vi "Main.vi"() -> ()   [LabVIEW 2015, in "Tool Module.lvlib"]
doc: "This template is based from the Queued Message Handler design pattern and the Queued Message Handler Project Template that ships with LabVIEW 2014.\n\nThe main difference is that the Queue is private to this module and communication between modules is done via Broadcast and Request events.\n\nRequest events are wrapped via public API methods and are handled in the Event handler loop in this VI.\nAny module can register for Broadcast events sent by this module.\n\nThe Event Handling Loop generates messages based on user interface actions.\n\nThe Message Handling Loop processes messages generated by the Event Handling Loop, or by other messages. The messages are string values, so new messages can be added easily to the Message Cases case structure in the Message Handling Loop. Each message cluster can also provide an optional value for Message Data, which is a variant that can be converted to whatever message-specific data is required.\n_____\nBased on Delacor QMH Project Template 2.1.0.2."
uses:
  Tool Module.lvlib
  <vilib>/Delacor/Delacor QMH/Libraries/Module Admin_class/Delacor_lib_QMH_Module Admin.lvclass
  Module Data--cluster.ctl
  Support/_STATUS Typedef--cluster.ctl
  Support/Timer State Return Typedef.ctl
  Support/_Sample Data Rtn Cluster--typedef.ctl
  Support/_Inspection Limits cluster--typedef.ctl
  Event Logger Library/Event Log/EventLog.lvclass
  Return FPGA Setup Data (Reply Payload)--cluster.ctl
  Tool Typedefs/_FPGA Setup Params Cluster--typedef.ctl
  Tool Typedefs/_FPGA Timing Constraints Cluster--typedef.ctl
  Tool Typedefs/_FPGA Timing Ctrl Cluster--typedef.ctl
  Tool Typedefs/_FPGA Laser Config Cluster--typedef.ctl
  Tool Typedefs/_FPGA Peak Proc Cfg Cluster--typedef.ctl
  Tool Typedefs/_FPGA SPI Cfg Cluster--typedef.ctl
  Tool Interface/_Host - HS Data Stream State Enum Typedef.ctl
  _Motion Status Reader SM enum--typedef.ctl
  Tool Typedefs/_Motion STATUS Cluster--typedef.ctl
  Support/_IHL Data Cluster--typedef.ctl
  Support/_IHL SM Enum--typedef.ctl
  Support/_IHL Status Update Cluster--typedef.ctl
  Support/_IHL Status Notifier Data Cluster--typedef.ctl
  Support/_HS Data Stream Params Cluster--typedef.ctl
  Support/_HS Data Stream SM enum--typedef.ctl
  <vilib>/Delacor/Delacor QMH/Libraries/Message Queue_class/Delacor_lib_QMH_Message Queue.lvclass/Delacor_lib_QMH_Message Queue.ctl
  Start Inspect 2 (Reply Payload)--cluster.ctl
  Get All Inspect Data (Reply Payload)--cluster.ctl
  Stop Argument--cluster.ctl
  <vilib>/Delacor/Delacor QMH/Libraries/Module Admin_class/Delacor_lib_QMH_Module Admin.lvclass/Delacor_lib_QMH_Module Admin.ctl
  CONNECT Argument--cluster.ctl
  GOTO Argument--cluster.ctl
  Support/_GoTo Cmd Typedef--enum.ctl
  Get All Inspect Data Argument--cluster.ctl
  Start Data Monitor Argument--cluster.ctl
  Get FPGA Setup Params Argument--cluster.ctl
  Get FPGA Setup Params (Reply Payload)--cluster.ctl
  Set FPGA Setup Params Argument--cluster.ctl
  Commit Tool Config Argument--cluster.ctl
  Tool Config/_Configuration Cluster_v3--typedef.ctl
  Tool Config/_Tool Block Cluster_v3--typedef.ctl
  Tool Config/_Motor Block Cluster_v2--typedef.ctl
  Tool Config/_Verification Blk Cluster--typedef.ctl
  Tool Config/_ProbeConfigParams Cluster--typedef.ctl
  Tool Config/_Sensor Block Cluster--typedef.ctl
  Tool Config/_SensorConfigParams Cluster--typedef.ctl
  Set Integration Count Argument--cluster.ctl
  Set Laser Params Argument--cluster.ctl
  Get Mtrl Ctrl Reg Argument--cluster.ctl
  Get Mtrl Ctrl Reg (Reply Payload)--cluster.ctl
  Commit Ctrl Reg Argument--cluster.ctl
  Set Event Logger Argument--cluster.ctl
  Write to File Argument--cluster.ctl
  Read from File Argument--cluster.ctl
  Set Device Temp Thresholds Argument--cluster.ctl
  Tool Typedefs/_Temperature Threshold Arrays--typedef.ctl
  Get Cycle Count Argument--cluster.ctl
  Get Cycle Count (Reply Payload)--cluster.ctl
  Return FPGA Setup Data Argument--cluster.ctl
  Update FPGA Setup Data Argument--cluster.ctl
  Get-Set Inspection Limits Argument--cluster.ctl
  Get-Set Inspection Limits (Reply Payload)--cluster.ctl
  Support/_Tool Status Update Cluster--typedef.ctl
  Connected Argument--cluster.ctl
  Read from File Rtn Argument--cluster.ctl
  Support/_Cycle Count File Cluster--typedef.ctl
  Tool Typedefs/_Temperature All Arrays--typedef.ctl
  Tool Typedefs/_FPGA Return Setup Data Cluster--typedef.ctl
  Tool Config/_Tool Cfg Return Parameters Cluster--typedef.ctl
  Tool Typedefs/_Data Stream Fmt Params Cluster--typedef.ctl
  <vilib>/Delacor/Delacor QMH/Libraries/Message Queue_class/Delacor_lib_QMH_Enqueue Message (Single).vi
  <vilib>/Delacor/Delacor QMH/Libraries/Module Admin_class/Delacor_lib_QMH_Get External Launch.vi
  <vilib>/Delacor/Delacor QMH/Libraries/Message Queue_class/Delacor_lib_QMH_Enqueue Message (Array).vi
  Tool Interface/GLOB - Configuration Options.vi
  Support/ToolModGLOB.vi
  <vilib>/Utility/error.llb/Error Cluster From Error Code.vi
  <vilib>/ErrorRing/Error Ring.xnode
  <vilib>/Delacor/Delacor QMH/Libraries/Message Queue_class/Delacor_lib_QMH_Message Queue.lvclass
  Collect Data Mgr/Collect Data Mgr.lvlib
  Tool Interface/Tool Interface.lvlib
  Tool Config/Tool Cfg.lvlib
panel:
  in  "Retrieve Cfg":bool
  in  "Cfg File Path":path
  in  "Simulate MHL Error":bool
  in  "Simulate EHL Error":bool
  out "error out":errorcluster
  in  "Module Admin":refnum<class "Delacor_lib_QMH_Module Admin.lvclass">
  out "Status":string
  # "Other QMH Modules communicate with this Module via its Public API (wrappers for its Request Events).\n\nThis Module communicates with other Modules via its Broadcast Events.\nAny module that wants to get these messages, just registers for this module's Broadcast events."
  # "This template is for the Delacor Modified Queued Message Handler design pattern.\n\nSee the block diagram for more information on how to use this template."
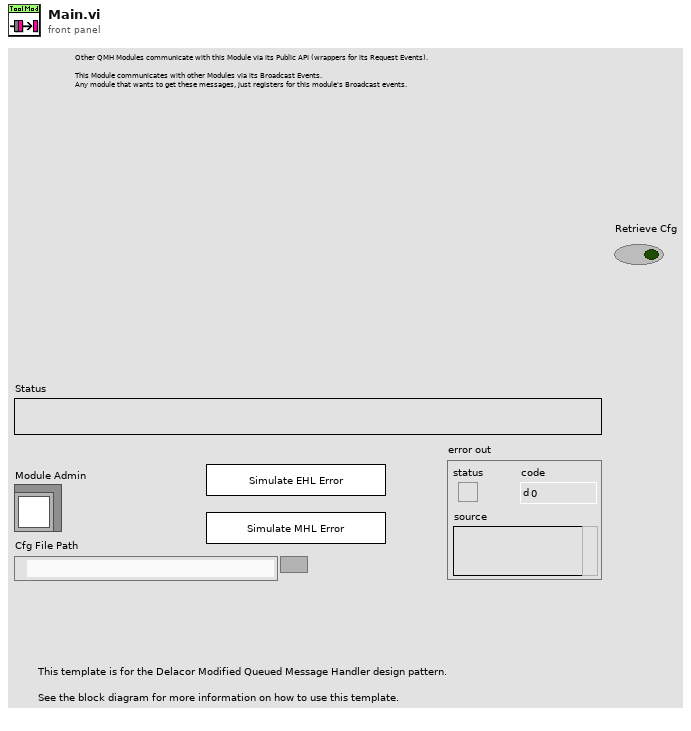
[diagram p1: front panel]
types:
  T1 = typedef "Tool Module.lvlib/_IHL Status Notifier Data Cluster--typedef.ctl" = cluster{"Status":u16, "Encoder":i32}
  T2 = typedef "Tool Module.lvlib/_IHL Data Cluster--typedef.ctl" = cluster{"IHL State":T3, "Timeout":i32, "Loop Count":i32, "Start Sample No.":u32, "Collecting Data":bool, "No. Samples":i32, "Success Flag":bool, "Inspect Status ":T4, "Status":u16, "Encoder Count":i32, "PosToStartScan":i32, "ScanLength":i32, "MaxSamples":i32, "PosToEndScan":i32, "Host SampleData":refnum<notifier>, "data value reference":refnum<data-value>, "Block Cnt notifier out":refnum<notifier>, "EventLog":refnum<class "EventLog.lvclass">}
  T3 = typedef "Tool Module.lvlib/_IHL SM Enum--typedef.ctl" = enum16{"Init", "Set Motion Speed", "Move To Scan Start", "Wait for Motion Out", "Wait for Start Pos", "Inspect: START", "Wait for Motion IN", "Wait for Inspect Range", "Inspecting", "Inspect: STOP"}
  T4 = typedef "Tool Module.lvlib/_IHL Status Update Cluster--typedef.ctl" = cluster{"Ready":bool, "Inspecting":bool, "Cancel":bool}
  T5 = typedef "_Motion STATUS Cluster--typedef.ctl" = cluster{"Encoder":i32, "STATUS":u16, "MC SM State":u16, "M_Ctrl":u16}
  T6 = typedef "Tool Module.lvlib/_Motion Status Reader SM enum--typedef.ctl" = enum16{"Not Connected", "Connect", "Idle", "Receive Data", "Disconnect"}
  T7 = typedef "Tool Module.lvlib/_Host - HS Data Stream State Enum Typedef.ctl" = enum16{"Idle", "Connect", "Receive Data", "Close Connection"}
  T8 = typedef "Tool Module.lvlib/Module Data--cluster.ctl" = cluster{"Status String":string, "STATUS":T9, "Timer 1":T10, "Timer 2":T10, "Timer 1 Call State":string, "Timer 2 Call State":string, "LED State 1":bool, "LED State 2":bool, "OK to Connect":bool, "Connecting":bool, "Got FW Ver":bool, "Got Tool Type":bool, "Got Tool Cfg":bool, "Got Fmt Params":bool, "Got FPGA Setup":bool, "Got Cycle Count":bool, "Cancel Inspect":bool, "Trig State":bool, "Encoder Count":i32, "Loop Counter":i32, "Start Sample No.":u32, "Host SampleData":refnum<notifier>, "Inspection Limits":T11, "EventLog.lvclass":refnum<class "EventLog.lvclass">, "Prev. Encdr":i32, "Status Update Cnt":i32, "Cycle Count":i32, "data value reference":refnum<data-value>, "Final No. of Blks":i32, "CD Success":bool, "FW Ver Maj/Min":dbl, "FPGA Setup Reply Notifier":refnum<notifier>}
  T9 = typedef "Tool Module.lvlib/_STATUS Typedef--cluster.ctl" = cluster{"Initialized":bool, "Connected":bool, "Ready":bool, "Inspecting":bool, "Position":dbl, "Status":u16, "Error":bool, "Code":i32, "MC SM State":u16, "M_Ctrl":u16}
  T10 = typedef "Tool Module.lvlib/Timer State Return Typedef.ctl" = cluster{"Instance Name":string, "On/Off":bool, "Running":bool}
  T11 = typedef "Tool Module.lvlib/_Inspection Limits cluster--typedef.ctl" = cluster{"MaxSamples":i32, "PosToStartScan":i32, "PosToEndScan":i32, "ScanLength":i32}
  T12 = typedef "Tool Module.lvlib/Request Events--cluster.ctl" = cluster{"Stop Module":refnum<user-event>, "Show Panel":refnum<user-event>, "Hide Panel":refnum<user-event>, "Get Module Execution Status":refnum<user-event>, "Show Diagram":refnum<user-event>, "GOTO":refnum<user-event>, "CONNECT":refnum<user-event>, "Get All Inspect Data":refnum<user-event>, "Start Data Monitor":refnum<user-event>, "Get FPGA Setup Params":refnum<user-event>, "Set FPGA Setup Params":refnum<user-event>, "Commit Tool Config":refnum<user-event>, "Set Integration Count":refnum<user-event>, "Set Laser Params":refnum<user-event>, "Get Mtrl Ctrl Reg":refnum<user-event>, "Commit Ctrl Reg":refnum<user-event>, "Set Event Logger":refnum<user-event>, "Write to File":refnum<user-event>, "Read from File":refnum<user-event>, "Set Device Temp Thresholds":refnum<user-event>, "Get Cycle Count":refnum<user-event>, "Return FPGA Setup Data":refnum<user-event>, "Update FPGA Setup Data":refnum<user-event>, "Setup Timer":refnum<user-event>, "Tool Status Reader Cmd":refnum<user-event>, "Stop Helper Loops":refnum<user-event>, "Enable Receive Stream":refnum<user-event>, "Get-Set Inspection Limits":refnum<user-event>, "Start Inspect 2":refnum<user-event>}
  T13 = typedef "Tool Module.lvlib/_Loop Ctrl Notifiers Cluster--typedef.ctl" = cluster{"Raw Stream Ctrl":refnum<notifier>}
  T14 = typedef "Tool Module.lvlib/Broadcast Events--cluster.ctl" = cluster{"Module Did Init":refnum<user-event>, "Status Updated":refnum<user-event>, "Error Reported":refnum<user-event>, "Module Did Stop":refnum<user-event>, "Update Module Execution Status":refnum<user-event>, "Send Status":refnum<user-event>, "Trigger":refnum<user-event>, "Connected":refnum<user-event>, "Read from File Rtn":refnum<user-event>, "Device Temperature":refnum<user-event>, "Time Expired":refnum<user-event>}
  T15 = typedef "Tool Module.lvlib/_HS Data Stream SM enum--typedef.ctl" = enum16{"Idle", "Receive HS Data", "Close Connection"}
  T16 = typedef "Tool Module.lvlib/_HS Data Stream Params Cluster--typedef.ctl" = cluster{"Raw Data Stream Loop cmd":T15, "Data Array DVR ref":refnum<data-value>, "HS Sample Data notifier":refnum<notifier>, "Block Count Notifier":refnum<notifier>}
  T17 = typedef "Tool Module.lvlib/Start Inspect 2 (Reply Payload)--cluster.ctl" = cluster{"Sample Data notifier":refnum<notifier>, "Start Inspect 2_error":errorcluster}
  T18 = typedef "Tool Module.lvlib/Get All Inspect Data (Reply Payload)--cluster.ctl" = cluster{"Success":bool, "Full Inspection Data":u32[][], "data value reference":refnum<data-value>}
  T19 = enum32{"invalid lock state", "Not Locked", "Locked (No Password)", "Password-protected"}
  T20 = typedef "Tool Module.lvlib/Stop Argument--cluster.ctl" = cluster{"Origin":string, "Exit via Stop Module Req?":bool, "Wait for Module to stop?":bool}
  T21 = typedef "Tool Module.lvlib/CONNECT Argument--cluster.ctl" = cluster{"Connect":bool}
  T22 = typedef "Tool Module.lvlib/GOTO Argument--cluster.ctl" = cluster{"GoTo Cmd":T23, "Data":i32}
  T23 = typedef "Tool Module.lvlib/_GoTo Cmd Typedef--enum.ctl" = enum16{"MoveA", "MoveR", "Home Position", "Home None", "Cleaning Position"}
  T24 = typedef "Tool Module.lvlib/Get All Inspect Data Argument--cluster.ctl" = cluster{"dummy":bool, "Wait Notifier":refnum<notifier>}
  T25 = typedef "Tool Module.lvlib/Start Data Monitor Argument--cluster.ctl" = cluster{"Monitor":bool, "Lasers ON?":bool, "Host Sample Data notifier":refnum<notifier>}
  T26 = typedef "Tool Module.lvlib/Get FPGA Setup Params Argument--cluster.ctl" = cluster{"dummy":bool, "Wait Notifier":refnum<notifier>}
  T27 = typedef "Tool Module.lvlib/Set FPGA Setup Params Argument--cluster.ctl" = cluster{"Commit":bool, "FPGA Setup Parameters":T28}
  T28 = typedef "_FPGA Setup Params Cluster--typedef.ctl" = cluster{"FPGA Timing Constraints":T29, "FPGA Timing Ctrl":T30, "FPGA Laser Config":T31, "FPGA Peak Proc Cfg":T32, "FPGA SPI Cfg":T33}
  T29 = typedef "_FPGA Timing Constraints Cluster--typedef.ctl" = cluster{"frame.length Min":u16, "frame.ST_OFF Min":u16, "frame.ST_ON Min":u16, "frame.first data idx":u16, "frame.integ Offset":u16, "frame.integ Delay":u16, "frame.ad_latch Delay":u16, "frame.trig time Max":u32}
  T30 = typedef "_FPGA Timing Ctrl Cluster--typedef.ctl" = cluster{"trig.time":u32, "integ.count 1":u32, "integ.count 2":u32, "encdr.latch ctrl":u32, "pixel.read count":u16, "clock.select":u16, "ad.clock offset":u16, "data.control reg":u16}
  T31 = typedef "_FPGA Laser Config Cluster--typedef.ctl" = cluster{"laser.gain":i16, "laser.threshold Low":u16, "laser.threshold High":u16, "laser.dac init":u16, "laser.dac Min":u16, "laser.dac Max":u16, "laser.config reg":u16}
  T32 = typedef "_FPGA Peak Proc Cfg Cluster--typedef.ctl" = cluster{"PD.threshold":u16, "PD.width detect Min":u8, "PD.sensor pixels":u16, "PD.config reg":u16}
  T33 = typedef "_FPGA SPI Cfg Cluster--typedef.ctl" = cluster{"SPI Divide Value":u8, "SPI config reg":u16}
  T34 = typedef "Tool Module.lvlib/Commit Tool Config Argument--cluster.ctl" = cluster{"Tool Config Cluster":T35}
  T35 = typedef "Tool Cfg.lvlib/_Configuration Cluster_v3--typedef.ctl" = cluster{"Tool Type":u16, "Tool SN":u16, "Tool Block":T36, "Motor Block":T37, "Verification Block":T38, "Probe Block":cluster{"nProbes":u16, "Probe Param Array":T39[]}}
  T36 = typedef "Tool Cfg.lvlib/_Tool Block Cluster_v3--typedef.ctl" = cluster{"Encoder Size":u16, "Encoder Scale":u32, "Encoder Offset":i32, "MaxEncoder":i32, "MinEncoder":i32, "Start Delay":sgl, "Tool Face Ref":sgl}
  T37 = typedef "Tool Cfg.lvlib/_Motor Block Cluster_v2--typedef.ctl" = cluster{"MinMotor Speed":u16, "MaxMotor Speed":u16, "Homing Speed":u16, "Jog Speed":u16, "Inspect Speed":u16, "VBlk Speed":u16, "CleaningPos":i32, "Safe Zone":i32, "Has Motor":bool, "Use Home Index":bool}
  T38 = typedef "Tool Cfg.lvlib/_Verification Blk Cluster--typedef.ctl" = cluster{"Angle":sgl, "FlankLength1":sgl, "FlankLength2":sgl, "Location":sgl, "Serial Number":u16}
  T39 = typedef "Tool Cfg.lvlib/_ProbeConfigParams Cluster--typedef.ctl" = cluster{"Name":string, "Laser Init Pwr":u16, "Laser Gain":u8, "Integ Count":u16, "Meas. Range":sgl, "Angle":sgl, "Probe Offset":sgl, "Sensor Block":T40}
  T40 = typedef "Tool Cfg.lvlib/_Sensor Block Cluster--typedef.ctl" = cluster{"nSensors":u16, "SensorCfgParams Array":T41[]}
  T41 = typedef "Tool Cfg.lvlib/_SensorConfigParams Cluster--typedef.ctl" = cluster{"Total Pixels":u16, "Positive  Peaks":bool, "CalibrCoefArray":dbl[], "Start Idx":u16, "End Idx":u16}
  T42 = typedef "Tool Module.lvlib/Set Integration Count Argument--cluster.ctl" = cluster{"Mode":i16, "Integ Count":u32}
  T43 = typedef "Tool Module.lvlib/Set Laser Params Argument--cluster.ctl" = cluster{"Mode":i16, "Gain":u16, "Init DAC":u16}
  T44 = typedef "Tool Module.lvlib/Get Mtrl Ctrl Reg Argument--cluster.ctl" = cluster{"dummy":bool, "Wait Notifier":refnum<notifier>}
  T45 = typedef "Tool Module.lvlib/Commit Ctrl Reg Argument--cluster.ctl" = cluster{"Ctrl Reg":u16}
  T46 = typedef "Tool Module.lvlib/Set Event Logger Argument--cluster.ctl" = cluster{"EventLog.lvclass":refnum<class "EventLog.lvclass">}
  T47 = typedef "Tool Module.lvlib/Write to File Argument--cluster.ctl" = cluster{"Filename":string, "Flattened data strings":string[]}
  T48 = typedef "Tool Module.lvlib/Read from File Argument--cluster.ctl" = cluster{"Filename":string, "Create?":bool, "Flattened Data Strings":string[]}
  T49 = typedef "Tool Module.lvlib/Set Device Temp Thresholds Argument--cluster.ctl" = cluster{"Device Temp Thold Arrays":T50}
  T50 = typedef "_Temperature Threshold Arrays--typedef.ctl" = cluster{"High Thold ":dbl[], "Low Thold ":dbl[]}
  T51 = typedef "Tool Module.lvlib/Get Cycle Count Argument--cluster.ctl" = cluster{"Clear?":bool, "Wait Notifier":refnum<notifier>}
  T52 = typedef "Tool Module.lvlib/Return FPGA Setup Data Argument--cluster.ctl" = cluster{"Reload":bool, "Wait Notifier":refnum<notifier>, "wait for reply":bool}
  T53 = typedef "Tool Module.lvlib/Update FPGA Setup Data Argument--cluster.ctl" = cluster{"Commit":bool, "FPGA Setup Parameters":T28}
  T54 = typedef "Tool Module.lvlib/Get-Set Inspection Limits Argument--cluster.ctl" = cluster{"Set":bool, "Inspection Limits":T11, "Wait Notifier":refnum<notifier>, "wait for reply":bool}
  T55 = enum32{"Invalid", "Standard", "Closed", "Hidden", "Minimized", "Maximized"}
  T56 = typedef "Tool Module.lvlib/_Tool Status Update Cluster--typedef.ctl" = cluster{"Tool Status":T5, "Reader SM State":T6}
  T57 = cluster{"TE_Running":bool, "PD_Running":bool, "Laser On 1":bool, "Laser On 2":bool}
  T58 = typedef "Tool Module.lvlib/Connected Argument--cluster.ctl" = cluster{"Connected":bool, "Tool Type":u16, "Tool SN":u16}
  T59 = typedef "Tool Module.lvlib/Get Mtrl Ctrl Reg (Reply Payload)--cluster.ctl" = cluster{"Mtr Ctrl Reg":u16, "Get Mtrl Ctrl Reg_error":errorcluster}
  T60 = typedef "Tool Module.lvlib/Get-Set Inspection Limits (Reply Payload)--cluster.ctl" = cluster{"Inspection Limits":T11, "Get-Set Inspection Limits_error":errorcluster}
  T61 = typedef "Tool Module.lvlib/Get FPGA Setup Params (Reply Payload)--cluster.ctl" = cluster{"Version String":string, "FPGA Setup Parameters":T28}
  T62 = typedef "Tool Module.lvlib/Read from File Rtn Argument--cluster.ctl" = cluster{"Filename":string, "XML Strings":string[], "Error Status":errorcluster}
  T63 = typedef "Tool Module.lvlib/_Cycle Count File Cluster--typedef.ctl" = cluster{"Cycle Count":i32}
  T64 = cluster{"Filename":string, "XML Strings":string, "Error Status":errorcluster}
  T65 = typedef "_Temperature All Arrays--typedef.ctl" = cluster{"Temp Sensors":dbl[], "High Thold ":dbl[], "Low Thold ":dbl[]}
  T66 = typedef "Tool Module.lvlib/Get Cycle Count (Reply Payload)--cluster.ctl" = cluster{"Cycle Count":i32, "Get Cycle Count_error":errorcluster}
  T67 = typedef "Tool Module.lvlib/Return FPGA Setup Data (Reply Payload)--cluster.ctl" = cluster{"Version String":string, "FPGA Setup Parameters":T28, "Return FPGA Setup Data_error":errorcluster}
  T68 = typedef "_FPGA Return Setup Data Cluster--typedef.ctl" = cluster{"Version String":string, "Mtr Ctrl Reg":u16, "FPGA Setup Parameters":T28}
  T69 = typedef "Tool Cfg.lvlib/_Tool Cfg Return Parameters Cluster--typedef.ctl" = cluster{"Config Cluster Version":string, "Product Name":string, "Tool Config Cluster":T35}
  T70 = typedef "_Data Stream Fmt Params Cluster--typedef.ctl" = cluster{"Samples per Block":i32, "Raw Data Status Len":i32, "Fltr Data Status Len":i32}
  T71 = typedef "Tool Module.lvlib/_Sample Data Rtn Cluster--typedef.ctl" = cluster{"Inspecting":bool, "Acquiring Data":bool, "Success":bool, "Cancelled":bool, "Scan Data Array":u32[], "error cluster":errorcluster}
  T72 = typedef "Tool Cfg.lvlib/_Tool Operation Config Cluster--typedef.ctl" = cluster{"Use Tool Cfg":bool, "Use Tool Cal":bool, "Fake Data?":bool, "Mode":i16, "Array Subset Length":i16, "nArrays to Read":i16, "Full Array Read Length":i16, "nSubarrays/Sensor":i16}
  T73 = typedef "Collect Data Mgr.lvlib/Start Collect (Reply Payload)--cluster.ctl" = cluster{"Success":bool, "CD_Status":u8}
  T74 = typedef "Tool Module.lvlib/_Data Notifiers Cluster--typedef.ctl" = cluster{"Sample Data":refnum<notifier>}
  T75 = cluster{"Tool Status Cluster":T5, "Tool Status Reader State":T6}
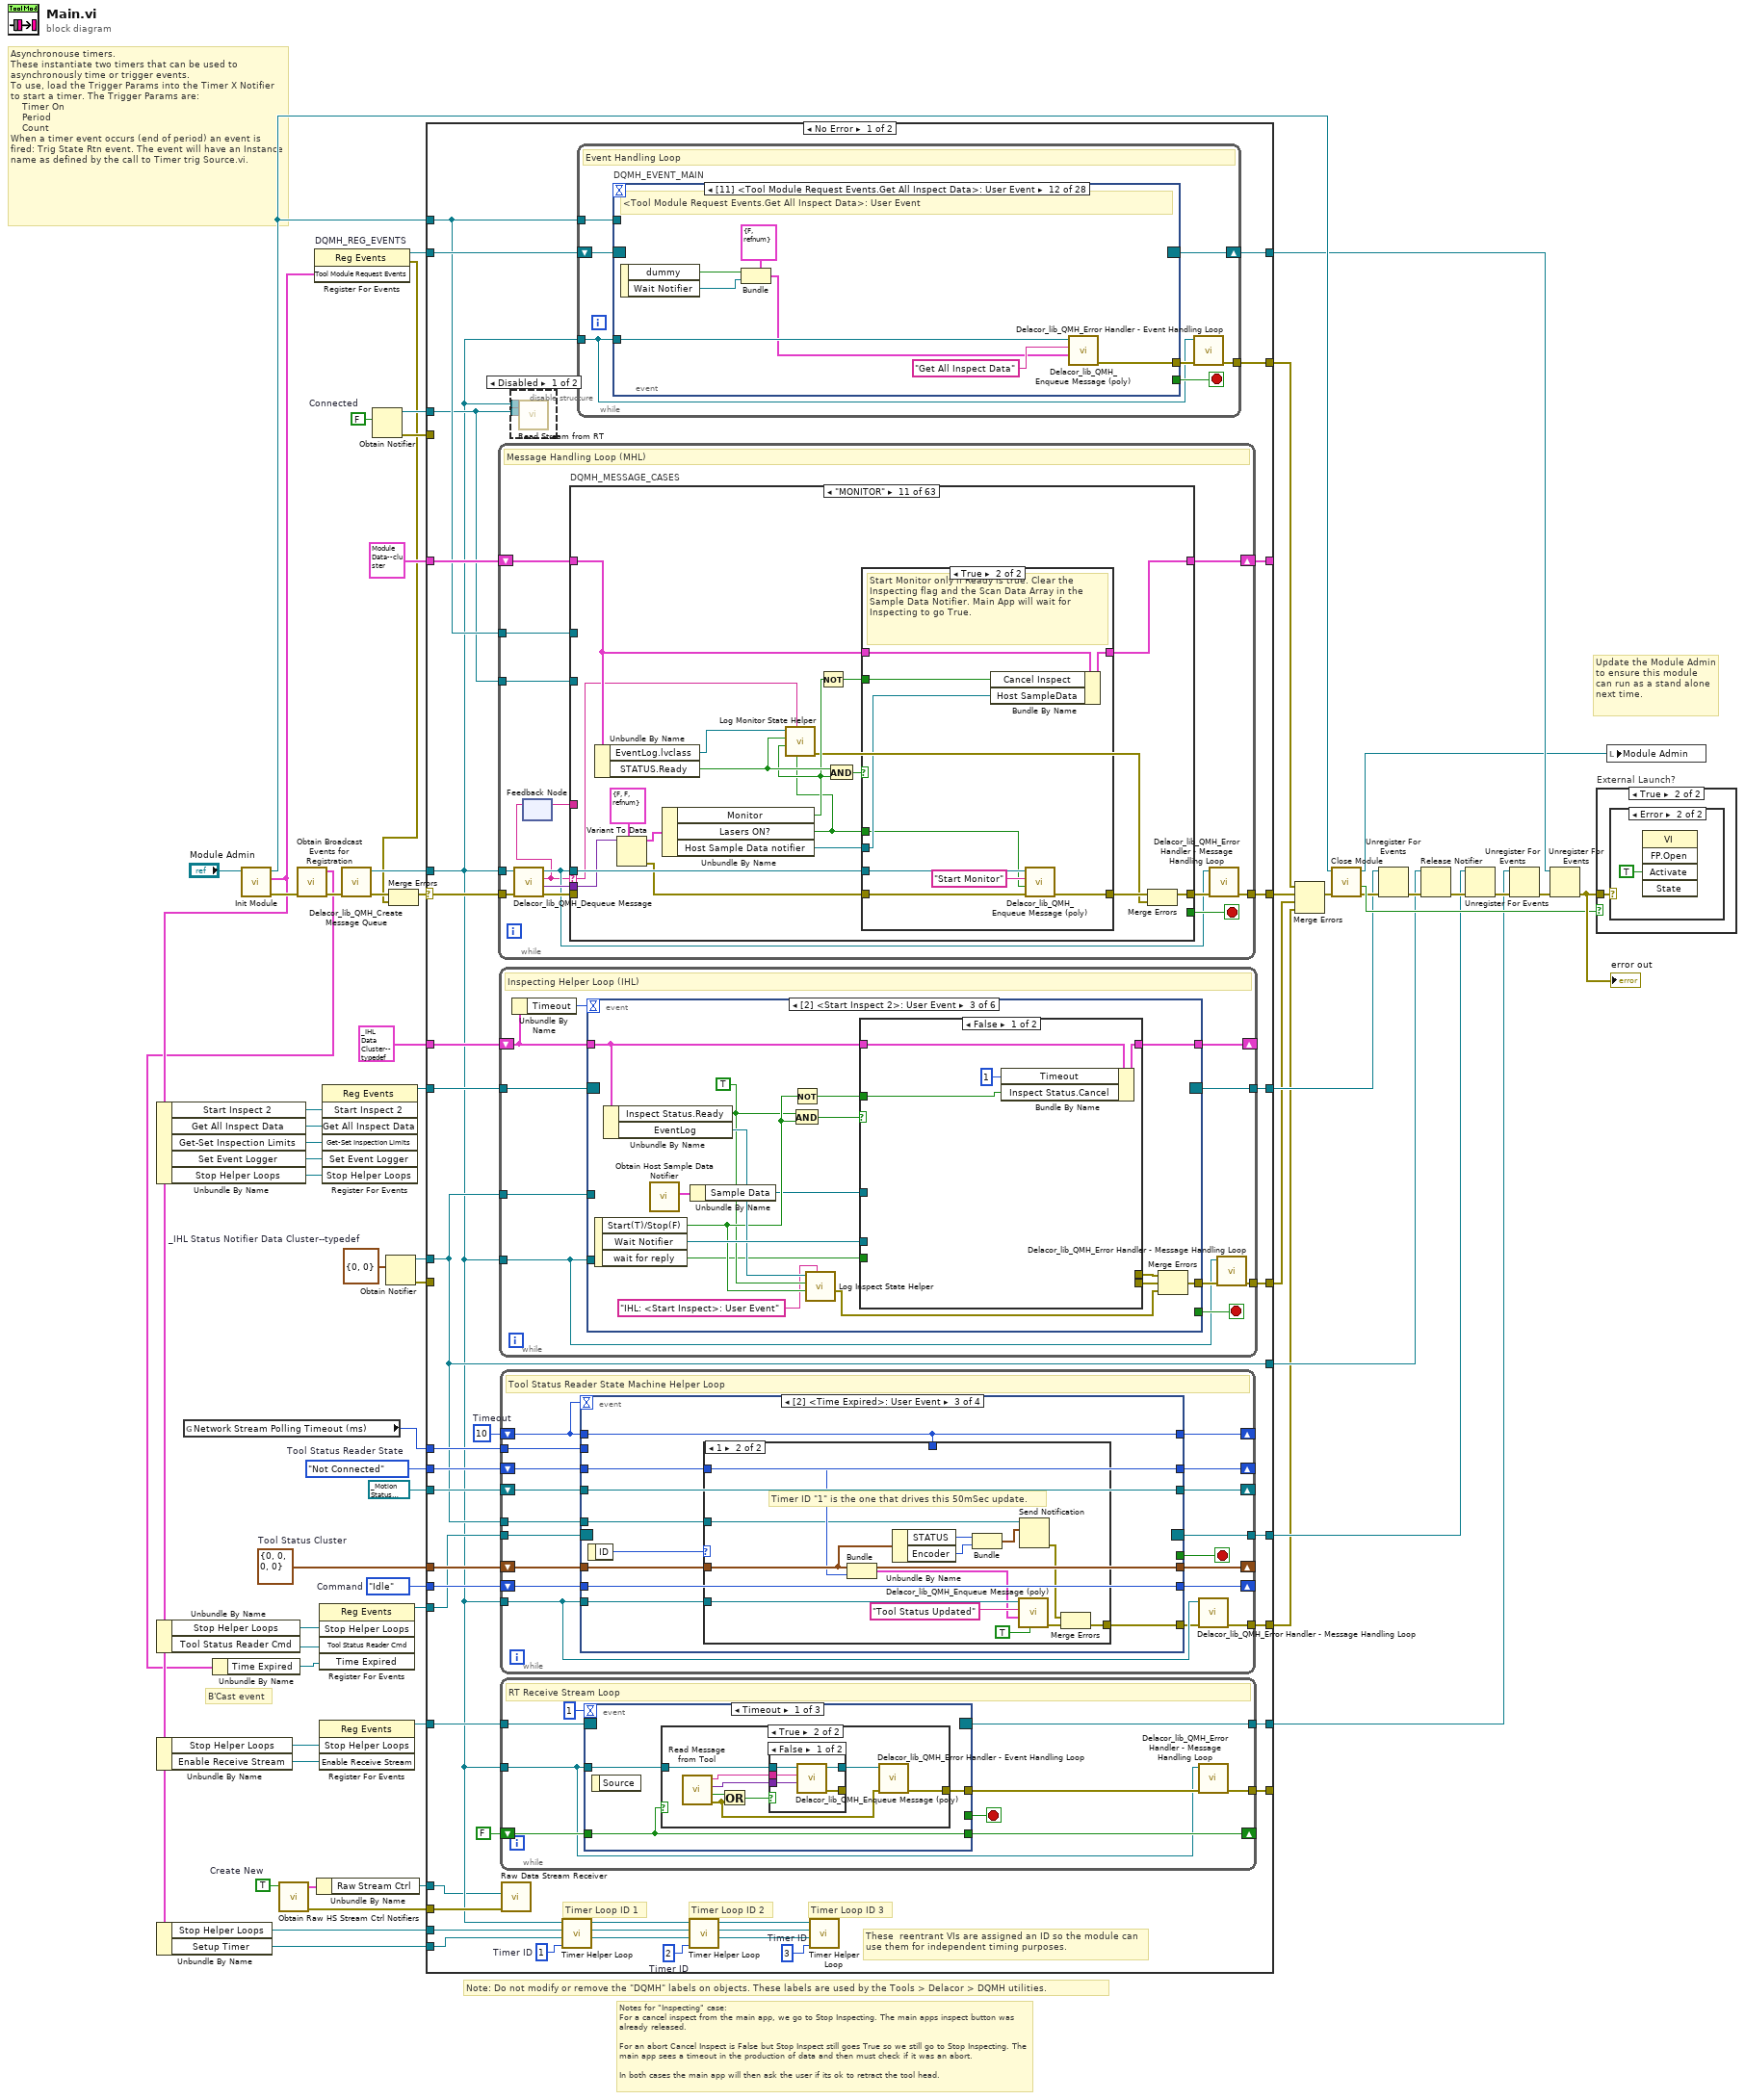
[diagram p0: block diagram]
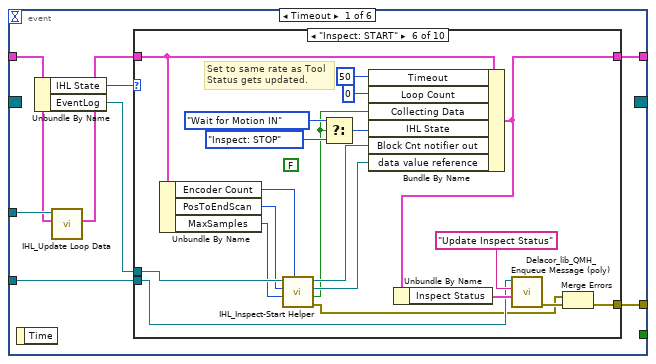
[diagram p2: hidden frame]
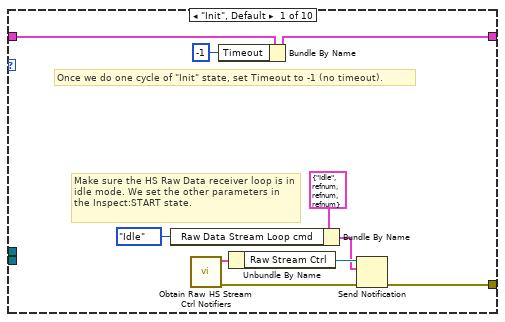
[diagram p3: hidden frame]
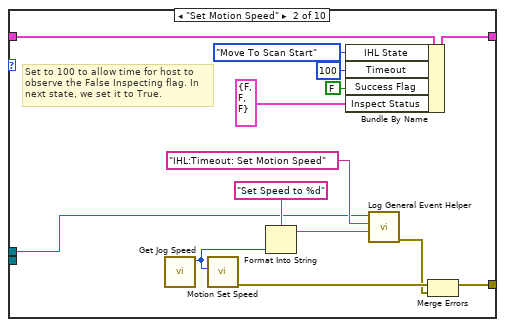
[diagram p4: hidden frame]
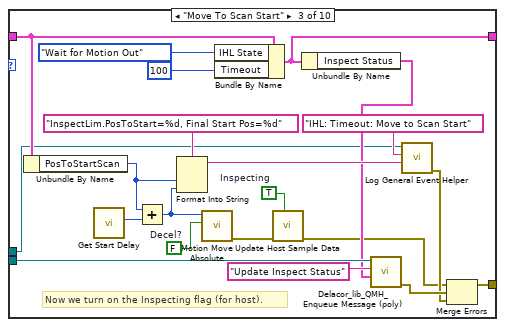
[diagram p5: hidden frame]
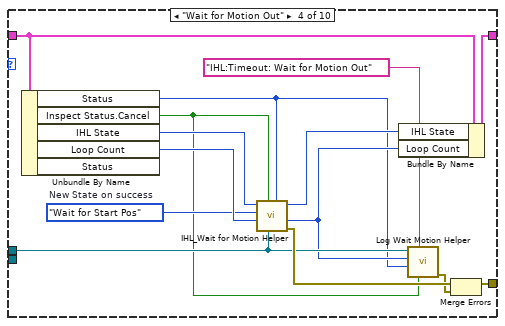
[diagram p6: hidden frame]
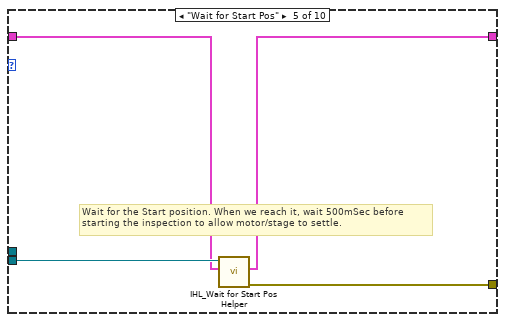
[diagram p7: hidden frame]
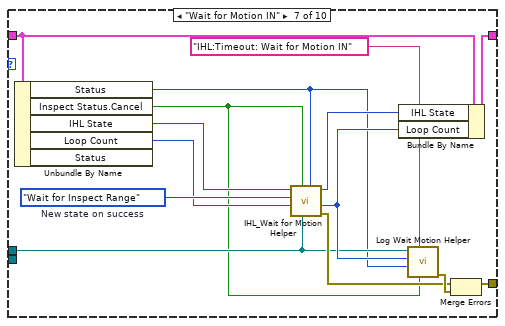
[diagram p8: hidden frame]
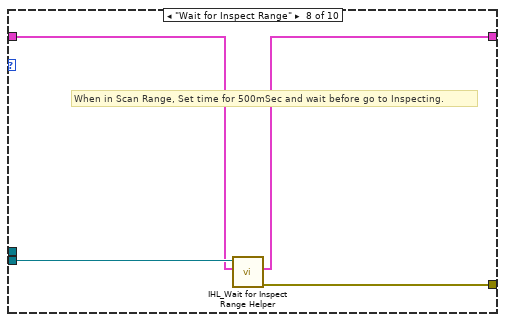
[diagram p9: hidden frame]
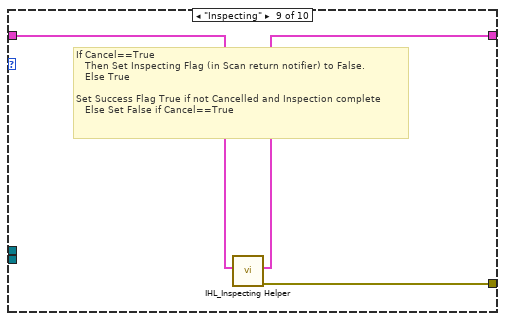
[diagram p10: hidden frame]
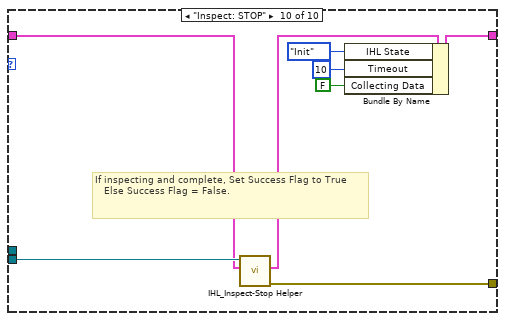
[diagram p11: hidden frame]
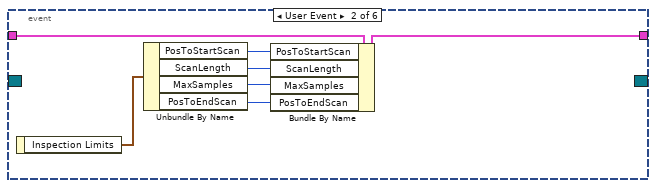
[diagram p12: hidden frame]
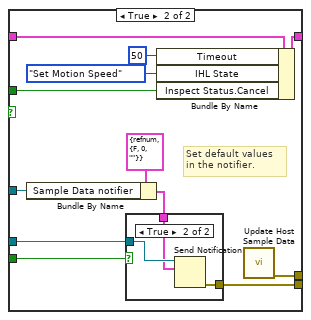
[diagram p13: hidden frame]
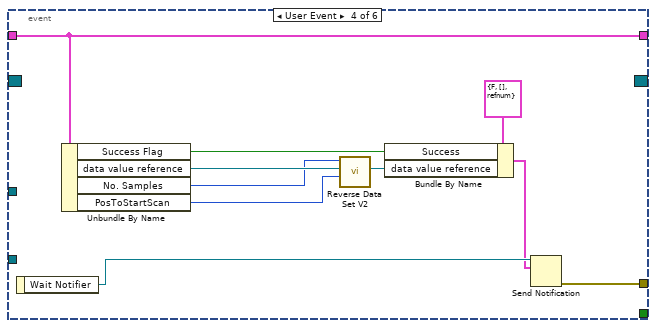
[diagram p15: hidden frame]
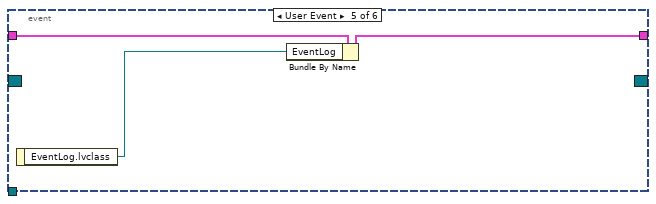
[diagram p16: hidden frame]
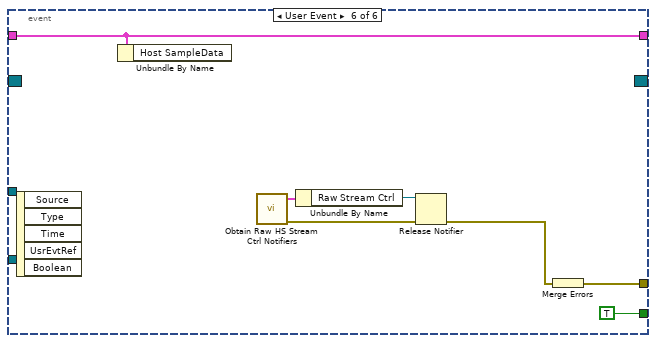
[diagram p17: hidden frame]
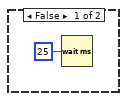
[diagram p18: hidden frame]
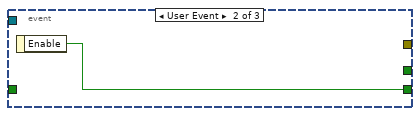
[diagram p20: hidden frame]
diagram:
  w5 = TRUE  # Create New
  w12 = T1 {"Status"=0, "Encoder"=0}  # _IHL Status Notifier Data Cluster--typedef
  w31 = T5 {"Encoder"=0, "STATUS"=0, "MC SM State"=0, "M_Ctrl"=0}  # Tool Status Cluster
  w36 = _Motion_Status_Reader_SM_enum--typedef."Not Connected"  # Tool Status Reader State
  w35 = _Host_-_HS_Data_Stream_State_Enum_Typedef."Idle"  # Command
  w46 = FALSE  # Connected
  # "B'Cast event"
  # "Notes for \"Inspecting\" case:\nFor a cancel inspect from the main app, we go to Stop Inspecting. The main apps inspect button was already released. \n\nFor an abort Cancel Inspect is False but Stop Inspect still goes True so we still go to Stop Inspecting. The main app sees a timeout in the production of data and then must check if it was an abort.\n\nIn both cases the main app will then ask the user if its ok to retract the tool head."
  # "Asynchronouse timers.\nThese instantiate two timers that can be used to asynchronously time or trigger events.\nTo use, load the Trigger Params into the Timer X Notifier to start a timer. The Trigger Params are:\n    Timer On\n    Period\n    Count\nWhen a timer event occurs (end of period) an event is fired: Trig State Rtn event. The event will have an Instance name as defined by the call to Timer trig Source.vi."
  # "Note: Do not modify or remove the \"DQMH\" labels on objects. These labels are used by the Tools > Delacor > DQMH utilities."
  # "Update the Module Admin to ensure this module can run as a stand alone next time."
  n1 = global read "GLOB - Configuration Options.vi" "Network Stream Polling Timeout (ms)"() -> (w34:i32)
  n2 = call "Init Module.vi"("Singleton Module Admin in"="Module Admin") -> ("error out"=w60:errorcluster, "Tool Module Request Events"=w22:T12, "Singleton Module Admin out"=w58:refnum<class "Delacor_lib_QMH_Module Admin.lvclass">)  [unwired: 8 in]
  n3 = Unbundle By Name(w22) -> ("Start Inspect 2"=w21:refnum<user-event>, "Get All Inspect Data"=w20:refnum<user-event>, "Get-Set Inspection Limits"=w19:refnum<user-event>, "Set Event Logger"=w15:refnum<user-event>, "Stop Helper Loops"=w14:refnum<user-event>)
  n4 = Unbundle By Name(w22) -> ("Stop Helper Loops"=w39:refnum<user-event>, "Tool Status Reader Cmd"=w37:refnum<user-event>)
  n5 = Unbundle By Name(w22) -> ("Stop Helper Loops"=w30:refnum<user-event>, "Enable Receive Stream"=w29:refnum<user-event>)
  n6 = Unbundle By Name(w22) -> ("Stop Helper Loops"=w41:refnum<user-event>, "Setup Timer"=w40:refnum<user-event>)
  n7 = call "Obtain Raw HS Stream Ctrl Notifiers.vi"("Create New"=w5) -> ("error out"=w6:errorcluster, "Loop Ctrl Notifiers Cluster"=w4:T13)  [unwired: 9 in]
  n8 = call "Obtain Broadcast Events for Registration.vi"("error in (no error)"=w60) -> ("error out"=w18:errorcluster, "Tool Module Broadcast Events"=w17:T14)  [unwired: 8 in, 1 out]
  n9 = Unbundle By Name(w17) -> ("Time Expired"=w24:refnum<user-event>)
  n10 = register-events "DQMH_REG_EVENTS"(w22) -> (reference out=w55:refnum<event-registration>, error out=w42:errorcluster)  [unwired: 2 in]
  n11 = Unbundle By Name(w4) -> ("Raw Stream Ctrl"=w3:refnum<notifier>)
  n12 = register-events(w39, w37, w24) -> (reference out=w38:refnum<event-registration>)  [unwired: 2 in, 1 out]
  n13 = register-events(w30, w29) -> (reference out=w28:refnum<event-registration>)  [unwired: 2 in, 1 out]
  n14 = register-events(w21, w20, w19, w15, w14) -> (reference out=w23:refnum<event-registration>)  [unwired: 2 in, 1 out]
  n15 = call <vilib>:"Delacor_lib_QMH_Create Message Queue.vi"("error in (no error)"=w18) -> ("error out"=w48:errorcluster, "Message Queue"=w54:refnum<class "Delacor_lib_QMH_Message Queue.lvclass">)  [unwired: 9 in]
  n16 = Obtain Notifier(notification data type=w46) -> (notifier out=w45:refnum<notifier>, error out=w44:errorcluster)  [unwired: 3 in, 1 out]
  n17 = Obtain Notifier(notification data type=w12) -> (notifier out=w13:refnum<notifier>, error out=w11:errorcluster)  [unwired: 3 in, 1 out]
  n18 = Merge Errors(w48, w42) -> (w43:errorcluster)
  n19 = case shown="No Error" w43 {
    selector: w43 -> [w89 w1939]
    tunnel: [w93 w1939] -> w57
    tunnel: [w92 w1944] -> w56
    tunnel: w55 -> [w91 w1944]
    tunnel: w54 -> [w64 _]
    tunnel: [w90 _] -> w47
    tunnel: w58 -> [w88 w1940]
    tunnel: T8 {"Status String"="", "STATUS"={"Initialized"=FALSE, "Connected"=FALSE, "Ready"=FALSE, "Inspecting"=FALSE, "Position"=0.0, "Status"=0, "Error"=FALSE, "Code"=0, "MC SM State"=0, "M_Ctrl"=0}, "Timer 1"={"Instance Name"="", "On/Off"=FALSE, "Running"=FALSE}, "Timer 2"={"Instance Name"="", "On/Off"=FALSE, "Running"=FALSE}, "Timer 1 Call State"="", "Timer 2 Call State"="", "LED State 1"=FALSE, "LED State 2"=FALSE, "OK to Connect"=FALSE, "Connecting"=FALSE, "Got FW Ver"=FALSE, "Got Tool Type"=FALSE, "Got Tool Cfg"=FALSE, "Got Fmt Params"=FALSE, "Got FPGA Setup"=FALSE, "Got Cycle Count"=FALSE, "Cancel Inspect"=FALSE, "Trig State"=FALSE, "Encoder Count"=0, "Loop Counter"=0, "Start Sample No."=0, "Host SampleData"=refnum, "Inspection Limits"={"MaxSamples"=0, "PosToStartScan"=0, "PosToEndScan"=0, "ScanLength"=0}, "EventLog.lvclass"=refnum, "Prev. Encdr"=0, "Status Update Cnt"=0, "Cycle Count"=0, "data value reference"=refnum, "Final No. of Blks"=0, "CD Success"=FALSE, "FW Ver Maj/Min"=0.0, "FPGA Setup Reply Notifier"=refnum} ("Data Cluster") -> [w94 _]
    tunnel: w45 -> [w87 _]
    tunnel: w44 -> [_ _]
    tunnel: [w86 _] -> _
    tunnel: w41 -> [w77 _]
    tunnel: w40 -> [w76 _]
    tunnel: w38 -> [w85 w1936]
    tunnel: w36 -> [w84 _]
    tunnel: w35 -> [w96 _]
    tunnel: w34 -> [w83 _]
    tunnel: refnum<k21> refnum ("reader endpoint") -> [w82 _]
    tunnel: w31 -> [w95 _]
    tunnel: [w81 _] -> w2
    tunnel: [w80 w1936] -> w32
    tunnel: w28 -> [w73 w1935]
    tunnel: [w71 _] -> _
    tunnel: [w70 w1935] -> w25
    tunnel: w23 -> [w69 w1934]
    tunnel: T2 {"IHL State"=enum."Init", "Timeout"=10, "Loop Count"=0, "Start Sample No."=0, "Collecting Data"=FALSE, "No. Samples"=0, "Success Flag"=FALSE, "Inspect Status "={"Ready"=FALSE, "Inspecting"=FALSE, "Cancel"=FALSE}, "Status"=0, "Encoder Count"=0, "PosToStartScan"=50800, "ScanLength"=50800, "MaxSamples"=50800, "PosToEndScan"=0, "Host SampleData"=refnum, "data value reference"=refnum, "Block Cnt notifier out"=refnum, "EventLog"=refnum} ("_Inspect Helper Loop Data Cluster--typedef") -> [w68 _]
    tunnel: w13 -> [w66 w1933]
    tunnel: w11 -> [_ _]
    tunnel: [w67 w1934] -> w9
    tunnel: [w66 w1933] -> w7
    tunnel: w6 -> [w65 _]
    tunnel: w3 -> [w63 _]
    tunnel: [w62 _] -> w1
    frame No Error {
      w74 = 10  # Timeout
      w75 = 3  # Timer ID
      w78 = 2  # Timer ID
      w79 = 1  # Timer ID
      # "These  reentrant VIs are assigned an ID so the module can use them for independent timing purposes."
      # "Timer Loop ID 3"
      # "Timer Loop ID 2"
      # "Timer Loop ID 1"
      n20 = while {
        tunnel: w64 -> [w523]
        shift-right: [w528] -> w86
        shift-left: w94 -> [w529]
        tunnel: w89 -> [w526]
        tunnel: [w521] -> w93
        tunnel: w88 -> [w520]
        tunnel: w87 -> [w519]
        stop <- w527 stop-if-true
        # "Message Handling Loop (MHL)"
        n21 = call-dynamic "Delacor_lib_QMH_Dequeue Message.vi"("error in (no error)"=w526, "Message Queue in"=w523) -> ("error out"=w525:errorcluster, "Message Data"=w524:variant, "Message"=w518:string, "Message Queue out"=w522:refnum<class "Delacor_lib_QMH_Message Queue.lvclass">)  [unwired: 6 in]
        n22 = feedback-in #1(w518) -> ()
        n23 = feedback #1() -> (w517:string)  [unwired: 1 in]
        n24 = case "DQMH_MESSAGE_CASES" shown="\"MONITOR\"" w518 {
          selector: w518 -> [_ _ _ w597 w608 w645 w661 _ w677 w769 w837 _ _ _ _ _ _ _ _ _ w1016 _ _ _ _ _ _ _ _ _ _ _ w1200 w1204 w1229 w1252 w1269 w1318 w1344 w1363 w1392 w1414 w1449 w1470 w1487 w1516 w1543 w1564 _ _ w1650 w1661 w1675 _ _ _ _ _ w1756 w1780 _ _ _]
          tunnel: w522 -> [w552 _ _ _ _ _ _ _ w696 w781 w853 _ _ _ _ _ _ _ w969 w997 _ _ _ _ _ _ _ w1104 _ _ _ _ _ w1217 _ w1256 w1287 _ w1357 _ w1401 w1430 w1462 _ w1507 _ _ w1585 w1618 w1636 w1653 w1670 w1681 _ _ _ w1731 w1746 w1771 _ _ _ _]
          tunnel: w525 -> [w541 w558 w563 w596 _ _ _ w675 _ w780 _ w878 w887 w904 w923 _ w945 w949 w982 w1005 _ w1041 w1072 w1082 w1087 _ w1101 w1118 w1143 _ _ w1186 w1189 _ _ w1258 _ _ _ _ _ _ w1463 _ w1506 w1537 w1555 _ w1616 w1639 w1652 w1669 w1680 w1710 w1713 w1718 w1737 w1750 w1770 _ w1792 w1794 w1796]
          tunnel: [w532 w559 w561 w596 w628 w647 w664 w673 w687 w776 w842 w872 w882 w896 w913 w928 w940 w946 w970 w998 w1018 w1037 w1068 w1081 w1086 w1088 w1097 w1111 w1137 w1153 w1167 w1184 w1203 w1209 w1234 w1250 w1278 w1326 w1352 w1381 w1398 w1428 w1461 w1473 w1504 w1535 w1545 w1586 w1619 w1637 w1659 w1666 w1682 w1708 w1711 w1716 w1728 w1748 w1767 w1781 w1792 w1794 w1796] -> w530
          tunnel: w529 -> [w540 w560 w562 w580 w635 w644 w663 w674 w690 w771 w848 w869 w880 w889 w918 w931 w937 w947 w972 w993 w1017 w1034 w1073 w1077 w1085 w1091 w1094 w1106 w1133 w1162 w1166 w1185 w1202 w1210 w1233 w1259 w1285 w1327 w1350 w1380 w1393 w1424 w1458 w1475 w1492 w1532 w1558 w1573 w1605 w1630 w1656 w1665 w1677 w1709 w1712 w1717 w1736 w1749 w1759 w1782 w1791 w1793 w1795]
          tunnel: [w539 w560 w562 w575 w629 w652 w663 w674 w685 w773 w847 w869 w880 w888 w918 w931 w937 w947 w972 w993 w1017 w1033 w1073 w1076 w1085 w1091 w1094 w1107 w1127 w1162 w1166 w1185 w1202 w1213 w1233 w1259 w1279 w1327 w1353 w1380 w1393 w1425 w1458 w1482 w1493 w1538 w1557 w1580 w1615 w1634 w1658 w1665 w1677 w1709 w1712 w1717 w1736 w1749 w1759 w1782 w1791 w1793 w1795] -> w528
          tunnel: [_ _ _ _ _ _ _ _ _ _ _ _ _ _ _ _ _ _ _ _ _ _ _ _ _ _ _ _ _ _ _ _ _ _ _ _ _ _ _ _ _ _ _ _ _ _ _ _ _ _ _ _ _ _ _ _ _ _ w1768 _ _ _ _] -> w527
          tunnel: w524 -> [_ w557 _ _ w615 w654 w672 _ w692 w779 w852 w877 w885 w902 w922 w934 w944 w948 w981 w1004 w1015 w1042 w1074 w1080 _ w1093 w1100 w1116 w1142 w1160 w1174 _ _ w1216 w1237 _ w1277 w1329 w1356 _ w1400 w1429 _ _ _ _ _ w1576 _ _ _ _ _ _ _ _ w1735 _ w1766 _ _ _ _]
          tunnel: w520 -> [w542 _ _ _ _ _ _ _ _ _ _ _ _ _ _ _ _ _ _ _ _ _ _ _ _ _ _ _ _ _ _ _ _ _ _ _ _ _ _ _ _ _ _ _ _ _ _ _ _ _ _ _ _ _ _ _ w1730 _ w1760 _ _ _ _]
          tunnel: w519 -> [_ _ _ _ _ _ _ _ w686 _ _ _ _ _ _ _ _ _ _ _ _ _ _ _ _ _ _ _ _ _ _ _ _ _ _ _ _ _ _ _ _ _ _ _ _ _ _ _ _ _ _ _ _ _ _ _ _ _ w1772 _ _ _ _]
          tunnel: w517 -> [_ _ _ _ _ _ _ _ _ _ _ _ _ _ _ _ _ _ _ _ _ _ _ _ _ _ _ _ _ _ _ _ _ _ _ _ _ _ _ _ _ _ _ _ _ _ _ _ _ _ _ _ _ _ _ _ w1726 _ _ _ _ _ _]
          frame "Initialize" {
            w538 = "Initial Message" ("Initial Message")
            # "#CodeNeeded - Initialize the appearance of the front panel."
            # "#CodeNeeded - Initialize your state data here."
            # "Initialize - Any operation that needs to be done before the module can receive messages. Synchronize Caller Events.vi will inform Start Module.vi that the module has launched and is ready to receive messages. Module Did Init.vi will broadcast that the module initialized."
            n25 = call "Synchronize Caller Events.vi"("error in (no error)"=w541, "Singleton Module Admin in"=w542) -> ("error out"=w534:errorcluster, "Singleton Module Admin out"=w535:refnum<class "Delacor_lib_QMH_Module Admin.lvclass">)  [unwired: 8 in]
            n26 = property on="Property Node" class="Module Admin"(reference=w535) -> ("Accessors:External Launch"=w546:bool)  [unwired: 1 in, 2 out]
            n27 = Select(t=T55."Hidden" ("State"), s=w546, f=T55."Standard" ("State")) -> (s? t:f=w543:T55)
            n28 = call-poly <vilib>:"Delacor_lib_QMH_Enqueue Message (poly).vi"("error in (no error)"=w534, "Message"="Init Tool", "Message Queue in"=w552) -> ("error out"=w533:errorcluster)  [unwired: 7 in, 1 out]
            n29 = call "Module Name--constant.vi"() -> ("Module Name"=w551:string)  [unwired: 11 in]
            n30 = property on="Property Node" class="VI"("Front Panel.Title"=w551) -> (reference out=w549:refnum<vi>, error out=w550:errorcluster)  [unwired: 2 in]
            n31 = call "Module Name--constant.vi"() -> ("Module Name"=w536:string)  [unwired: 11 in]
            n32 = invoke on="Invoke Node" class="VI" method="FP.Open"(reference=w549, error in=w550, "State"=w543) -> (reference out=w548:refnum<vi>, error out=w547:errorcluster)  [unwired: 2 in, 3 out]
            n33 = call "Module Did Init.vi"("error in (no error)"=w533, "Initialized?"=TRUE, "Origin"=w536) -> ("error out"=w532:errorcluster)  [unwired: 8 in]
            n34 = Bundle By Name(cluster=w540, "Status String"=w538) -> (w539:T8)
            n35 = local write "Status"(w538) -> ()
            n36 = invoke on="Invoke Node" class="VI" method="FP.Center"(reference=w548, error in=w547) -> ()  [unwired: 1 in, 3 out]
          }
          frame "Update Display" {
            # "Broadcast updated status to any VI registered to listen to this module's broadcast events."
            # "Convert the message data to a string to display in the Status indicator."
            # "#CodeRecommended - If you wish to decouple the Message Handling Loop from your user interface, consider creating User Events (like the \"Stop\" event in this VI) to message the Event Handling Loop whenever the user interface needs updating."
            # "Update Display - Update user interface here."
            n37 = Variant To Data(error in=w558, type="", Variant=w557) -> (data=w555:string, error out=w554:errorcluster)
            "Status" <- w555
            n38 = call "Status Updated.vi"("error in (no error)"=w554, "Status"=w555) -> ("error out"=w553:errorcluster)  [unwired: 9 in]
            n39 = Merge Errors(w553) -> (w559:errorcluster)
          }
          frame "------- Module Specific -------" {
            # "Separator -- The following cases handle messages specific to this Module."
            n40 = Merge Errors(w563) -> (w561:errorcluster)
          }
          frame "Init Tool" {
            w568 = TRUE  # Create New?
            w577 = FALSE ("Error")
            w586 = 1 items=["no exception", "cancel error on match", "set error on match"] ("[exception action] (none:0)")
            w576 = FALSE ("STATUS.Connected")
            # "Note: EventLog.lvclass has not been initialized yet!"
            # "Start asynchronous timer for 50ms period, run forever (Count = -1)."
            # "Read in the QC-X Tool Cfg.xml file, which sets up the ToolMgrGLOB tool config and Operation Config clusters.\nAsynchronous timer will fire status event to main app regularly. Note that the cfg file path is passed in when this VI is called to run by the Start Module.vi."
            n41 = global read "ToolModGLOB.vi" "Tool Config Filename"() -> (w594:string)
            n42 = call "Setup Timer.vi"("Enqueue Next State"=FALSE, "Timer ID"=1, "Count"=-1, "Period"=50, "Timer On"=TRUE) -> ("error out"=w566:errorcluster)  [unwired: 6 in]
            n43 = Unbundle By Name(w580) -> ("STATUS"=w579:T9, "EventLog.lvclass"=w564:refnum<class "EventLog.lvclass">)
            n44 = disable-structure shown="Enabled" {
              disable-tunnel: w594 -> [w601 _]
              disable-tunnel: [w600 w604] -> w593
              disable-tunnel: [w599 w603] -> w592
              disable-tunnel: "Cfg File Path" -> [w598 w605]
              frame Disabled {
                n45 = Build Path(base path=w598, name or relative path=w601) -> (appended path=w602:path)
                n46 = call "READ Config from XML file.vi"("Path"=w602) -> ("error out"=w600:errorcluster, "Found"=w599:bool)  [unwired: 7 in, 2 out]
              }
              frame Enabled {
                n47 = call "Read OpCfg from GXML File.vi"("Path"=w605) -> ("error out"=w604:errorcluster, "Found"=w603:bool)  [unwired: 8 in, 1 out]
              }
            }
            n48 = call "IHL_HS Stream Sample Data Notifier.vi"("error in (no error)"=w566, "Create New?"=w568) -> ("error out"=w567:errorcluster)  [unwired: 8 in, 1 out]
            n49 = call "Format Boolean Descriptor.vi"("Descriptor"="Tool Cfg File OK?", "selector"=w592) -> ("resulting string"=w581:string)  [unwired: 6 in]
            n50 = call "Obtain Host Sample Data Notifier.vi"("error in (no error)"=w567, "Create New?"=w568) -> ("error out"=w565:errorcluster)  [unwired: 8 in, 1 out]
            n51 = call "Log General Event Helper.vi"("Payload"=w581, "State Info"=w597, "EventLog in"=w564) -> ("error out"=w583:errorcluster, "EventLog out"=w582:refnum<class "EventLog.lvclass">)  [unwired: 7 in]
            n52 = Bundle By Name(cluster=w579, "Initialized"=TRUE, "Connected"=w577, "Ready"=w577, "Inspecting"=w577, "Error"=w577) -> (w574:T9)
            n53 = call "Error Event.vi"("error in (no error)"=w593, "EventLog ref"=w582) -> ("error out"=w589:errorcluster)  [unwired: 8 in, 1 out]
            n54 = call <vilib>:"General Error Handler.vi"("error in (no error)"=w583, "[exception action] (none:0)"=w586, "[exception code]"=538053) -> ("error out"=w584:errorcluster)  [unwired: 8 in, 4 out]
            n55 = Merge Errors(w589, w565, w584) -> (w588:errorcluster)
            n56 = Bundle By Name(cluster=w580, "Trig State"=w576, "LED State 1"=w576, "LED State 2"=w576, "OK to Connect"=w576, "Connecting"=w576, "Got FW Ver"=w576, "Got Tool Type"=w576, "Got Tool Cfg"=w576, "Got Fmt Params"=w576, "Got FPGA Setup"=w576, "STATUS"=w574) -> (w575:T8)
            n57 = call "Close Tool Connection.vi"() -> ("error out"=w595:errorcluster)  [unwired: 11 in]
            n58 = call <vilib>:"Simple Error Handler.vi"("error in (no error)"=w588) -> ("error out"=w587:errorcluster)  [unwired: 4 in, 4 out]
            n59 = call <vilib>:"Clear Errors.vi"("error in (no error)"=w595) -> ()  [unwired: 5 in, 2 out]
            n60 = call <vilib>:"Clear Errors.vi"("error in (no error)"=w587) -> ()  [unwired: 5 in, 2 out]
          }
          frame "Tool Status Updated" {
            # "Tool Status Updated is used for the Status update timer. This will send a status update event to the main app regularly. (50mSec)"
            n61 = Variant To Data(type=T56 {"Tool Status"={"Encoder"=0, "STATUS"=0, "MC SM State"=0, "M_Ctrl"=0}, "Reader SM State"=enum."Not Connected"} ("_Tool Status Update Cluster--typedef"), Variant=w615) -> (data=w606:T56, error out=w607:errorcluster)  [unwired: 1 in]
            n62 = Unbundle By Name(w635) -> ("Status Update Cnt"=w611:i32, "Connecting"=w619:bool, "OK to Connect"=w618:bool, "Trig State"=w633:bool, "STATUS"=w631:T9, "EventLog.lvclass"=w626:refnum<class "EventLog.lvclass">, "STATUS.Connected"=w620:bool)
            n63 = Unbundle By Name(w606) -> ("Tool Status"=w613:T5, "Reader SM State"=w612:T6)
            n64 = Unbundle By Name(w613) -> ("Encoder"=w632:i32, "STATUS"=w610:u16, "MC SM State"=w624:u16, "M_Ctrl"=w623:u16)
            n65 = call "Encoder to Inch.vi"("Encoder in"=w632) -> ("Encoder out(in)"=w625:dbl)  [unwired: 14 in]
            n66 = Bundle By Name(cluster=w631, "Code"=w611, "Position"=w625, "Status"=w610, "MC SM State"=w624, "M_Ctrl"=w623) -> (w634:T9)
            n67 = call "Update Tool Status Helper.vi"("STATUS Cluster in"=w634, "error in (no error)"=w607, "Trig State in"=w633, "OK to Connect"=w618, "Connecting"=w619) -> ("error out"=w637:errorcluster, "Trig State out"=w622:bool, "Stream Connected"=w616:bool, "STATUS Cluster out"=w621:T9)  [unwired: 3 in]
            n68 = Increment(x=w611) -> (x+1=w630:i32)
            n69 = call "Send Status.vi"("error in (no error)"=w637, "STATUS"=w621) -> ("error out"=w636:errorcluster)  [unwired: 9 in]
            n70 = Number To Hexadecimal String(2:w610) -> (0:w609:string)  [unwired: 1 in]
            n71 = Format Into String(w625, w609, w624, w623, w616, w620, w619, w618, w612) -> (resulting string=w617:string)  [unwired: 3 in, 1 out]
            n72 = Bundle By Name(cluster=w635, "Status Update Cnt"=w630, "Trig State"=w622, "Encoder Count"=w632, "STATUS"=w621) -> (w629:T8)
            n73 = call "Log General Event Helper.vi"("Payload"=w617, "State Info"=w608, "EventLog in"=w626) -> ("error out"=w627:errorcluster)  [unwired: 7 in, 1 out]
            n74 = Merge Errors(w636, w627) -> (w628:errorcluster)
          }
          frame "Update Inspect Status" {
            # "Send B'cast to Tool Status Reader State Machine Helper Loop to trigger an update to the tool status using the new settings here. Can't just queue up request to Tool Status Updated state, because we don't have the payload to deliver."
            # "Update the Ready, Inspecting, and Cancel status flags in the MHL data from the 'Inspecting Helper Loop'. It queues this state whenever it modifies any of these flags."
            n75 = Variant To Data(type=T4 {"Ready"=FALSE, "Inspecting"=FALSE, "Cancel"=FALSE} ("Inspect Status"), Variant=w654) -> (data=w649:T4, error out=w650:errorcluster)  [unwired: 1 in]
            n76 = Unbundle By Name(w644) -> ("EventLog.lvclass"=w643:refnum<class "EventLog.lvclass">)
            n77 = Unbundle By Name(w649) -> ("Ready"=w642:bool, "Inspecting"=w641:bool, "Cancel"=w640:bool)
            n78 = call "Time Expired.vi"("error in (no error)"=w650, "ID"=1) -> ("error out"=w648:errorcluster)  [unwired: 9 in]
            n79 = Format Into String(format string="Ready=%s, Inspecting=%s, Cancel=%s", w642, w641, w640) -> (resulting string=w639:string)  [unwired: 2 in, 1 out]
            n80 = Bundle By Name(cluster=w644, "STATUS.Ready"=w642, "STATUS.Inspecting"=w641, "Cancel Inspect"=w640) -> (w652:T8)
            n81 = call "Log General Event Helper.vi"("Payload"=w639, "State Info"=w645, "EventLog in"=w643) -> ("error out"=w646:errorcluster)  [unwired: 7 in, 1 out]
            n82 = Merge Errors(w648, w646) -> (w647:errorcluster)
          }
          frame "FPGA Acq Status Rtn" {
            # "This state exists for the debug log.."
            n83 = Variant To Data(type=T57 {"TE_Running"=FALSE, "PD_Running"=FALSE, "Laser On 1"=FALSE, "Laser On 2"=FALSE} ("_FPGA Run Status Rtn Cluster--typedef"), Variant=w672) -> (data=w655:T57, error out=w656:errorcluster)  [unwired: 1 in]
            n84 = Unbundle By Name(w663) -> ("EventLog.lvclass"=w659:refnum<class "EventLog.lvclass">)
            n85 = Unbundle By Name(w655) -> ("TE_Running"=w670:bool, "PD_Running"=w669:bool, "Laser On 1"=w668:bool, "Laser On 2"=w667:bool)
            n86 = Unbundle By Name(w656) -> ("code"=w657:i32)
            n87 = Format Into String(format string="TE_Running=%s, PD_Running=%s, Laser On 1=%s, Laser On 2=%s, ErrCode=%d", w670, w669, w668, w667, w657) -> (resulting string=w660:string)  [unwired: 2 in, 1 out]
            n88 = call "Log General Event Helper.vi"("Payload"=w660, "State Info"=w661, "EventLog in"=w659) -> ("error out"=w662:errorcluster, "EventLog out"=w658:refnum<class "EventLog.lvclass">)  [unwired: 7 in]
            n89 = call "Error Event.vi"("error in (no error)"=w656, "EventLog ref"=w658) -> ("error out"=w665:errorcluster)  [unwired: 8 in, 1 out]
            n90 = Merge Errors(w665, w662) -> (w664:errorcluster)
          }
          frame "------- Event Handlers -------" {
            # "These states handle specific events (commands) from the calling app."
            n91 = Merge Errors(w675) -> (w673:errorcluster)
          }
          frame "CONNECT" {
            # "Attempt to connect/disconnect from the tool. Report back with Success, Tool Type and Tool Serial Number. Set OK to Connect to True (even if unsuccessful). This tells the system to keep trying to connect (see Timer Event 2 state)."
            n92 = Unbundle By Name(w690) -> ("STATUS.Connected"=w682:bool)
            n93 = Variant To Data(type=T21 {"Connect"=FALSE} ("CONNECT Argument"), Variant=w692) -> (data=w694:T21, error out=w695:errorcluster)  [unwired: 1 in]
            n94 = Unbundle By Name(w694) -> ("Connect"=w681:bool)
            n95 = case shown="False" w681 {
              tunnel: w695 -> [w699 w730]
              tunnel: [w699 w729] -> w689
              tunnel: w682 -> [w704 w728]
              tunnel: [w700 w727] -> w680
              tunnel: T58 {"Connected"=FALSE, "Tool Type"=0, "Tool SN"=0} ("Connected Argument") -> [w701 w726]
              tunnel: w690 -> [w703 w725]
              tunnel: [w702 w724] -> w685
              tunnel: [w698 w723] -> w684
              tunnel: w696 -> [_ w722]
              tunnel: w686 -> [w697 w721]
              frame False {
                # "Disconnect"
                n96 = case shown="True" w704 {
                  tunnel: w703 -> [w705 w719]
                  tunnel: [w705 w715] -> w702
                  tunnel: w701 -> [_ w718]
                  tunnel: [_ w716] -> w700
                  tunnel: [_ w714] -> w698
                  tunnel: w697 -> [_ w712]
                  frame False {
                    # "Already disconnected: do nothing"
                  }
                  frame True {
                    w711 = FALSE  # Connected
                    w713 = FALSE ("STATUS.Connected")
                    # "Connected, so disconnect"
                    n97 = call "Enable Receive Stream.vi"("Enable"=FALSE) -> ("error out"=w720:errorcluster)  [unwired: 10 in]
                    n98 = Send Notification(notification=w711, notifier=w712) -> ()  [unwired: 1 in, 2 out]
                    n99 = Bundle By Name(cluster=w719, "STATUS.Connected"=w713, "STATUS.Ready"=w713, "Trig State"=w713, "STATUS.Inspecting"=w713, "Connecting"=w713) -> (w715:T8)
                    n100 = call "Tool Status Reader Cmd.vi"("error in (no error)"=w720, "Command"=_Host_-_HS_Data_Stream_State_Enum_Typedef."Close Connection" ("notification")) -> ("error out"=w708:errorcluster)  [unwired: 9 in]
                    n101 = Bundle By Name(cluster=w718, "Connected"=FALSE) -> (w716:T58)
                    n102 = call "wait (ms) with error clusters.vi"("error in (no error)"=w708, "milliseconds to wait"=u32 2000) -> ("error out"=w710:errorcluster)  [unwired: 9 in]
                    n103 = call "Close Tool Connection.vi"("error in (no error)"=w710) -> ("error out"=w714:errorcluster)  [unwired: 10 in]
                  }
                }
              }
              frame True {
                # "Connect"
                n104 = case shown="False" w728 {
                  tunnel: w730 -> [w743 w761]
                  tunnel: [w742 w761] -> w729
                  tunnel: [w749 w764] -> w727
                  tunnel: w726 -> [w748 w765]
                  tunnel: w725 -> [w747 w762]
                  tunnel: [w746 w762] -> w724
                  tunnel: [w735 _] -> w723
                  tunnel: w722 -> [w741 _]
                  tunnel: w721 -> [w739 _]
                  frame False {
                    # "Note, if no tool, this VI takes 2 seconds to execute."
                    # "Start the Message Stream"
                    # "Start the Motion\nStatus Stream"
                    # "Not connected, so connect"
                    n105 = disable-structure shown="Enabled" {
                      disable-tunnel: [w753 _] -> w736
                      frame Enabled {
                        n106 = call "Close Tool Connection.vi"() -> ("error out"=w753:errorcluster)  [unwired: 11 in]
                      }
                      frame Disabled {
                      }
                    }
                    n107 = disable-structure shown="Enabled" {
                      disable-tunnel: [w752 _] -> w744
                      disable-tunnel: [w751 _] -> w740
                      disable-tunnel: w736 -> [w750 _]
                      frame Enabled {
                        n108 = call "ConnectOnly.vi"("error in (no error)"=w750) -> ("error out"=w752:errorcluster, "Success"=w751:bool)  [unwired: 9 in]
                      }
                      frame Disabled {
                      }
                    }
                    n109 = case shown="True" w740 {
                      tunnel: w743 -> [w754 w758]
                      tunnel: [w754 w757] -> w742
                      tunnel: w741 -> [_ w756]
                      frame False {
                      }
                      frame True {
                        n110 = call-poly <vilib>:"Delacor_lib_QMH_Enqueue Message (poly).vi"("error in (no error)"=w758, "Message"="Connect: Get Version", "Message Queue in"=w756) -> ("error out"=w757:errorcluster)  [unwired: 7 in, 1 out]
                      }
                    }
                    n111 = Send Notification(notification=w740, notifier=w739, error in (no error)=w744) -> (error out=w733:errorcluster)  [unwired: 1 out]
                    n112 = call "Enable Receive Stream.vi"("error in (no error)"=w733, "Enable"=TRUE) -> ("error out"=w732:errorcluster)  [unwired: 9 in]
                    n113 = Bundle By Name(cluster=w747, "Timer 2 Call State"="Check if Ready", "Connecting"=w740, "OK to Connect"=TRUE) -> (w746:T8)
                    n114 = call "Tool Status Reader Cmd.vi"("error in (no error)"=w732, "Command"=_Host_-_HS_Data_Stream_State_Enum_Typedef."Connect") -> ("error out"=w735:errorcluster)  [unwired: 9 in]
                    n115 = Bundle By Name(cluster=w748, "Connected"=FALSE) -> (w749:T58)
                  }
                  frame True {
                    # "Already Connected"
                    n116 = call "Get Tool Type and SN.vi"() -> ("Tool SN"=w759:u16, "Tool Type"=w760:u16)  [unwired: 10 in]
                    n117 = Bundle By Name(cluster=w765, "Connected"=TRUE, "Tool Type"=w760, "Tool SN"=w759) -> (w764:T58)
                  }
                }
              }
            }
            n118 = Unbundle By Name(w685) -> ("EventLog.lvclass"=w679:refnum<class "EventLog.lvclass">)
            n119 = call "Connected.vi"("error in (no error)"=w689, "Connected Argument"=w680) -> ("error out"=w688:errorcluster)  [unwired: 9 in]
            n120 = call "Log Connect Event Helper.vi"("Connected Argument"=w680, "State Info"=w677, "Connecting"=w681, "Connected"=w682, "EventLog in"=w679) -> ("error out"=w676:errorcluster, "EventLog out"=w678:refnum<class "EventLog.lvclass">)  [unwired: 5 in]
            n121 = call "Error Event.vi"("error in (no error)"=w684, "EventLog ref"=w678) -> ("error out"=w683:errorcluster)  [unwired: 8 in, 1 out]
            n122 = Merge Errors(w688, w683, w676) -> (w687:errorcluster)
          }
          frame "GOTO" {
            n123 = Unbundle By Name(w771) -> ("EventLog.lvclass"=w770:refnum<class "EventLog.lvclass">)
            n124 = Variant To Data(error in=w780, type=T22 {"GoTo Cmd"=enum."MoveA", "Data"=0} ("GOTO Argument"), Variant=w779) -> (data=w777:T22, error out=w774:errorcluster)
            n125 = Unbundle By Name(w777) -> ("Data"=w768:i32, "GoTo Cmd"=w767:T23)
            n126 = call "Log GoTo State Helper.vi"("State Info"=w769, "GoTo Cmd"=w767, "Data"=w768, "EventLog in"=w770) -> ("error out"=w766:errorcluster)  [unwired: 6 in, 1 out]
            n127 = case shown="\"MoveA\"" w767 {
              tunnel: w768 -> [_ _ w809 w820 _ _]
              tunnel: [w792 w795 w802 w813 w825 _] -> w775
              tunnel: w774 -> [w790 w800 w810 w821 w832 w835]
              tunnel: [w789 w800 w810 w821 w832 w835] -> w772
              tunnel: w781 -> [_ w799 _ _ _ _]
              tunnel: w771 -> [w793 w797 w801 w812 w823 w834]
              tunnel: [w787 w797 w801 w812 w823 w834] -> w773
              frame "Home Position" {
                w784 = 1000  # Period
                # "Set a 1 second timer which will\nthen go to the Homing: Check Home Off State."
                # "Need to send status update\nimmediately so main sees\nReady as False for Home."
                n128 = Bundle By Name(cluster=w793, "STATUS.Ready"=FALSE, "Loop Counter"=0 ("Count")) -> (w787:T8)
                n129 = Unbundle By Name(w787) -> ("STATUS"=w788:T9)
                n130 = call "Setup Delay for Next State.vi"("Period"=w784, "Next State"="Homing: Check Home Off" ("Timer 2 Call State")) -> ("error out"=w782:errorcluster)  [unwired: 9 in]
                n131 = call "Motion Home.vi"("Home(T)/Fake(F)"=TRUE) -> ("error out"=w794:errorcluster)  [unwired: 10 in]
                n132 = call "Send Status.vi"("error in (no error)"=w790, "STATUS"=w788) -> ("error out"=w789:errorcluster)  [unwired: 9 in]
                n133 = Merge Errors(w782, w794) -> (w792:errorcluster)
              }
              frame "Home None" {
                w796 = FALSE  # Home(T)/Fake(F)
                n134 = call-poly <vilib>:"Delacor_lib_QMH_Enqueue Message (poly).vi"("Message"="Ready", "Message Queue in"=w799) -> ()  [unwired: 8 in, 2 out]
                n135 = call "Motion Home.vi"("Home(T)/Fake(F)"=w796) -> ("error out"=w795:errorcluster)  [unwired: 10 in]
              }
              frame "MoveR" {
                w808 = FALSE  # Decel?
                n136 = call "Get Jog Speed.vi"() -> ("Jog Speed"=w807:u16)  [unwired: 11 in]
                n137 = call "Motion Set Speed.vi"("Speed"=w807) -> ("error out"=w803:errorcluster)  [unwired: 10 in]
                n138 = call "Wait(ms).vi"("error in (no error)"=w803, "milliseconds"=u32 50 ("Milliseconds to wait")) -> ("error out"=w811:errorcluster)  [unwired: 9 in]
                n139 = call "Motion Move Relative.vi"("error in (no error)"=w811, "Decel?"=w808, "Distance"=w809) -> ("error out"=w804:errorcluster)  [unwired: 8 in]
                n140 = call "Wait(ms).vi"("error in (no error)"=w804, "milliseconds"=u32 100 ("Milliseconds to wait")) -> ("error out"=w802:errorcluster)  [unwired: 9 in]
              }
              frame "MoveA" {
                w819 = FALSE  # Decel?
                n141 = call "Get Jog Speed.vi"() -> ("Jog Speed"=w818:u16)  [unwired: 11 in]
                n142 = call "Motion Set Speed.vi"("Speed"=w818) -> ("error out"=w814:errorcluster)  [unwired: 10 in]
                n143 = call "Wait(ms).vi"("error in (no error)"=w814, "milliseconds"=u32 50 ("Milliseconds to wait")) -> ("error out"=w822:errorcluster)  [unwired: 9 in]
                n144 = call "Motion Move Absolute.vi"("error in (no error)"=w822, "Decel?"=w819, "Position"=w820) -> ("error out"=w815:errorcluster)  [unwired: 8 in]
                n145 = call "Wait(ms).vi"("error in (no error)"=w815, "milliseconds"=u32 100 ("Milliseconds to wait")) -> ("error out"=w813:errorcluster)  [unwired: 9 in]
              }
              frame "Cleaning Position" {
                w831 = FALSE  # Decel?
                n146 = call "Get Jog Speed.vi"() -> ("Jog Speed"=w830:u16)  [unwired: 11 in]
                n147 = call "Motion Set Speed.vi"("Speed"=w830) -> ("error out"=w826:errorcluster)  [unwired: 10 in]
                n148 = call "Wait(ms).vi"("error in (no error)"=w826, "milliseconds"=u32 50 ("Milliseconds to wait")) -> ("error out"=w833:errorcluster)  [unwired: 9 in]
                n149 = call "Get Cleaning Position.vi"() -> ("CleaningPos"=w824:i32)  [unwired: 11 in]
                n150 = call "Motion Move Absolute.vi"("error in (no error)"=w833, "Decel?"=w831, "Position"=w824) -> ("error out"=w827:errorcluster)  [unwired: 8 in]
                n151 = call "Wait(ms).vi"("error in (no error)"=w827, "milliseconds"=u32 100 ("Milliseconds to wait")) -> ("error out"=w825:errorcluster)  [unwired: 9 in]
              }
              frame Default {
              }
            }
            n152 = Merge Errors(w775, w772, w766) -> (w776:errorcluster)
          }
          frame "MONITOR" {
            n153 = Unbundle By Name(w848) -> ("EventLog.lvclass"=w841:refnum<class "EventLog.lvclass">, "STATUS.Ready"=w840:bool)
            n154 = Variant To Data(type=T25 {"Monitor"=FALSE, "Lasers ON?"=FALSE, "Host Sample Data notifier"=refnum} ("Start Data Monitor Argument"), Variant=w852) -> (data=w850:T25, error out=w844:errorcluster)  [unwired: 1 in]
            n155 = Unbundle By Name(w850) -> ("Monitor"=w839:bool, "Lasers ON?"=w838:bool, "Host Sample Data notifier"=w845:refnum<notifier>)
            n156 = call "Log Monitor State Helper.vi"("Laser ON?"=w838, "State Info"=w837, "Monitor"=w839, "STATUS.Ready"=w840, "EventLog in"=w841) -> ("error out"=w836:errorcluster)  [unwired: 5 in, 1 out]
            n157 = Not(x=w839) -> (.not. x?=w846:bool)
            n158 = And(x=w840, y=w839) -> (x .and. y?=w849:bool)
            n159 = case shown="True" w849 {
              tunnel: w848 -> [w857 w866]
              tunnel: [w856 w865] -> w847
              tunnel: w846 -> [w855 w864]
              tunnel: w845 -> [_ w863]
              tunnel: w844 -> [w854 w862]
              tunnel: w853 -> [_ w861]
              tunnel: [w854 w859] -> w843
              tunnel: w838 -> [_ w858]
              frame False {
                n160 = Bundle By Name(cluster=w857, "Cancel Inspect"=w855) -> (w856:T8)
              }
              frame True {
                # "Start Monitor only if Ready is true. Clear the Inspecting flag and the Scan Data Array in the Sample Data Notifier. Main App will wait for Inspecting to go True."
                n161 = Bundle By Name(cluster=w866, "Cancel Inspect"=w864, "Host SampleData"=w863) -> (w865:T8)
                n162 = call-poly <vilib>:"Delacor_lib_QMH_Enqueue Message (poly).vi"("error in (no error)"=w862, "Message Data"=w858, "Message"="Start Monitor", "Message Queue in"=w861) -> ("error out"=w859:errorcluster)  [unwired: 6 in, 1 out]
              }
            }
            n163 = Merge Errors(w843, w836) -> (w842:errorcluster)
          }
          frame "Get Mtr Ctrl Reg" {
            # "Retrieves the Mtr Ctrl Reg current state from the FPGA Support Global which is a copy of what was used to set the FPGA."
            n164 = Variant To Data(error in=w878, type=T44 {"dummy"=FALSE, "Wait Notifier"=refnum} ("Get Mtrl Ctrl Reg Argument"), Variant=w877) -> (data=w875:T44, error out=w868:errorcluster)
            n165 = Unbundle By Name(w875) -> ("Wait Notifier"=w874:refnum<notifier>)
            n166 = global read "ToolModGLOB.vi" "Mtr Ctrl Reg(File)"() -> (w867:u16)
            n167 = Bundle By Name(cluster=T59 {"Mtr Ctrl Reg"=0, "Get Mtrl Ctrl Reg_error"={"status"=FALSE, "code"=0, "source"=""}} ("Get Mtrl Ctrl Reg (Reply Payload)"), "Mtr Ctrl Reg"=w867, "Get Mtrl Ctrl Reg_error"=w868) -> (w873:T59)
            n168 = Send Notification(notification=w873, notifier=w874) -> (error out=w870:errorcluster)  [unwired: 1 in, 1 out]
            n169 = Merge Errors(w870) -> (w872:errorcluster)
          }
          frame "Commit Ctrl Reg" {
            # "Send a new value for the Ctrl Register to the Tool. \nNeed to send new value to RT and have RT write to the XML file."
            n170 = Variant To Data(error in=w887, type=T45 {"Ctrl Reg"=0} ("Set Mtr Ctrl Reg Argument"), Variant=w885) -> (data=w883:T45, error out=w886:errorcluster)
            n171 = Unbundle By Name(w883) -> ("Ctrl Reg"=w879:u16)
            n172 = call "Commit Ctrl Reg.vi"("Ctrl Reg"=w879) -> ("error out"=w881:errorcluster)  [unwired: 10 in]
            n173 = Merge Errors(w881, w886) -> (w882:errorcluster)
          }
          frame "Get-Set Inspection Limits" {
            # "If Set is True, then don't do wait for reply."
            # "Get or Set the Inspection Limits. These are local parameters for the Tool Module operation (not in the tool)."
            n174 = Variant To Data(error in=w904, type=T54 {"Set"=FALSE, "Inspection Limits"={"MaxSamples"=50800, "PosToStartScan"=50800, "PosToEndScan"=0, "ScanLength"=50800}, "Wait Notifier"=refnum, "wait for reply"=FALSE} ("Get-Set Inspection Limits Argument"), Variant=w902) -> (data=w900:T54, error out=w903:errorcluster)
            n175 = Unbundle By Name(w900) -> ("Set"=w893:bool, "Inspection Limits"=w894:T11, "Wait Notifier"=w899:refnum<notifier>, "wait for reply"=w892:bool)
            n176 = case shown="True" w893 {
              tunnel: [w905 w908] -> w888
              tunnel: w889 -> [w905 w907]
              tunnel: w894 -> [_ w906]
              frame False {
              }
              frame True {
                n177 = Bundle By Name(cluster=w907, "Inspection Limits"=w906) -> (w908:T8)
              }
            }
            n178 = Unbundle By Name(w888) -> ("Inspection Limits"=w895:T11)
            n179 = Compound Arithmetic op=AND(invert w893, w892) -> (w891:bool)
            n180 = Bundle By Name(cluster=T60 {"Inspection Limits"={"MaxSamples"=50800, "PosToStartScan"=50800, "PosToEndScan"=0, "ScanLength"=50800}, "Get-Set Inspection Limits_error"={"status"=FALSE, "code"=0, "source"=""}} ("Get-Set Inspection Limits (Reply Payload)"), "Inspection Limits"=w895) -> (w898:T60)
            n181 = case shown="True" w891 {
              tunnel: w899 -> [_ w911]
              tunnel: w898 -> [_ w910]
              tunnel: [_ w909] -> w890
              frame False {
              }
              frame True {
                n182 = Send Notification(notification=w910, notifier=w911) -> (error out=w909:errorcluster)  [unwired: 1 in, 1 out]
              }
            }
            n183 = Merge Errors(w903, w890) -> (w896:errorcluster)
          }
          frame "Get FPGA Setup Params" {
            n184 = Variant To Data(error in=w923, type=T26 {"dummy"=FALSE, "Wait Notifier"=refnum} ("Get FPGA Setup Params Argument"), Variant=w922) -> (data=w920:T26, error out=w914:errorcluster)
            n185 = Unbundle By Name(w920) -> ("Wait Notifier"=w919:refnum<notifier>)  [unwired: 1 out]
            n186 = global read "ToolModGLOB.vi" "FPGA Setup Parameters"() -> (w916:T28)
            n187 = global read "ToolModGLOB.vi" "Version String"() -> (w912:string)
            n188 = Bundle By Name(cluster=T61 {"Version String"="", "FPGA Setup Parameters"={"FPGA Timing Constraints"={"frame.length Min"=530, "frame.ST_OFF Min"=15, "frame.ST_ON Min"=8, "frame.first data idx"=14, "frame.integ Offset"=6, "frame.integ Delay"=3, "frame.ad_latch Delay"=11, "frame.trig time Max"=0}, "FPGA Timing Ctrl"={"trig.time"=220, "integ.count 1"=400, "integ.count 2"=350, "encdr.latch ctrl"=1, "pixel.read count"=512, "clock.select"=2, "ad.clock offset"=16, "data.control reg"=2}, "FPGA Laser Config"={"laser.gain"=10, "laser.threshold Low"=1400, "laser.threshold High"=1900, "laser.dac init"=912, "laser.dac Min"=800, "laser.dac Max"=4000, "laser.config reg"=3}, "FPGA Peak Proc Cfg"={"PD.threshold"=0, "PD.width detect Min"=0, "PD.sensor pixels"=512, "PD.config reg"=23}, "FPGA SPI Cfg"={"SPI Divide Value"=1, "SPI config reg"=1}}} ("Get FPGA Setup Params (Reply Payload)"), "Version String"=w912, "FPGA Setup Parameters"=w916) -> (w915:T61)
            n189 = Send Notification(notification=w915, notifier=w919, error in (no error)=w914) -> (error out=w913:errorcluster)  [unwired: 1 out]
          }
          frame "Set FPGA Setup Params" {
            # "Sets the Tool Mgr copy and also the working (volatile) copy in the Tool."
            n190 = Variant To Data(type=T27 {"Commit"=FALSE, "FPGA Setup Parameters"={"FPGA Timing Constraints"={"frame.length Min"=530, "frame.ST_OFF Min"=15, "frame.ST_ON Min"=8, "frame.first data idx"=14, "frame.integ Offset"=6, "frame.integ Delay"=3, "frame.ad_latch Delay"=11, "frame.trig time Max"=0}, "FPGA Timing Ctrl"={"trig.time"=220, "integ.count 1"=400, "integ.count 2"=350, "encdr.latch ctrl"=1, "pixel.read count"=512, "clock.select"=2, "ad.clock offset"=16, "data.control reg"=2}, "FPGA Laser Config"={"laser.gain"=10, "laser.threshold Low"=1400, "laser.threshold High"=1900, "laser.dac init"=912, "laser.dac Min"=800, "laser.dac Max"=4000, "laser.config reg"=3}, "FPGA Peak Proc Cfg"={"PD.threshold"=0, "PD.width detect Min"=0, "PD.sensor pixels"=512, "PD.config reg"=23}, "FPGA SPI Cfg"={"SPI Divide Value"=1, "SPI config reg"=1}}} ("Set Cur FPGA Setup Params Argument"), Variant=w934) -> (data=w932:T27, error out=w930:errorcluster)  [unwired: 1 in]
            n191 = Unbundle By Name(w932) -> ("Commit"=w924:bool, "FPGA Setup Parameters"=w929:T28)
            n192 = Select(t="Commit FPGA Setup Params", s=w924, f="Set Cur FPGA Setup" ("Message")) -> (s? t:f=w925:string)
            n193 = call "Message to RT.vi"("error in (no error)"=w930, "Message Data"=w929, "Message"=w925) -> ("error out"=w928:errorcluster)  [unwired: 8 in]
            n194 = case shown="No Error" w928 {
              tunnel: w929 -> [w935 _]
              frame No Error {
                n195 = global write "ToolModGLOB.vi" "FPGA Setup Parameters"(w935) -> ()
              }
              frame Error {
              }
            }
          }
          frame "Commit Tool Config" {
            # "Saves Tool Configuration to Tool. Currently, the Commit element is ignored. The data is stored in the Tools file system."
            n196 = Variant To Data(error in=w945, type=T34 {"Tool Config Cluster"={"Tool Type"=0, "Tool SN"=0, "Tool Block"={"Encoder Size"=0, "Encoder Scale"=0, "Encoder Offset"=0, "MaxEncoder"=0, "MinEncoder"=0, "Start Delay"=0.0, "Tool Face Ref"=0.0}, "Motor Block"={"MinMotor Speed"=0, "MaxMotor Speed"=0, "Homing Speed"=90, "Jog Speed"=90, "Inspect Speed"=90, "VBlk Speed"=90, "CleaningPos"=0, "Safe Zone"=0, "Has Motor"=FALSE, "Use Home Index"=FALSE}, "Verification Block"={"Angle"=90.0, "FlankLength1"=0.0, "FlankLength2"=0.0, "Location"=0.0, "Serial Number"=0}, "Probe Block"={"nProbes"=0, "Probe Param Array"=[]}}} ("Set Tool Config Argument"), Variant=w944) -> (data=w942:T34, error out=w941:errorcluster)
            n197 = Unbundle By Name(w937) -> ("STATUS.Connected"=w936:bool)
            n198 = Unbundle By Name(w942) -> ("Tool Config Cluster"=w938:T35)
            n199 = call "Message to RT.vi"("error in (no error)"=w941, "Message Data"=w938, "Message"="Commit Tool Config", "Connected(T)"=w936) -> ("error out"=w940:errorcluster)  [unwired: 7 in]
          }
          frame "Get All Inspect Data" {
            # "Use the Data value ref to get the scan data, reverse it and send as reply to caller. We close the data value ref here. \n10Oct19 DJS - Process data in the Reverse Data Set VI in an inplace structure, so pass the DVR in and out. Return DVR to caller rather than data array."
            n200 = disable-structure shown="Disabled" {
              disable-tunnel: w949 -> [w964 _]
              disable-tunnel: w948 -> [w963 _]
              disable-tunnel: w947 -> [w959 _]
              disable-tunnel: [w954 _] -> w946
              frame Disabled {
                n201 = Unbundle By Name(w959) -> ("CD Success"=w957:bool, "Final No. of Blks"=w953:i32, "Inspection Limits.PosToStartScan"=w955:i32, "data value reference"=w965:refnum<data-value>)
                n202 = Variant To Data(error in=w964, type=T24 {"dummy"=FALSE, "Wait Notifier"=refnum} ("Get All Inspect Data Argument"), Variant=w963) -> (data=w961:T24, error out=w951:errorcluster)
                n203 = Unbundle By Name(w961) -> ("Wait Notifier"=w960:refnum<notifier>)
                n204 = call "Reverse Data Set V2.vi"("Pos to Start Scan"=w955, "data value reference"=w965, "Final No of Blocks"=w953) -> ("data value ref out"=w952:refnum<data-value>)  [unwired: 8 in]
                n205 = Bundle By Name(cluster=T18 {"Success"=FALSE, "Full Inspection Data"=[], "data value reference"=refnum} ("Get All Inspect Data (Reply Payload)"), "Success"=w957, "data value reference"=w952) -> (w956:T18)
                n206 = Send Notification(notification=w956, notifier=w960) -> (error out=w950:errorcluster)  [unwired: 1 in, 1 out]
                n207 = Merge Errors(w951, w950) -> (w954:errorcluster)
              }
              frame Enabled {
              }
            }
          }
          frame "Set Laser Params" {
            # "13May2019, DJS, For RT FW Ver 1.7 and higher, use new 'Pull FPGA Setup form Tool' command so as not to overwrite the new local FPGA settings (which the old 'Get Cur FPGA Setup' cmd does)."
            # "Sets the Gain and Init value for laser control."
            n208 = Unbundle By Name(w972) -> ("FW Ver Maj/Min"=w967:dbl)
            n209 = Variant To Data(error in=w982, type=T43 {"Mode"=0, "Gain"=0, "Init DAC"=0} ("Set Laser Params Argument"), Variant=w981) -> (data=w979:T43, error out=w977:errorcluster)
            n210 = Unbundle By Name(w979) -> ("Mode"=w976:i16, "Init DAC"=w974:u16, "Gain"=w973:u16)
            n211 = Greater Or Equal?(x=w967, y=1.7) -> (x >= y?=w966:bool)
            n212 = call "Laser Config.vi"("error in (no error)"=w977, "Gain"=w973, "Init Power"=w974, "Select Probe"=w976) -> ("error out"=w975:errorcluster)  [unwired: 7 in]
            n213 = call "Wait(ms).vi"("error in (no error)"=w975, "milliseconds"=u32 50) -> ("error out"=w971:errorcluster)  [unwired: 9 in]
            n214 = case shown="False" w966 {
              tunnel: [w984 w989] -> w970
              tunnel: w969 -> [_ w988]
              tunnel: w971 -> [w985 w986]
              frame False {
                n215 = call "Message to RT.vi"("error in (no error)"=w985, "Message"="Pull FPGA Setup from Tool") -> ("error out"=w984:errorcluster)  [unwired: 9 in]
              }
              frame True {
                n216 = call-poly <vilib>:"Delacor_lib_QMH_Enqueue Message (poly).vi"("error in (no error)"=w986, "Message"="Get Cur FPGA Setup", "Message Queue in"=w988) -> ("error out"=w989:errorcluster)  [unwired: 7 in, 1 out]
              }
            }
          }
          frame "Set Integration Count" {
            # "13May2019, DJS, For RT FW Ver 1.7 and higher, use new 'Pull FPGA Setup form Tool' command so as not to overwrite the new local FPGA settings (which the old 'Get Cur FPGA Setup' cmd does)."
            # "Sets either one or both integration counts."
            n217 = Unbundle By Name(w993) -> ("FW Ver Maj/Min"=w991:dbl)
            n218 = Variant To Data(error in=w1005, type=T42 {"Mode"=0, "Integ Count"=0} ("Set Integration Count Argument"), Variant=w1004) -> (data=w1002:T42, error out=w999:errorcluster)
            n219 = Unbundle By Name(w1002) -> ("Mode"=w1001:i16, "Integ Count"=w1000:u32)
            n220 = Greater Or Equal?(x=w991, y=1.7) -> (x >= y?=w990:bool)
            n221 = call "Set Integration.vi"("error in (no error)"=w999, "Integ Count"=w1000, "Mode"=w1001) -> ("error out"=w996:errorcluster)  [unwired: 8 in]
            n222 = call "Wait(ms).vi"("error in (no error)"=w996, "milliseconds"=u32 50) -> ("error out"=w994:errorcluster)  [unwired: 9 in]
            n223 = case shown="False" w990 {
              tunnel: [w1007 w1012] -> w998
              tunnel: w997 -> [_ w1011]
              tunnel: w994 -> [w1008 w1009]
              frame False {
                n224 = call "Message to RT.vi"("error in (no error)"=w1008, "Message"="Pull FPGA Setup from Tool") -> ("error out"=w1007:errorcluster)  [unwired: 9 in]
              }
              frame True {
                n225 = call-poly <vilib>:"Delacor_lib_QMH_Enqueue Message (poly).vi"("error in (no error)"=w1009, "Message"="Get Cur FPGA Setup", "Message Queue in"=w1011) -> ("error out"=w1012:errorcluster)  [unwired: 7 in, 1 out]
              }
            }
          }
          frame "Read from File", "Write to File" {
            # "Send flattened XML data string to the tool to save in 'Filename' file.  The error status is returned in \"Write from File Rtn\".\n-OR-\nRead flattened XML data string from the specified file.The flattened XML data string and an error status cluster are returned via broadcast event."
            n226 = case shown="\"Write to File\", Default" w1016 {
              tunnel: w1015 -> [w1027 w1031]
              tunnel: [w1020 w1029] -> w1014
              tunnel: [w1019 w1028] -> w1013
              frame "Write to File", Default {
                n227 = Variant To Data(type=T47 {"Filename"="", "Flattened data strings"=[]} ("Write to File Argument"), Variant=w1027) -> (data=w1026:T47, error out=w1019:errorcluster)  [unwired: 1 in]
                n228 = Unbundle By Name(w1026) -> ("Filename"=w1023:string, "Flattened data strings"=w1022:string[])
                n229 = Bundle By Name(cluster=T48 {"Filename"="", "Create?"=FALSE, "Flattened Data Strings"=[]} ("Read from File Argument"), "Filename"=w1023, "Flattened Data Strings"=w1022, "Create?"=TRUE) -> (w1020:T48)
              }
              frame "Read from File" {
                n230 = Variant To Data(type=T48 {"Filename"="", "Create?"=FALSE, "Flattened Data Strings"=[]} ("Read from File Argument"), Variant=w1031) -> (data=w1029:T48, error out=w1028:errorcluster)  [unwired: 1 in]
              }
            }
            n231 = call "Message to RT.vi"("error in (no error)"=w1013, "Message Data"=w1014, "Message"=w1016) -> ("error out"=w1018:errorcluster)  [unwired: 8 in]
          }
          frame "Read from File Rtn" {
            # "The tool returns the data from the Read from File cmd here. The payload is the XML string from the file and the error code status from the tools attempt to read the file. We broadcast the event so the main app gets it in its event loop."
            n232 = Variant To Data(error in=w1041, type=T62 {"Filename"="", "XML Strings"=[], "Error Status"={"status"=FALSE, "code"=0, "source"=""}} ("Read from File Rtn Argument"), Variant=w1042) -> (data=w1040:T62, error out=w1038:errorcluster)
            n233 = Unbundle By Name(w1040) -> ("Filename"=w1032:string, "XML Strings"=w1035:string[], "Error Status"=w1039:errorcluster)
            n234 = case shown="\"Cycle Count.xml\"" w1032 {
              selector: w1032 -> [w1043 w1049 _]
              tunnel: w1035 -> [w1048 w1050 w1060]
              tunnel: w1039 -> [w1047 w1051 _]
              tunnel: w1038 -> [w1046 w1052 w1063]
              tunnel: [w1045 w1052 w1056] -> w1037
              tunnel: w1034 -> [w1044 w1053 w1062]
              tunnel: [w1044 w1053 w1061] -> w1033
              frame Default {
                # "#ToDo: create custom error msg that includes filename."
                # "Broadcast the contents to listeners."
                n235 = call "Read from File Rtn.vi"("error in (no error)"=w1046, "error status"=w1047, "XML Strings"=w1048, "Filename"=w1043) -> ("error out"=w1045:errorcluster)  [unwired: 7 in]
              }
              frame "Verification Cal Quality Log.xml" {
                n236 = call "Read from File Rtn.vi"("error in (no error)"=w1052, "error status"=w1051, "XML Strings"=w1050, "Filename"=w1049) -> ()  [unwired: 7 in, 1 out]
              }
              frame "Cycle Count.xml" {
                # "This is from the Cycle Counter file, so just update the local parameter."
                n237 = Index Array(array=w1060) -> (element=w1054:string)  [unwired: 1 in]
                n238 = Unflatten From XML(xml string=w1054, type=T63 {"Cycle Count"=0} ("_Cycle Count File Cluster--typedef")) -> (value=w1059:T63, error out=w1055:errorcluster)  [unwired: 1 in]
                n239 = Unbundle By Name(w1059) -> ("Cycle Count"=w1057:i32)
                n240 = Bundle By Name(cluster=w1062, "Cycle Count"=w1057) -> (w1061:T8)
                n241 = Merge Errors(w1055, w1063) -> (w1056:errorcluster)
              }
            }
          }
          frame "Write to File Rtn" {
            # "11Nov19 DJS - The typedef is incorrect for what the RT system returns. Need to fix RT so that the 'XML Strings' item in the cluster is an array of strings. We are hacking it here for now."
            # "The tool returns the the error status from attempting to write to the data file. The payload is a standard error cluster. We broadcast the event so the main app gets it in its event loop."
            n242 = disable-structure shown="Disabled" {
              frame Disabled {
                (unwired) T62 {"Filename"="", "XML Strings"=[], "Error Status"={"status"=FALSE, "code"=0, "source"=""}} ("Read from File Rtn Argument")
              }
              frame Enabled {
              }
            }
            n243 = Variant To Data(error in=w1072, type=T64 {"Filename"="", "XML Strings"="", "Error Status"={"status"=FALSE, "code"=0, "source"=""}} ("Read from File Rtn Argument"), Variant=w1074) -> (data=w1071:T64, error out=w1069:errorcluster)
            n244 = Unbundle By Name(w1071) -> ("Filename"=w1066:string, "Error Status"=w1070:errorcluster)  [unwired: 1 out]
            n245 = Build Array("<***WRITE STATUS***>" ("XML String")) -> (w1065:string[])
            n246 = call "Read from File Rtn.vi"("error in (no error)"=w1069, "error status"=w1070, "XML Strings"=w1065, "Filename"=w1066) -> ("error out"=w1068:errorcluster)  [unwired: 7 in]
          }
          frame "Set Event Logger" {
            # "Sends the event logger data (path, type, etc) class to this module for use logging events."
            n247 = Variant To Data(error in=w1082, type=T46 {"EventLog.lvclass"=refnum} ("Set Event Logger Argument"), Variant=w1080) -> (data=w1078:T46, error out=w1081:errorcluster)
            n248 = Unbundle By Name(w1078) -> ("EventLog.lvclass"=w1075:refnum<class "EventLog.lvclass">)
            n249 = Bundle By Name(cluster=w1077, "EventLog.lvclass"=w1075) -> (w1076:T8)
          }
          frame "Get Device Temperature" {
            # "Send request for the device temperatures. Return will be in \"Get Device Temperature Rtn\" State."
            n250 = Unbundle By Name(w1085) -> ("STATUS.Connected"=w1084:bool)
            n251 = call "Message to RT.vi"("error in (no error)"=w1087, "Message"="Get Device Temperature", "Connected(T)"=w1084) -> ("error out"=w1086:errorcluster)  [unwired: 8 in]
          }
          frame "Get Device Temperature Rtn" {
            # "After the requested Device temperature data is returned, send a broadcast event to whoever is listening."
            n252 = Variant To Data(type=T65 {"Temp Sensors"=[], "High Thold "=[], "Low Thold "=[]} ("_Temperature All Arrays--typedef"), Variant=w1093) -> (data=w1090:T65, error out=w1089:errorcluster)  [unwired: 1 in]
            n253 = call "Device Temperature.vi"("error in (no error)"=w1089, "Device Temperature Arrays"=w1090) -> ("error out"=w1088:errorcluster)  [unwired: 9 in]
          }
          frame "Set Device Temp Thresholds" {
            # "Sets the Device Temperature Thresholds, High and Low for all the sensors."
            n254 = Variant To Data(error in=w1101, type=T49 {"Device Temp Thold Arrays"={"High Thold "=[], "Low Thold "=[]}} ("Set Device Temp Thresholds Argument"), Variant=w1100) -> (data=w1098:T49, error out=w1097:errorcluster)
            n255 = Unbundle By Name(w1098) -> ("Device Temp Thold Arrays"=w1095:T50)
            n256 = call "Message to RT.vi"("error in (no error)"=w1097, "Message Data"=w1095, "Message"="Set Temperature Thresholds") -> ()  [unwired: 8 in, 1 out]
          }
          frame "Get Cycle Count" {
            # "Get the cycle count value. If Clear is set TRUE then clear the cycle count to 0 in the tool."
            n257 = Unbundle By Name(w1106) -> ("Cycle Count"=w1105:i32)
            n258 = Variant To Data(error in=w1118, type=T51 {"Clear?"=FALSE, "Wait Notifier"=refnum} ("Get Cycle Count Argument"), Variant=w1116) -> (data=w1114:T51, error out=w1117:errorcluster)
            n259 = Unbundle By Name(w1114) -> ("Clear?"=w1102:bool, "Wait Notifier"=w1113:refnum<notifier>)
            n260 = Bundle By Name(cluster=T66 {"Cycle Count"=0, "Get Cycle Count_error"={"status"=FALSE, "code"=0, "source"=""}} ("Get Cycle Count (Reply Payload)"), "Cycle Count"=w1105, "Get Cycle Count_error"=errorcluster {"status"=FALSE, "code"=0, "source"=""} ("error constant")) -> (w1112:T66)
            n261 = case shown="True" w1102 {
              tunnel: [w1119 w1125] -> w1107
              tunnel: w1106 -> [w1119 w1124]
              tunnel: w1104 -> [_ w1122]
              tunnel: [_ w1120] -> w1103
              frame False {
              }
              frame True {
                n262 = Bundle By Name(cluster=w1124, "Cycle Count"=-1) -> (w1125:T8)
                n263 = call-poly <vilib>:"Delacor_lib_QMH_Enqueue Message (poly).vi"("Message"="Update Cycle Count", "Message Queue in"=w1122) -> ("error out"=w1120:errorcluster)  [unwired: 8 in, 1 out]
              }
            }
            n264 = Send Notification(notification=w1112, notifier=w1113) -> (error out=w1108:errorcluster)  [unwired: 1 in, 1 out]
            n265 = Merge Errors(w1103, w1108, w1117) -> (w1111:errorcluster)
          }
          frame "Return FPGA Setup Data" {
            # "If Reload is true, do not reply. Instead ask the tool to reload the FPGA setup data from its file system."
            # "Returns local copy of FPGA setup data from Tool Module."
            n266 = Variant To Data(error in=w1143, type=T52 {"Reload"=FALSE, "Wait Notifier"=refnum, "wait for reply"=FALSE} ("Return FPGA Setup Data Argument"), Variant=w1142) -> (data=w1140:T52, error out=w1130:errorcluster)
            n267 = Unbundle By Name(w1140) -> ("Reload"=w1128:bool, "Wait Notifier"=w1126:refnum<notifier>, "wait for reply"=w1132:bool)
            n268 = global read "ToolModGLOB.vi" "FPGA Setup Parameters"() -> (w1134:T28)
            n269 = global read "ToolModGLOB.vi" "Version String"() -> (w1135:string)
            n270 = case shown="True" w1128 {
              tunnel: w1130 -> [w1144 w1147]
              tunnel: [w1144 w1146] -> w1129
              frame False {
              }
              frame True {
                n271 = call "Message to RT.vi"("error in (no error)"=w1147, "Message"="Reload FPGA Setup from File") -> ("error out"=w1146:errorcluster)  [unwired: 9 in]
              }
            }
            n272 = Compound Arithmetic op=AND(invert w1128, w1132) -> (w1131:bool)
            n273 = Bundle By Name(cluster=T67 {"Version String"="", "FPGA Setup Parameters"={"FPGA Timing Constraints"={"frame.length Min"=530, "frame.ST_OFF Min"=15, "frame.ST_ON Min"=8, "frame.first data idx"=14, "frame.integ Offset"=6, "frame.integ Delay"=3, "frame.ad_latch Delay"=11, "frame.trig time Max"=0}, "FPGA Timing Ctrl"={"trig.time"=220, "integ.count 1"=400, "integ.count 2"=350, "encdr.latch ctrl"=1, "pixel.read count"=512, "clock.select"=2, "ad.clock offset"=16, "data.control reg"=2}, "FPGA Laser Config"={"laser.gain"=10, "laser.threshold Low"=1400, "laser.threshold High"=1900, "laser.dac init"=912, "laser.dac Min"=800, "laser.dac Max"=4000, "laser.config reg"=3}, "FPGA Peak Proc Cfg"={"PD.threshold"=0, "PD.width detect Min"=0, "PD.sensor pixels"=512, "PD.config reg"=23}, "FPGA SPI Cfg"={"SPI Divide Value"=1, "SPI config reg"=1}}, "Return FPGA Setup Data_error"={"status"=FALSE, "code"=0, "source"=""}} ("Return FPGA Setup Data (Reply Payload)"), "Version String"=w1135, "FPGA Setup Parameters"=w1134) -> (w1139:T67)
            n274 = case shown="True" w1131 {
              tunnel: w1126 -> [_ w1150]
              tunnel: w1139 -> [_ w1149]
              tunnel: [_ w1148] -> w1136
              frame False {
              }
              frame True {
                n275 = Send Notification(notification=w1149, notifier=w1150) -> (error out=w1148:errorcluster)  [unwired: 1 in, 1 out]
              }
            }
            n276 = Bundle By Name(cluster=w1133, "FPGA Setup Reply Notifier"=w1126) -> (w1127:T8)
            n277 = Merge Errors(w1129, w1136) -> (w1137:errorcluster)
          }
          frame "Reload FPGA Setup from File Rtn" {
            # "The tool is returning the FPGA setup data from the file system. Return it in the Notifier that was sent by the original request."
            n278 = Variant To Data(type=T68 {"Version String"="", "Mtr Ctrl Reg"=0, "FPGA Setup Parameters"={"FPGA Timing Constraints"={"frame.length Min"=530, "frame.ST_OFF Min"=15, "frame.ST_ON Min"=8, "frame.first data idx"=14, "frame.integ Offset"=6, "frame.integ Delay"=3, "frame.ad_latch Delay"=11, "frame.trig time Max"=0}, "FPGA Timing Ctrl"={"trig.time"=220, "integ.count 1"=400, "integ.count 2"=350, "encdr.latch ctrl"=1, "pixel.read count"=512, "clock.select"=2, "ad.clock offset"=16, "data.control reg"=2}, "FPGA Laser Config"={"laser.gain"=10, "laser.threshold Low"=1400, "laser.threshold High"=1900, "laser.dac init"=912, "laser.dac Min"=800, "laser.dac Max"=4000, "laser.config reg"=3}, "FPGA Peak Proc Cfg"={"PD.threshold"=0, "PD.width detect Min"=0, "PD.sensor pixels"=512, "PD.config reg"=23}, "FPGA SPI Cfg"={"SPI Divide Value"=1, "SPI config reg"=1}}} ("_FPGA Return Setup Data Cluster--typedef"), Variant=w1160) -> (data=w1158:T68, error out=w1152:errorcluster)  [unwired: 1 in]
            n279 = Unbundle By Name(w1162) -> ("FPGA Setup Reply Notifier"=w1161:refnum<notifier>)
            n280 = Unbundle By Name(w1158) -> ("Version String"=w1155:string, "FPGA Setup Parameters"=w1154:T28)
            n281 = Bundle By Name(cluster=T67 {"Version String"="", "FPGA Setup Parameters"={"FPGA Timing Constraints"={"frame.length Min"=530, "frame.ST_OFF Min"=15, "frame.ST_ON Min"=8, "frame.first data idx"=14, "frame.integ Offset"=6, "frame.integ Delay"=3, "frame.ad_latch Delay"=11, "frame.trig time Max"=0}, "FPGA Timing Ctrl"={"trig.time"=220, "integ.count 1"=400, "integ.count 2"=350, "encdr.latch ctrl"=1, "pixel.read count"=512, "clock.select"=2, "ad.clock offset"=16, "data.control reg"=2}, "FPGA Laser Config"={"laser.gain"=10, "laser.threshold Low"=1400, "laser.threshold High"=1900, "laser.dac init"=912, "laser.dac Min"=800, "laser.dac Max"=4000, "laser.config reg"=3}, "FPGA Peak Proc Cfg"={"PD.threshold"=0, "PD.width detect Min"=0, "PD.sensor pixels"=512, "PD.config reg"=23}, "FPGA SPI Cfg"={"SPI Divide Value"=1, "SPI config reg"=1}}, "Return FPGA Setup Data_error"={"status"=FALSE, "code"=0, "source"=""}} ("Return FPGA Setup Data (Reply Payload)"), "Version String"=w1155, "FPGA Setup Parameters"=w1154) -> (w1156:T67)
            n282 = Send Notification(notification=w1156, notifier=w1161) -> (error out=w1151:errorcluster)  [unwired: 1 in, 1 out]
            n283 = Merge Errors(w1152, w1151) -> (w1153:errorcluster)
          }
          frame "Update FPGA Setup Data" {
            # "Updates the FPGA Setup Data in either the Tool working copy or as well to the Tool File non-volitile File System (if Commit==T)."
            n284 = Unbundle By Name(w1166) -> ("FW Ver Maj/Min"=w1165:dbl)
            n285 = Variant To Data(type=T53 {"Commit"=FALSE, "FPGA Setup Parameters"={"FPGA Timing Constraints"={"frame.length Min"=530, "frame.ST_OFF Min"=15, "frame.ST_ON Min"=8, "frame.first data idx"=14, "frame.integ Offset"=6, "frame.integ Delay"=3, "frame.ad_latch Delay"=11, "frame.trig time Max"=0}, "FPGA Timing Ctrl"={"trig.time"=220, "integ.count 1"=400, "integ.count 2"=350, "encdr.latch ctrl"=1, "pixel.read count"=512, "clock.select"=2, "ad.clock offset"=16, "data.control reg"=2}, "FPGA Laser Config"={"laser.gain"=10, "laser.threshold Low"=1400, "laser.threshold High"=1900, "laser.dac init"=912, "laser.dac Min"=800, "laser.dac Max"=4000, "laser.config reg"=3}, "FPGA Peak Proc Cfg"={"PD.threshold"=0, "PD.width detect Min"=0, "PD.sensor pixels"=512, "PD.config reg"=23}, "FPGA SPI Cfg"={"SPI Divide Value"=1, "SPI config reg"=1}}} ("Update FPGA Setup Data Argument"), Variant=w1174) -> (data=w1172:T53, error out=w1170:errorcluster)  [unwired: 1 in]
            n286 = Unbundle By Name(w1172) -> ("Commit"=w1168:bool, "FPGA Setup Parameters"=w1169:T28)
            n287 = Greater Or Equal?(x=w1165, y=1.7) -> (x >= y?=w1163:bool)
            n288 = case shown="False" w1163 {
              tunnel: [w1176 w1180] -> w1171
              tunnel: w1168 -> [w1175 w1179]
              frame True {
                # "New version commands after RT V1.7.x"
                n289 = Select(t="Commit FPGA Setup to File", s=w1175, f="Push FPGA Setup to Tool" ("Message")) -> (s? t:f=w1176:string)
              }
              frame False {
                # "Old versions"
                n290 = Select(t="Commit FPGA Setup Params", s=w1179, f="Set Cur FPGA Setup" ("Message")) -> (s? t:f=w1180:string)
              }
            }
            n291 = call "Message to RT.vi"("error in (no error)"=w1170, "Message Data"=w1169, "Message"=w1171) -> ("error out"=w1167:errorcluster)  [unwired: 8 in]
            n292 = case shown="No Error" w1167 {
              tunnel: w1169 -> [w1183 _]
              frame No Error {
                n293 = global write "ToolModGLOB.vi" "FPGA Setup Parameters"(w1183) -> ()
              }
              frame Error {
              }
            }
          }
          frame "------- Tool Connection State Sequence -------" {
            # "These states do the work of interfacing with the tool."
            n294 = Merge Errors(w1186) -> (w1184:errorcluster)
          }
          frame "Connect: Get Version" {
            w1190 = TRUE  # Enqueue Next State
            w1193 = 1000  # Period
            w1194 = -1  # Count
            w1195 = 3  # Timer ID
            # "Start a 1 sec repeating timer to get the tool temperatures. When the timer expires, it will enqueue the \"Get Device Temperature\" state."
            # "Start the Tool Status Reader Helper Loop reading data so that when we finish getting all the tool info, there will be good tool status data available."
            # "Send the Get Firmware Version command.  Wait for the Get Firmware Version Rtn message back from the tool."
            n295 = Unbundle By Name(w1202) -> ("EventLog.lvclass"=w1201:refnum<class "EventLog.lvclass">)
            n296 = call "Message to RT.vi"("error in (no error)"=w1189, "Message"="Get Firmware Version") -> ("error out"=w1188:errorcluster)  [unwired: 9 in]
            n297 = call "Log General Event Helper.vi"("State Info"=w1200, "EventLog in"=w1201) -> ("error out"=w1199:errorcluster)  [unwired: 8 in, 1 out]
            n298 = call "Tool Status Reader Cmd.vi"("error in (no error)"=w1188, "Command"=_Host_-_HS_Data_Stream_State_Enum_Typedef."Receive Data") -> ("error out"=w1197:errorcluster)  [unwired: 9 in]
            n299 = call "Setup Timer.vi"("Enqueue Next State"=w1190, "Timer ID"=w1195, "Next State"="Get Device Temperature", "error in (no error)"=w1197, "Count"=w1194, "Period"=w1193, "Timer On"=TRUE) -> ("error out"=w1196:errorcluster)  [unwired: 4 in]
            n300 = Merge Errors(w1199, w1196) -> (w1203:errorcluster)
          }
          frame "Get Firmware Version Rtn" {
            n301 = Variant To Data(type="", Variant=w1216) -> (data=w1205:string, error out=w1212:errorcluster)  [unwired: 1 in]
            n302 = Unbundle By Name(w1210) -> ("EventLog.lvclass"=w1207:refnum<class "EventLog.lvclass">)
            n303 = Fract/Exp String To Number(string=w1205) -> (number=w1208:dbl)  [unwired: 3 in, 1 out]
            n304 = call "Set Firmware Version.vi"("Firmware Version String"=w1205) -> ()  [unwired: 11 in]
            n305 = case shown="No Error" w1212 {
              selector: w1212 -> [w1220 w1225]
              tunnel: w1217 -> [w1223 _]
              tunnel: [w1222 w1224] -> w1214
              tunnel: [TRUE _] -> w1211
              tunnel: w1207 -> [_ w1226]
              frame No Error {
                w1218 = TRUE  # Init
                n306 = call-poly <vilib>:"Delacor_lib_QMH_Enqueue Message (poly).vi"("error in (no error)"=w1220, "Message Data"=w1218, "Message"="Connect: Retrieve Tool Config", "Message Queue in"=w1223) -> ("error out"=w1222:errorcluster)  [unwired: 6 in, 1 out]
              }
              frame Error {
                n307 = call "Error Event.vi"("error in (no error)"=w1225, "EventLog ref"=w1226) -> ("error out"=w1224:errorcluster)  [unwired: 8 in, 1 out]
              }
            }
            n308 = call "Log General Event Helper.vi"("Payload"=w1205, "State Info"=w1204, "EventLog in"=w1207) -> ("error out"=w1206:errorcluster)  [unwired: 7 in, 1 out]
            n309 = Bundle By Name(cluster=w1210, "FW Ver Maj/Min"=w1208, "Got FW Ver"=w1211) -> (w1213:T8)
            n310 = Merge Errors(w1206, w1214) -> (w1209:errorcluster)
          }
          frame "Connect: Retrieve Tool Config" {
            w1236 = FALSE  # Init
            n311 = Unbundle By Name(w1233) -> ("EventLog.lvclass"=w1230:refnum<class "EventLog.lvclass">)
            n312 = Variant To Data(type=w1236, Variant=w1237) -> (data=w1232:bool, error out=w1235:errorcluster)  [unwired: 1 in]
            n313 = call "wait (ms) with error clusters.vi"("error in (no error)"=w1235, "milliseconds to wait"=u32 1000) -> ("error out"=w1241:errorcluster)  [unwired: 9 in]
            n314 = Format Into String(format string="Got Tool Config?=%s", w1232) -> (resulting string=w1228:string)  [unwired: 2 in, 1 out]
            n315 = call "Message to RT.vi"("error in (no error)"=w1241, "Message"="Retrieve Tool Config") -> ("error out"=w1239:errorcluster)  [unwired: 9 in]
            n316 = case shown="True" w1232 {
              tunnel: w1239 -> [w1244 w1248]
              tunnel: [w1244 w1247] -> w1238
              tunnel: "Connect: Wait for Tool Cfg" ("Timer 2 Call State") -> [_ w1245]
              frame False {
              }
              frame True {
                n317 = call "Setup Delay for Next State.vi"("error in (no error)"=w1248, "Period"=1000, "Next State"=w1245) -> ("error out"=w1247:errorcluster)  [unwired: 8 in]
              }
            }
            n318 = call "Log General Event Helper.vi"("Payload"=w1228, "State Info"=w1229, "EventLog in"=w1230) -> ("error out"=w1243:errorcluster)  [unwired: 7 in, 1 out]
            n319 = Merge Errors(w1238, w1243) -> (w1234:errorcluster)
          }
          frame "Connect: Wait for Tool Cfg" {
            n320 = Unbundle By Name(w1259) -> ("EventLog.lvclass"=w1253:refnum<class "EventLog.lvclass">, "Got Tool Type"=w1255:bool)
            n321 = case shown="False" w1255 {
              tunnel: w1258 -> [w1264 w1265]
              tunnel: [w1263 w1265] -> w1257
              tunnel: w1256 -> [w1262 _]
              frame False {
                # "Haven't gotten the return Tool Config data, so request again."
                n322 = call-poly <vilib>:"Delacor_lib_QMH_Enqueue Message (poly).vi"("error in (no error)"=w1264, "Message Data"=FALSE, "Message"="Connect: Retrieve Tool Config", "Message Queue in"=w1262) -> ("error out"=w1263:errorcluster)  [unwired: 6 in, 1 out]
              }
              frame True {
                # "We do nothing."
                # "This case handles when we've already gotten the Tool Cfg stuff but there is still a \"Wait for Tool Cfg\" state in the timer queue."
              }
            }
            n323 = Format Into String(format string="Got Tool Type=%s", w1255) -> (resulting string=w1251:string)  [unwired: 2 in, 1 out]
            n324 = call "Log General Event Helper.vi"("Payload"=w1251, "State Info"=w1252, "EventLog in"=w1253) -> ("error out"=w1249:errorcluster)  [unwired: 7 in, 1 out]
            n325 = Merge Errors(w1257, w1249) -> (w1250:errorcluster)
          }
          frame "Retrieve Tool Config Rtn" {
            n326 = Unbundle By Name(w1285) -> ("EventLog.lvclass"=w1270:refnum<class "EventLog.lvclass">, "Connecting"=w1268:bool)
            n327 = Variant To Data(type=T69 {"Config Cluster Version"="", "Product Name"="", "Tool Config Cluster"={"Tool Type"=0, "Tool SN"=0, "Tool Block"={"Encoder Size"=0, "Encoder Scale"=0, "Encoder Offset"=0, "MaxEncoder"=0, "MinEncoder"=0, "Start Delay"=0.0, "Tool Face Ref"=0.0}, "Motor Block"={"MinMotor Speed"=0, "MaxMotor Speed"=0, "Homing Speed"=0, "Jog Speed"=0, "Inspect Speed"=0, "VBlk Speed"=0, "CleaningPos"=0, "Safe Zone"=0, "Has Motor"=FALSE, "Use Home Index"=FALSE}, "Verification Block"={"Angle"=0.0, "FlankLength1"=0.0, "FlankLength2"=0.0, "Location"=0.0, "Serial Number"=0}, "Probe Block"={"nProbes"=0, "Probe Param Array"=[]}}} ("output cluster"), Variant=w1277) -> (data=w1273:T69, error out=w1288:errorcluster)  [unwired: 1 in]
            n328 = Unbundle By Name(w1273) -> ("Tool Config Cluster"=w1272:T35, "Config Cluster Version"=w1275:string, "Product Name"=w1274:string)
            n329 = case shown="True" w1268 {
              selector: w1268 -> [w1307 w1314]
              tunnel: w1285 -> [w1308 w1316]
              tunnel: [w1308 w1315] -> w1280
              tunnel: [w1307 w1314] -> w1284
              tunnel: [_ w1313] -> w1267
              tunnel: w1272 -> [_ w1311]
              tunnel: w1275 -> [_ w1310]
              tunnel: w1274 -> [_ w1309]
              frame False {
              }
              frame True {
                # "If connecting, then first get tool type. Check that it is the right type."
                n330 = call "Check Tool Type.vi"("Tool Config Cluster"=w1311) -> ("Success"=w1312:bool, "Tool Type"=w1313:u16)  [unwired: 9 in]
                n331 = Bundle By Name(cluster=w1316, "Got Tool Type"=w1312) -> (w1315:T8)
                n332 = call "Set Config Cluster Version.vi"("Config Cluster Version"=w1310) -> ()  [unwired: 11 in]
                n333 = call "Set Product Name.vi"("Product Name"=w1309) -> ()  [unwired: 11 in]
                n334 = call "Set Tool Type.vi"("Tool Type"=w1313) -> ()  [unwired: 11 in]
              }
            }
            n335 = To Variant(anything=w1272) -> (Variant=w1271:variant)
            n336 = call "Get Op Cfg.vi"() -> ("Tool Operation Config"=w1283:T72)  [unwired: 11 in]
            n337 = call "Log Tool Config Rtn Event Helper.vi"("State Info"=w1269, "Tool Type"=w1267, "Connecting"=w1268, "EventLog in"=w1270) -> ("error out"=w1266:errorcluster)  [unwired: 6 in, 1 out]
            n338 = call "Init Config Data.vi"("error in (no error)"=w1288, "Config Data in"=w1271, "Tool Operation Config"=w1283) -> ("error out"=w1281:errorcluster, "Tool Op Cfg out"=w1282:T72)  [unwired: 7 in]
            n339 = case shown="No Error" w1281 {
              selector: w1281 -> [w1289 w1306]
              tunnel: w1287 -> [w1295 _]
              tunnel: [w1294 w1306] -> w1286
              tunnel: w1284 -> [w1293 _]
              tunnel: w1282 -> [w1292 _]
              tunnel: w1280 -> [w1291 w1305]
              tunnel: [w1290 w1305] -> w1279
              frame No Error {
                n340 = case shown="True" w1293 {
                  tunnel: w1295 -> [_ w1303]
                  tunnel: [w1296 w1304] -> w1294
                  tunnel: w1292 -> [_ w1302]
                  tunnel: w1291 -> [w1297 w1300]
                  tunnel: [w1297 w1299] -> w1290
                  tunnel: w1289 -> [w1296 _]
                  frame False {
                  }
                  frame True {
                    n341 = Bundle By Name(cluster=w1300, "Got Tool Cfg"=TRUE) -> (w1299:T8)
                    n342 = call-poly <vilib>:"Delacor_lib_QMH_Enqueue Message (poly).vi"("Message Data"=w1302, "Message"="Connect: Config Probes", "Message Queue in"=w1303) -> ("error out"=w1304:errorcluster)  [unwired: 7 in, 1 out]
                  }
                }
              }
              frame Error {
              }
            }
            n343 = Merge Errors(w1286, w1266) -> (w1278:errorcluster)
          }
          frame "Connect: Config Probes" {
            n344 = call "Get Op Cfg.vi"() -> ("Tool Operation Config"=w1331:T72)  [unwired: 11 in]
            n345 = Unbundle By Name(w1327) -> ("EventLog.lvclass"=w1319:refnum<class "EventLog.lvclass">, "Connecting"=w1325:bool)
            n346 = Variant To Data(type=w1331, Variant=w1329) -> (data=w1328:T72, error out=w1330:errorcluster)  [unwired: 1 in]
            n347 = call "Configure Probe.vi"("error in (no error)"=w1330, "Tool Operation Config"=w1328) -> ("error out"=w1323:errorcluster)  [unwired: 8 in, 1 out]
            n348 = case shown="True" w1325 {
              tunnel: [w1332 w1335] -> w1322
              tunnel: w1323 -> [w1332 w1333]
              frame False {
              }
              frame True {
                n349 = case shown="No Error" w1333 {
                  selector: w1333 -> [w1337 w1340]
                  tunnel: "Get Data Stream Format Params" ("Message") -> [w1339 _]
                  tunnel: [w1338 w1340] -> w1335
                  tunnel: [TRUE _] -> _
                  frame No Error {
                    n350 = call "Message to RT.vi"("error in (no error)"=w1337, "Message"=w1339) -> ("error out"=w1338:errorcluster)  [unwired: 9 in]
                  }
                  frame Error {
                  }
                }
              }
            }
            n351 = Format Into String(format string="Connecting=%s, ", w1325) -> (resulting string=w1317:string)  [unwired: 2 in, 1 out]
            n352 = call "Log General Event Helper.vi"("Payload"=w1317, "State Info"=w1318, "EventLog in"=w1319) -> ("error out"=w1320:errorcluster)  [unwired: 7 in, 1 out]
            n353 = call "Error Event.vi"("error in (no error)"=w1322, "EventLog ref"=w1319) -> ("error out"=w1321:errorcluster)  [unwired: 8 in, 1 out]
            n354 = Merge Errors(w1320, w1321) -> (w1326:errorcluster)
          }
          frame "Data Stream Format Params Rtn" {
            # "Reads the FPGA setup parameters file from the Tool File system and save to local copy."
            n355 = Variant To Data(type=T70 {"Samples per Block"=20, "Raw Data Status Len"=0, "Fltr Data Status Len"=0} ("_Acq  Process Params Cluster--typedef"), Variant=w1356) -> (data=w1354:T70, error out=w1349:errorcluster)  [unwired: 1 in]
            n356 = case shown="No Error" w1349 {
              tunnel: w1354 -> [w1362 _]
              tunnel: [TRUE _] -> w1351
              frame No Error {
                n357 = global write "ToolModGLOB.vi" "Data Stream Fmt Params"(w1362) -> ()
              }
              frame Error {
              }
            }
            n358 = Unbundle By Name(w1350) -> ("EventLog.lvclass"=w1346:refnum<class "EventLog.lvclass">, "Connecting"=w1347:bool)
            n359 = call "Error Event.vi"("error in (no error)"=w1349, "EventLog ref"=w1346) -> ("error out"=w1343:errorcluster)  [unwired: 8 in, 1 out]
            n360 = case shown="True" w1347 {
              tunnel: w1357 -> [_ w1359]
              tunnel: w1351 -> [_ _]
              tunnel: [_ w1358] -> w1342
              frame False {
              }
              frame True {
                n361 = call-poly <vilib>:"Delacor_lib_QMH_Enqueue Message (poly).vi"("Message"="Get Cur FPGA Setup", "Message Queue in"=w1359) -> ("error out"=w1358:errorcluster)  [unwired: 8 in, 1 out]
              }
            }
            n362 = Format Into String(format string="Connecting=%s, ", w1347) -> (resulting string=w1345:string)  [unwired: 2 in, 1 out]
            n363 = call "Log General Event Helper.vi"("Payload"=w1345, "State Info"=w1344, "EventLog in"=w1346) -> ("error out"=w1341:errorcluster)  [unwired: 7 in, 1 out]
            n364 = Bundle By Name(cluster=w1350, "Got Fmt Params"=w1351) -> (w1353:T8)
            n365 = Merge Errors(w1343, w1342, w1341) -> (w1352:errorcluster)
          }
          frame "Get Cur FPGA Setup" {
            # "Reads the FPGA setup parameters file from the Tool File system and save to local copy."
            n366 = Unbundle By Name(w1380) -> ("EventLog.lvclass"=w1365:refnum<class "EventLog.lvclass">, "Connecting"=w1377:bool, "STATUS.Connected"=w1376:bool, "FW Ver Maj/Min"=w1368:dbl)
            n367 = Greater Or Equal?(x=w1368, y=1.7) -> (x >= y?=w1369:bool)
            n368 = Select(t="Pull FPGA Setup from Tool" ("Message"), s=w1369, f="Get Cur FPGA Setup" ("Message")) -> (s? t:f=w1371:string)
            n369 = Or(x=w1377, y=w1376) -> (x .or. y?=w1379:bool)
            n370 = Format Into String(format string="Connecting=%s, Connected=%s", w1377, w1376) -> (resulting string=w1364:string)  [unwired: 2 in, 1 out]
            n371 = case shown="True" w1379 {
              tunnel: [_ w1383] -> w1375
              tunnel: w1371 -> [_ w1382]
              frame False {
              }
              frame True {
                n372 = call "Message to RT.vi"("Message"=w1382) -> ("error out"=w1383:errorcluster)  [unwired: 10 in]
              }
            }
            n373 = call "Log General Event Helper.vi"("Payload"=w1364, "State Info"=w1363, "EventLog in"=w1365) -> ("error out"=w1367:errorcluster, "EventLog out"=w1366:refnum<class "EventLog.lvclass">)  [unwired: 7 in]
            n374 = call "Error Event.vi"("error in (no error)"=w1375, "EventLog ref"=w1366) -> ("error out"=w1374:errorcluster)  [unwired: 8 in, 1 out]
            n375 = Merge Errors(w1367, w1374) -> (w1381:errorcluster)
          }
          frame "Get Cur FPGA Setup Rtn", "Pull FPGA Setup from Tool Rtn" {
            # "The return data from the this request. If no error, save the data and go to the 'Connected' state."
            n376 = Variant To Data(type=T68 {"Version String"="", "Mtr Ctrl Reg"=0, "FPGA Setup Parameters"={"FPGA Timing Constraints"={"frame.length Min"=530, "frame.ST_OFF Min"=15, "frame.ST_ON Min"=8, "frame.first data idx"=14, "frame.integ Offset"=6, "frame.integ Delay"=3, "frame.ad_latch Delay"=11, "frame.trig time Max"=0}, "FPGA Timing Ctrl"={"trig.time"=220, "integ.count 1"=400, "integ.count 2"=350, "encdr.latch ctrl"=1, "pixel.read count"=512, "clock.select"=2, "ad.clock offset"=16, "data.control reg"=2}, "FPGA Laser Config"={"laser.gain"=10, "laser.threshold Low"=1400, "laser.threshold High"=1900, "laser.dac init"=912, "laser.dac Min"=800, "laser.dac Max"=4000, "laser.config reg"=3}, "FPGA Peak Proc Cfg"={"PD.threshold"=0, "PD.width detect Min"=0, "PD.sensor pixels"=512, "PD.config reg"=23}, "FPGA SPI Cfg"={"SPI Divide Value"=1, "SPI config reg"=1}}} ("_FPGA Return Setup Data Cluster--typedef"), Variant=w1400) -> (data=w1399:T68, error out=w1396:errorcluster)  [unwired: 1 in]
            n377 = Unbundle By Name(w1399) -> ("Version String"=w1388:string, "Mtr Ctrl Reg"=w1395:u16, "FPGA Setup Parameters"=w1394:T28)
            n378 = Unbundle By Name(w1393) -> ("EventLog.lvclass"=w1391:refnum<class "EventLog.lvclass">, "Connecting"=w1390:bool)
            n379 = case shown="No Error" w1396 {
              tunnel: [TRUE _] -> w1387
              tunnel: w1395 -> [w1407 _]
              tunnel: w1388 -> [w1408 _]
              tunnel: w1394 -> [w1406 _]
              frame No Error {
                n380 = global write "ToolModGLOB.vi" "Version String"(w1408) -> ()
                n381 = global write "ToolModGLOB.vi" "Mtr Ctrl Reg(File)"(w1407) -> ()
                n382 = global write "ToolModGLOB.vi" "FPGA Setup Parameters"(w1406) -> ()
              }
              frame Error {
              }
            }
            n383 = case shown="True" w1390 {
              tunnel: w1401 -> [_ w1405]
              tunnel: [_ w1403] -> w1397
              tunnel: w1387 -> [_ w1402]
              frame False {
              }
              frame True {
                n384 = call-poly <vilib>:"Delacor_lib_QMH_Enqueue Message (poly).vi"("Message Data"=w1402, "Message"="Connected", "Message Queue in"=w1405) -> ("error out"=w1403:errorcluster)  [unwired: 7 in, 1 out]
              }
            }
            n385 = Format Into String(format string="Connecting=%s, Success=%s, Version String=%s", w1390, w1387, w1388) -> (resulting string=w1386:string)  [unwired: 2 in, 1 out]
            n386 = call "Log General Event Helper.vi"("Payload"=w1386, "State Info"=w1392, "EventLog in"=w1391) -> ("error out"=w1385:errorcluster)  [unwired: 7 in, 1 out]
            n387 = Merge Errors(w1397, w1396, w1385) -> (w1398:errorcluster)
          }
          frame "Connected" {
            w1415 = FALSE  # Connected
            # "Create cycle count file if it doesn't exist with value set to 0."
            # "There is a connection to the tool AND all necessary information has been retrieved from the tool. Set the 'Conncted' and 'Got FPGA Setup' flags, and clear the 'Connecting' flag (we are done connecting and are connected). We broadcast a conected event (if anyone wants it) and request the tool cycle count and go check if the tool is in the ready state."
            n388 = Variant To Data(type=w1415, Variant=w1429) -> (data=w1413:bool, error out=w1411:errorcluster)  [unwired: 1 in]
            n389 = call "Cycle Count XML Default Text.vi"() -> ("Cycle Counter XML String"=w1421:string)  [unwired: 11 in]
            n390 = Build Array(w1421) -> (w1418:string[])
            n391 = Bundle By Name(cluster=T48 {"Filename"="Cycle Count.xml", "Create?"=FALSE, "Flattened Data Strings"=[]} ("Read from File Argument"), "Filename"="Cycle Count.xml", "Create?"=TRUE, "Flattened Data Strings"=w1418) -> (w1420:T48)
            n392 = Unbundle By Name(w1424) -> ("EventLog.lvclass"=w1410:refnum<class "EventLog.lvclass">, "Connecting"=w1412:bool)
            n393 = case shown="True" w1412 {
              tunnel: w1430 -> [_ w1435]
              tunnel: [_ w1448] -> w1427
              tunnel: w1413 -> [_ w1441]
              tunnel: [_ w1436] -> w1426
              tunnel: w1424 -> [w1431 w1443]
              tunnel: [w1431 w1442] -> w1425
              tunnel: [_ w1440] -> w1417
              tunnel: w1420 -> [_ w1438]
              tunnel: w1411 -> [_ _]
              frame False {
              }
              frame True {
                # "Get Cycle Count"
                # "Update Status Immediately"
                n394 = call "Get Tool Type and SN.vi"() -> ("Tool SN"=w1445:u16, "Tool Type"=w1446:u16)  [unwired: 10 in]
                n395 = call-poly <vilib>:"Delacor_lib_QMH_Enqueue Message (poly).vi"("Message"="Check if Ready", "Message Queue in"=w1435) -> ("error out"=w1433:errorcluster)  [unwired: 8 in, 1 out]
                n396 = Bundle By Name(cluster=w1443, "Got FPGA Setup"=w1441, "STATUS.Connected"=w1441, "Connecting"=FALSE) -> (w1442:T8)
                n397 = Bundle By Name(cluster=T58 {"Connected"=FALSE, "Tool Type"=0, "Tool SN"=0} ("Connected Argument"), "Connected"=w1441, "Tool Type"=w1446, "Tool SN"=w1445) -> (w1440:T58)
                n398 = call "Message to RT.vi"("error in (no error)"=w1433, "Message Data"=w1438, "Message"="Read from File") -> ("error out"=w1432:errorcluster)  [unwired: 8 in]
                n399 = call "Connected.vi"("Connected Argument"=w1440) -> ("error out"=w1448:errorcluster)  [unwired: 10 in]
                n400 = call "Time Expired.vi"("error in (no error)"=w1432, "ID"=1 ("Timer ID")) -> ("error out"=w1436:errorcluster)  [unwired: 9 in]
              }
            }
            n401 = call "Log Connect Event Helper.vi"("Connected Argument"=w1417, "State Info"=w1414, "Connecting"=w1412, "Connected"=w1413, "EventLog in"=w1410) -> ("error out"=w1416:errorcluster)  [unwired: 5 in, 1 out]
            n402 = Merge Errors(w1427, w1426, w1416) -> (w1428:errorcluster)
          }
          frame "Check if Ready" {
            # "has motor?"
            # "After connecting and flashing the mode LED, check if tool has a motor. If so, wait for home command from main app. Otherwise go to 'Ready'."
            n403 = Unbundle By Name(w1458) -> ("STATUS.Status"=w1455:u16, "STATUS.MC SM State"=w1454:u16, "STATUS.M_Ctrl"=w1453:u16)
            n404 = Unbundle By Name(w1458) -> ("EventLog.lvclass"=w1452:refnum<class "EventLog.lvclass">)
            n405 = call "Get Has Motor.vi"() -> ("Has Motor"=w1457:bool)  [unwired: 11 in]
            n406 = call "Check Home Init Status.vi"("Status Byte"=w1455) -> ("Home Init?"=w1456:bool)  [unwired: 14 in]
            n407 = Compound Arithmetic op=OR(invert w1457, w1456) -> (w1460:bool)
            n408 = case shown="True" w1460 {
              tunnel: w1463 -> [w1465 w1469]
              tunnel: w1462 -> [_ w1468]
              tunnel: [w1465 w1467] -> w1464
              frame False {
                # "If tool has motor and home is not set then we wait for main app to send home command."
              }
              frame True {
                # "Tool has no motor  OR\nHome bit is already set."
                n409 = call-poly <vilib>:"Delacor_lib_QMH_Enqueue Message (poly).vi"("error in (no error)"=w1469, "Message"="Ready", "Message Queue in"=w1468) -> ("error out"=w1467:errorcluster)  [unwired: 7 in, 1 out]
              }
            }
            n410 = Format Into String(format string="Has Motor=%s, Home Init=%s, Status=%x, MC SM State=%x, M_Ctrl=%x", w1457, w1456, w1455, w1454, w1453) -> (resulting string=w1451:string)  [unwired: 2 in, 1 out]
            n411 = call "Log General Event Helper.vi"("Payload"=w1451, "State Info"=w1449, "EventLog in"=w1452) -> ("error out"=w1450:errorcluster)  [unwired: 7 in, 1 out]
            n412 = Merge Errors(w1464, w1450) -> (w1461:errorcluster)
          }
          frame "Ready" {
            # "If Tool is now ready to receive commands, take data, etc. Set the ready bit in the STATUS cluster. This will be broadcast to the Main App from the Update Status state."
            n413 = Unbundle By Name(w1475) -> ("STATUS"=w1480:T9, "EventLog.lvclass"=w1471:refnum<class "EventLog.lvclass">)
            n414 = Unbundle By Name(w1480) -> ("Initialized"=w1477:bool, "Connected"=w1476:bool, "Status"=w1474:u16)
            n415 = Compound Arithmetic op=AND(w1477, w1476) -> (w1479:bool)
            n416 = case shown="True" w1479 {
              tunnel: w1480 -> [w1483 w1486]
              tunnel: [w1483 w1484] -> w1481
              frame False {
              }
              frame True {
                n417 = Bundle By Name(cluster=w1486, "Ready"=TRUE) -> (w1484:T9)
              }
            }
            n418 = Format Into String(format string="Initialized=%s, Connected=%s, Status=%x", w1477, w1476, w1474) -> (resulting string=w1472:string)  [unwired: 2 in, 1 out]
            n419 = call "Log General Event Helper.vi"("Payload"=w1472, "State Info"=w1470, "EventLog in"=w1471) -> ("error out"=w1473:errorcluster)  [unwired: 7 in, 1 out]
            n420 = Bundle By Name(cluster=w1475, "STATUS"=w1481) -> (w1482:T8)
          }
          frame "Homing: Check Home Off" {
            w1505 = TRUE  # Ignore Limit Switches?
            # "7Nov16-DJS Added delay because Home bit goes high before the back and forth homing motion is finished. After Ready goes to Monitor state, the Read Encoder vi was timing out cause the homing wasn't finished."
            # "Wait for the Home Init status bit to go False.  We do this so we don't see a false positive. We wait for it to go off, then wait for it to come back on when home operation is complete."
            n421 = Unbundle By Name(w1492) -> ("Loop Counter"=w1497:i32, "STATUS.Status"=w1502:u16, "Encoder Count"=w1500:i32, "STATUS.MC SM State"=w1496:u16, "STATUS.M_Ctrl"=w1495:u16, "EventLog.lvclass"=w1508:refnum<class "EventLog.lvclass">)
            n422 = call "Check Homing Status V2.vi"("Ignore Limit Switches?"=w1505, "Prev Encoder"=w1500, "error in (no error)"=w1506, "Status Byte in"=w1502, "Homing Count in"=w1497) -> ("error out"=w1499:errorcluster, "Homing Count Out"=w1509:i32, "Home Complete"=w1503:bool)  [unwired: 4 in]
            n423 = case shown="True" w1503 {
              tunnel: [w1512 w1515] -> w1490
              tunnel: w1507 -> [w1511 _]
              tunnel: w1487 -> [_ w1513]
              frame False {
                n424 = call-poly <vilib>:"Delacor_lib_QMH_Enqueue Message (poly).vi"("Message"="Homing: Check Status", "Message Queue in"=w1511) -> ("error out"=w1512:errorcluster)  [unwired: 8 in, 1 out]
              }
              frame True {
                n425 = call "Setup Delay for Next State.vi"("Period"=1000, "Next State"=w1513) -> ("error out"=w1515:errorcluster)  [unwired: 9 in]
              }
            }
            n426 = Unbundle By Name(w1499) -> ("code"=w1498:i32)
            n427 = Format Into String(format string="Home Complete=%s, Loop Counter=%d, Status=%x, Encoder=%d, Error=%d\n, MC SM State=%x, M_Ctrl=%x", w1503, w1497, w1502, w1500, w1498, w1496, w1495) -> (resulting string=w1494:string)  [unwired: 2 in, 1 out]
            n428 = call "Error Event.vi"("error in (no error)"=w1499, "EventLog ref"=w1508) -> ("error out"=w1489:errorcluster, "EventLog ref"=w1491:refnum<class "EventLog.lvclass">)  [unwired: 8 in]
            n429 = Bundle By Name(cluster=w1492, "Loop Counter"=w1509) -> (w1493:T8)
            n430 = call "Log General Event Helper.vi"("Payload"=w1494, "State Info"=w1487, "EventLog in"=w1491) -> ("error out"=w1488:errorcluster)  [unwired: 7 in, 1 out]
            n431 = Merge Errors(w1490, w1489, w1488) -> (w1504:errorcluster)
          }
          frame "Homing: Check Status" {
            w1536 = TRUE  # Ignore Limit Switches?
            # "After waiting for the Home Init bit to go false, we now wait until it goes True, indicating the homing has complete."
            n432 = Unbundle By Name(w1532) -> ("EventLog.lvclass"=w1517:refnum<class "EventLog.lvclass">)
            n433 = Unbundle By Name(w1532) -> ("Loop Counter"=w1524:i32, "STATUS.Status"=w1528:u16, "Encoder Count"=w1525:i32, "STATUS.MC SM State"=w1520:u16, "STATUS.M_Ctrl"=w1519:u16, "Prev. Encdr"=w1526:i32)
            n434 = call "Check Homing Status V2.vi"("Ignore Limit Switches?"=w1536, "Prev Encoder"=w1526, "error in (no error)"=w1537, "Status Byte in"=w1528, "Homing Count in"=w1524, "New Encoder"=w1525) -> ("error out"=w1527:errorcluster, "Homing Count Out"=w1529:i32, "Home Complete"=w1530:bool)  [unwired: 3 in]
            n435 = Unbundle By Name(w1527) -> ("code"=w1521:i32, "status"=w1522:bool)
            n436 = Or(x=w1530, y=w1522) -> (x .or. y?=w1533:bool)
            n437 = call <vilib>:"Clear Errors.vi"("error in (no error)"=w1527) -> ("error out"=w1523:errorcluster)  [unwired: 5 in, 1 out]
            n438 = Format Into String(format string="Home Complete=%s, Loop Counter=%d, Status=%x, Encoder=%d, Error Code=%d\n, MC SM State=%x, M_Ctrl=%x", w1530, w1524, w1528, w1525, w1521, w1520, w1519) -> (resulting string=w1518:string)  [unwired: 2 in, 1 out]
            n439 = case shown="False" w1533 {
              tunnel: [w1542 _] -> w1534
              tunnel: w1516 -> [w1540 _]
              frame False {
                n440 = call "Setup Delay for Next State.vi"("Period"=1000, "Next State"=w1540) -> ("error out"=w1542:errorcluster)  [unwired: 9 in]
              }
              frame True {
              }
            }
            n441 = Bundle By Name(cluster=w1532, "Loop Counter"=w1529) -> (w1538:T8)
            n442 = call "Log General Event Helper.vi"("Payload"=w1518, "State Info"=w1516, "EventLog in"=w1517) -> ("error out"=w1539:errorcluster)  [unwired: 7 in, 1 out]
            n443 = Merge Errors(w1539, w1534, w1523) -> (w1535:errorcluster)
          }
          frame "Update Cycle Count" {
            # "Update the cycle count locally and write the updated value to the cycle count.xml file in the tool."
            n444 = Unbundle By Name(w1558) -> ("Cycle Count"=w1556:i32, "EventLog.lvclass"=w1559:refnum<class "EventLog.lvclass">)
            n445 = Increment(x=w1556) -> (x+1=w1547:i32)
            n446 = Bundle By Name(cluster=T63 {"Cycle Count"=0} ("_Cycle Count File Cluster"), "Cycle Count"=w1547) -> (w1552:T63)
            n447 = Bundle By Name(cluster=w1558, "Cycle Count"=w1547) -> (w1557:T8)
            n448 = Flatten To XML(anything=w1552) -> (xml string=w1551:string)
            n449 = Build Array(w1551) -> (w1549:string[])
            n450 = call "Write to File.vi"("error in (no error)"=w1555, "Flattened data strings"=w1549, "Filename"="Cycle Count.xml") -> ("error out"=w1554:errorcluster)  [unwired: 8 in]
            n451 = Format Into String(format string="Cycle Count=%d", w1547) -> (resulting string=w1548:string)  [unwired: 2 in, 1 out]
            n452 = call "Log General Event Helper.vi"("Payload"=w1548, "State Info"=w1543, "EventLog in"=w1559) -> ("error out"=w1544:errorcluster)  [unwired: 7 in, 1 out]
            n453 = Merge Errors(w1554, w1544) -> (w1545:errorcluster)
          }
          frame "Start Monitor" {
            # "Start collecting data while moving from the start position back toward home. Set the Inspect Speed, probe data parameters such as array size and mode. Don't set STATUS.Inspecting true yet.  Wait for Inspect Range state does that."
            n454 = Variant To Data(type=FALSE, Variant=w1576) -> (data=w1568:bool, error out=w1574:errorcluster)  [unwired: 1 in]
            n455 = Unbundle By Name(w1573) -> ("EventLog.lvclass"=w1566:refnum<class "EventLog.lvclass">)
            n456 = call "Get Inspect Speed.vi"() -> ("Inspect Speed"=w1578:u16)  [unwired: 11 in]
            n457 = call "Motion Set Speed.vi"("Speed"=w1578) -> ("error out"=w1577:errorcluster)  [unwired: 10 in]
            n458 = call "CD_MGR Run.vi"("error in (no error)"=w1577, "Lasers ON?"=w1568) -> ("error out"=w1572:errorcluster, "Start Collect (Reply Payload)"=w1587:T73)  [unwired: 7 in, 1 out]
            n459 = Unbundle By Name(w1587) -> ("Success"=w1571:bool)
            n460 = Select(t="Monitor Sample Data" ("Message"), s=w1571, f="Stop Monitor") -> (s? t:f=w1581:string)
            n461 = call "Boolean to Text.vi"("selector"=w1571) -> ("output string"=w1570:string)  [unwired: 4 in]
            n462 = call "Boolean to Text.vi"("selector"=w1568) -> ("output string"=w1567:string)  [unwired: 4 in]
            n463 = call-poly <vilib>:"Delacor_lib_QMH_Enqueue Message (poly).vi"("error in (no error)"=w1574, "Message"=w1581, "Message Queue in"=w1585) -> ("error out"=w1562:errorcluster)  [unwired: 7 in, 1 out]
            n464 = Format Into String(format string="CD MGR Run=%s, Run Lasers=%s", w1570, w1567) -> (resulting string=w1565:string)  [unwired: 2 in, 1 out]
            n465 = call "Log General Event Helper.vi"("Payload"=w1565, "State Info"=w1564, "EventLog in"=w1566) -> ("error out"=w1560:errorcluster, "EventLog out"=w1563:refnum<class "EventLog.lvclass">)  [unwired: 7 in]
            n466 = call "Error Event.vi"("error in (no error)"=w1572, "EventLog ref"=w1563) -> ("error out"=w1561:errorcluster)  [unwired: 8 in, 1 out]
            n467 = Bundle By Name(cluster=w1573, "Trig State"=FALSE ("STATUS.Trigger"), "Cancel Inspect"=FALSE, "STATUS.Inspecting"=w1571) -> (w1580:T8)
            n468 = Merge Errors(w1562, w1561, w1560) -> (w1586:errorcluster)
          }
          frame "Monitor Sample Data" {
            # "#ToDo insert index.\n(Temporary insert 0\nhere)."
            # "Subtract the Start Sample No. from the current sample number and replace the value in the sample data array."
            # "Get the last data sample, replace the sample number with one reduced by the number of samples taken before the nspection actually started.  Send via the Sample Data notifier to the main app. Check if the inspection is done, either by exceeding max samples or at end of scan position."
            n469 = global read "ToolModGLOB.vi" "Data Stream Fmt Params"() -> (w1589:T70)
            n470 = Unbundle By Name(w1605) -> ("Cancel Inspect"=w1617:bool, "Host SampleData"=w1614:refnum<notifier>)
            n471 = call "Get Op Cfg.vi"() -> ("Tool Operation Config"=w1592:T72)  [unwired: 11 in]
            n472 = Unbundle By Name(w1605) -> ("STATUS.Status"=w1602:u16, "Trig State"=w1601:bool)
            n473 = call "IHL_HS Stream Sample Data Notifier.vi"() -> ("Sample Data notifier out"=w1596:refnum<notifier>)  [unwired: 10 in, 1 out]
            n474 = Unbundle By Name(w1592) -> ("Full Array Read Length"=w1591:i16)
            n475 = Unbundle By Name(w1589) -> ("Raw Data Status Len"=w1588:i32)
            n476 = Wait on Notification(notifier=w1596, timeout in ms (-1)=300) -> (notification=w1593:u32[], error out=w1594:errorcluster)  [unwired: 2 in, 2 out]
            n477 = case shown="True" w1617 {
              tunnel: [w1624 w1625] -> w1609
              tunnel: w1618 -> [w1623 w1626]
              tunnel: w1616 -> [w1622 w1627]
              tunnel: [TRUE _] -> w1611
              frame False {
                # "Inspection not Cancelled."
                n478 = call-poly <vilib>:"Delacor_lib_QMH_Enqueue Message (poly).vi"("error in (no error)"=w1622, "Message"="Monitor Sample Data", "Message Queue in"=w1623) -> ("error out"=w1624:errorcluster)  [unwired: 7 in, 1 out]
              }
              frame True {
                # "If Cancel Inspect is true, then go stop the inspection."
                n479 = call-poly <vilib>:"Delacor_lib_QMH_Enqueue Message (poly).vi"("error in (no error)"=w1627, "Message"="Stop Monitor", "Message Queue in"=w1626) -> ("error out"=w1625:errorcluster)  [unwired: 7 in, 1 out]
              }
            }
            n480 = call "Check Start Button.vi"("Trigger Status"=w1601, "Status Byte"=w1602) -> ("error out"=w1603:errorcluster, "Trigger Pressed?"=w1604:bool)  [unwired: 8 in]
            n481 = call "Parse CD Notifier Data V2.vi"("Status Hdr Length"=w1588, "Pixel Array Length"=w1591, "Sample Data Array"=w1593) -> ("Last Sample"=w1590:u32[])  [unwired: 4 in, 4 out]
            n482 = Replace Array Subset(array=w1590, new element=u32 0 ("new element/subarray")) -> (w1610:u32[])  [unwired: 1 in]
            n483 = Insert Into Array(array=w1610, index=5, new element=u32 0 ("new element/subarray")) -> (w1600:u32[])
            n484 = Bundle By Name(cluster=T71 {"Inspecting"=FALSE, "Acquiring Data"=FALSE, "Success"=FALSE, "Cancelled"=FALSE, "Scan Data Array"=[], "error cluster"={"status"=FALSE, "code"=0, "source"=""}} ("_Full Scan Data Rtn Cluster"), "Inspecting"=w1611, "Scan Data Array"=w1600) -> (w1612:T71)
            n485 = Send Notification(notification=w1612, notifier=w1614, error in (no error)=w1609) -> (error out=w1608:errorcluster)  [unwired: 1 out]
            n486 = Bundle By Name(cluster=w1605, "Trig State"=w1604) -> (w1615:T8)
            n487 = call <vilib>:"Clear Errors.vi"("error in (no error)"=w1608, "specific error code to clear (0: all)"=1) -> ("error out"=w1607:errorcluster)  [unwired: 4 in, 1 out]
            n488 = Merge Errors(w1603, w1594, w1607) -> (w1619:errorcluster)
          }
          frame "Stop Monitor" {
            # "#ToDo: Deal with errors"
            # "Stop Mode LED Blinking;\nPower off LaserOn LED"
            # "Stop the inspection.  If Inspecting is still true, then ok to get and save the data. If inspecting is false, then inspection cancelled and no data. Data is saved locally until the main app requests it."
            n489 = Unbundle By Name(w1630) -> ("STATUS.Inspecting"=w1632:bool)
            n490 = case shown="True" w1632 {
              tunnel: [_ w1642] -> w1631
              tunnel: [FALSE _] -> w1629
              frame False {
              }
              frame True {
                n491 = call "Stop Collect.vi"() -> ("error out"=w1641:errorcluster)  [unwired: 9 in, 2 out]
                n492 = call "Stop Module.vi"("Timeout to Wait for Stop (s) (-1: no timeout)"=5.0, "error in (no error)"=w1641, "Wait for Module to Stop? (F)"=TRUE) -> ("error out"=w1642:errorcluster)  [unwired: 8 in]
              }
            }
            n493 = call-poly <vilib>:"Delacor_lib_QMH_Enqueue Message (poly).vi"("error in (no error)"=w1639, "Message"="Ready", "Message Queue in"=w1636) -> ("error out"=w1638:errorcluster)  [unwired: 7 in, 1 out]
            n494 = Bundle By Name(cluster=w1630, "STATUS.Inspecting"=FALSE, "CD Success"=w1629) -> (w1634:T8)
            n495 = Merge Errors(w1631, w1638) -> (w1637:errorcluster)
          }
          frame "EXIT: Shutdown Tool" {
            # "Exit - Exit the application. \nQueue CONNECT, then EXIT: Update Status.  Using priority set true we enqueue in reverse order cause it enqueues to the front of the queue."
            n496 = Unbundle By Name(w1656) -> ("EventLog.lvclass"=w1651:refnum<class "EventLog.lvclass">)
            n497 = Build Array(variant ("Message Data"), T21 {"Connect"=FALSE} ("CONNECT Argument")) -> (w1645:variant[])
            n498 = call-poly <vilib>:"Delacor_lib_QMH_Enqueue Message (poly).vi"("Priority Message? Array"=bool[] [TRUE, TRUE] ("Priority Message? (F)"), "error in (no error)"=w1652, "Message Data Array"=w1645, "Message Array"=string[] ["EXIT: Update Status", "CONNECT"] ("Message"), "Message Queue in"=w1653) -> ("error out"=w1654:errorcluster)  [unwired: 5 in, 1 out]
            n499 = Bundle By Name(cluster=w1656, "OK to Connect"=FALSE) -> (w1658:T8)
            n500 = call "Log General Event Helper.vi"("State Info"=w1650, "EventLog in"=w1651) -> ("error out"=w1649:errorcluster)  [unwired: 8 in, 1 out]
            n501 = Merge Errors(w1654, w1649) -> (w1659:errorcluster)
          }
          frame "EXIT: Update Status" {
            n502 = Unbundle By Name(w1665) -> ("EventLog.lvclass"=w1663:refnum<class "EventLog.lvclass">, "STATUS"=w1660:T9)
            n503 = call "Send Status.vi"("error in (no error)"=w1669, "STATUS"=w1660) -> ("error out"=w1668:errorcluster)  [unwired: 9 in]
            n504 = call "Log General Event Helper.vi"("State Info"=w1661, "EventLog in"=w1663) -> ("error out"=w1662:errorcluster)  [unwired: 8 in, 1 out]
            n505 = call-poly <vilib>:"Delacor_lib_QMH_Enqueue Message (poly).vi"("Priority Message? (F)"=TRUE, "error in (no error)"=w1668, "Message"="EXIT: Shutdown Timers", "Message Queue in"=w1670) -> ("error out"=w1666:errorcluster)  [unwired: 6 in, 1 out]
            n506 = call <vilib>:"Clear Errors.vi"("error in (no error)"=w1662) -> ()  [unwired: 5 in, 2 out]
          }
          frame "EXIT: Shutdown Timers" {
            # "Exit - Exit the application."
            n507 = flat-sequence {
              tunnel: w1680 -> [w1686]
              tunnel: w1681 -> [w1687]
              tunnel: [w1687] -> w1679
              tunnel: [w1686] -> w1678
              tunnel: w1677 -> [w1684]
              tunnel: [w1684] -> w1676
              tunnel: w1675 -> [w1683]
              tunnel: [w1683] -> w1674
              tunnel: w1679 -> [w1701]
              tunnel: w1678 -> [w1700]
              tunnel: w1676 -> [w1699]
              tunnel: [w1696] -> w1671
              tunnel: w1674 -> [w1697]
              tunnel: [w1695] -> w1673
              tunnel: [w1693] -> w1672
              frame #0 {
                n508 = Wait (ms)(milliseconds to wait=u32 200) -> ()  [unwired: 1 out]
              }
              frame #1 {
                # "Close notifier reference for Raw Data Stream Receiver (Sample Data)."
                n509 = call "Obtain Host Sample Data Notifier.vi"() -> ("error out"=w1688:errorcluster, "Data Notifiers"=w1690:T74)  [unwired: 10 in]
                n510 = call "IHL_HS Stream Sample Data Notifier.vi"() -> ("error out"=w1692:errorcluster, "Sample Data notifier out"=w1691:refnum<notifier>)  [unwired: 10 in]
                n511 = Unbundle By Name(w1690) -> ("Sample Data"=w1689:refnum<notifier>)
                n512 = Unbundle By Name(w1699) -> ("EventLog.lvclass"=w1698:refnum<class "EventLog.lvclass">)
                n513 = Release Notifier(notifier=w1689, error in (no error)=w1688) -> ()  [unwired: 1 in, 3 out]
                n514 = Release Notifier(notifier=w1691, error in (no error)=w1692) -> ()  [unwired: 1 in, 3 out]
                n515 = call "Stop Helper Loops.vi"() -> ("error out"=w1694:errorcluster)  [unwired: 11 in]
                n516 = disable-structure shown="Enabled" {
                  disable-tunnel: [w1707 _] -> w1695
                  disable-tunnel: w1701 -> [w1705 _]
                  disable-tunnel: w1700 -> [w1704 _]
                  frame Enabled {
                    n517 = call-poly <vilib>:"Delacor_lib_QMH_Enqueue Message (poly).vi"("Priority Message? (F)"=TRUE, "error in (no error)"=w1704, "Message"="Exit", "Message Queue in"=w1705) -> ("error out"=w1707:errorcluster)  [unwired: 6 in, 1 out]
                  }
                  frame Disabled {
                  }
                }
                n518 = call "Log General Event Helper.vi"("State Info"=w1697, "EventLog in"=w1698) -> ("error out"=w1696:errorcluster)  [unwired: 8 in, 1 out]
                n519 = call "wait (ms) with error clusters.vi"("error in (no error)"=w1694, "milliseconds to wait"=u32 100) -> ("error out"=w1693:errorcluster)  [unwired: 9 in]
              }
            }
            n520 = Merge Errors(w1673, w1672, w1671) -> (w1682:errorcluster)
          }
          frame "-------Copy This Frame-------" {
            # "Duplicate this frame when creating new messages.  Change this comment in the duplicated frame to describe this message."
            n521 = Merge Errors(w1710) -> (w1708:errorcluster)
          }
          frame "------- Exit and Error Handling-------" {
            # "Separator - The following cases handle errors and exit messages."
            n522 = Merge Errors(w1713) -> (w1711:errorcluster)
          }
          frame "Simulate MHL Error" {
            # "Simulate an error occurring at the MHL"
            n523 = call "Module Name--constant.vi"() -> ("Module Name"=w1715:string)  [unwired: 11 in]
            n524 = xnode "Error Ring"("parameter 0"=w1715) -> ("error out"=w1714:errorcluster)
            n525 = Merge Errors(w1718, w1714) -> (w1716:errorcluster)
          }
          frame "Error" {
            # "#CodeRecommended - If you ever change the name of this \"Error\" message, you'll need to update the name in the Check Loop Error.vi as well."
            # "#CodeRecommended - If the module is running in standalone mode (External Launch = FALSE), this code will pop up an error dialog and call the 'Exit' message if an error occurs. Add more fine-grained error handling here."
            # "Error - Check the error message data and respond accordingly. This message is sent by the \"Error Handler\" VIs at the end of each loop in this application."
            n526 = property on="Property Node" class="Module Admin"(reference=w1730) -> ("Accessors:External Launch"=w1729:bool)  [unwired: 1 in, 2 out]
            n527 = Variant To Data(error in=w1737, type=errorcluster {"status"=FALSE, "code"=0, "source"=""} ("error constant"), Variant=w1735) -> (data=w1738:errorcluster, error out=w1733:errorcluster)
            n528 = call "Error Reported.vi"("Additional Information"=w1726, "Error"=w1738) -> ("error out"=w1727:errorcluster)  [unwired: 9 in]
            n529 = case shown="True" w1729 {
              tunnel: [w1743 _] -> w1732
              tunnel: w1731 -> [w1742 _]
              tunnel: w1738 -> [w1739 _]
              tunnel: w1727 -> [_ _]
              frame False {
                # "If the module is running standalone, then pop up an error dialog and call the \"Exit\" message."
                n530 = call <vilib>:"Simple Error Handler.vi"("error in (no error)"=w1739) -> ()  [unwired: 4 in, 5 out]
                n531 = call-poly <vilib>:"Delacor_lib_QMH_Enqueue Message (poly).vi"("Priority Message? (F)"=TRUE, "Message"="Exit", "Message Queue in"=w1742) -> ("error out"=w1743:errorcluster)  [unwired: 7 in, 1 out]
              }
              frame True {
                # "If the module was launched externally, calling the Error Reported broadcast VI is the only action performed by the \"Error\" message. The module's caller can then process the error appropriately."
              }
            }
            n532 = Merge Errors(w1733, w1732) -> (w1728:errorcluster)
            n533 = local write "error out"(w1728) -> ()
          }
          frame "Confirm Quit" {
            # "#CodeNeeded - If you want to provide an \"Are you sure\" dialog (or some other notification) before the application exits, place that code here. This message is typically sent from a Panel Close? event."
            # "Confirm Quit - Message that can confirm whether or not the user wants to exit the application."
            n534 = call-poly <vilib>:"Delacor_lib_QMH_Enqueue Message (poly).vi"("Priority Message? (F)"=TRUE, "error in (no error)"=w1750, "Message"="Exit", "Message Queue in"=w1746) -> ("error out"=w1747:errorcluster)  [unwired: 6 in, 1 out]
            n535 = Merge Errors(w1747) -> (w1748:errorcluster)
          }
          frame "Exit" {
            w1764 = 91  # 91: not all Exit messages will have an argument
            w1768 = TRUE  # Stop the VI
            # "Release the message queue reference"
            # "Exit - Exit the application."
            n536 = Release Notifier(notifier=w1772) -> (error out=w1752:errorcluster)  [unwired: 2 in, 2 out]
            n537 = Variant To Data(error in=w1770, type=T20 {"Origin"="", "Exit via Stop Module Req?"=FALSE, "Wait for Module to stop?"=FALSE} ("Stop Argument"), Variant=w1766) -> (data=w1762:T20, error out=w1765:errorcluster)
            n538 = call <vilib>:"Clear Errors.vi"("error in (no error)"=w1752) -> ()  [unwired: 5 in, 2 out]
            n539 = disable-structure shown="Disabled" {
              disable-tunnel: [w1775 _] -> w1751
              frame Disabled {
                # "This is handled in IHL."
                n540 = call "Obtain Raw HS Stream Ctrl Notifiers.vi"() -> ("error out"=w1776:errorcluster, "Loop Ctrl Notifiers Cluster"=w1778:T13)  [unwired: 10 in]
                n541 = Unbundle By Name(w1778) -> ("Raw Stream Ctrl"=w1777:refnum<notifier>)
                n542 = Release Notifier(notifier=w1777, error in (no error)=w1776) -> (error out=w1775:errorcluster)  [unwired: 1 in, 2 out]
              }
              frame Enabled {
              }
            }
            n543 = call <vilib>:"Clear Errors.vi"("error in (no error)"=w1765, "specific error code to clear (0: all)"=w1764) -> ("error out"=w1769:errorcluster)  [unwired: 4 in, 1 out]
            n544 = Unbundle By Name(w1759) -> ("EventLog.lvclass"=w1757:refnum<class "EventLog.lvclass">, "Host SampleData"=w1758:refnum<notifier>)
            n545 = control-ref of="This VI"() -> (w1761:refnum<vi>)
            n546 = call-dynamic "Delacor_lib_QMH_Release Message Queue.vi"("error in (no error)"=w1769, "Message Queue"=w1771) -> ("error out"=w1755:errorcluster)  [unwired: 9 in]
            n547 = call "Log General Event Helper.vi"("State Info"=w1756, "EventLog in"=w1757) -> ("error out"=w1753:errorcluster)  [unwired: 8 in, 1 out]
            n548 = call "Handle Exit.vi"("Stop Argument"=w1762, "Admin in"=w1760, "VI reference"=w1761) -> ("error out"=w1754:errorcluster)  [unwired: 7 in, 1 out]
            n549 = disable-structure shown="Disabled" {
              disable-tunnel: w1758 -> [w1774 _]
              frame Disabled {
                # "This is closed when inspecting stopped."
                n550 = Release Notifier(notifier=w1774) -> (error out=w1773:errorcluster)  [unwired: 2 in, 2 out]
                n551 = call <vilib>:"Clear Errors.vi"("error in (no error)"=w1773) -> ()  [unwired: 5 in, 2 out]
              }
              frame Enabled {
              }
            }
            n552 = call <vilib>:"Clear Errors.vi"("error in (no error)"=w1753) -> ()  [unwired: 5 in, 2 out]
            n553 = Merge Errors(w1755, w1754, w1751) -> (w1767:errorcluster)
          }
          frame Default {
            # "'Default' case only runs if there is a message that isn't defined in any of the other cases.  Output a programming error."
            n554 = call "Module Name--constant.vi"() -> ("Module Name"=w1779:string)  [unwired: 11 in]
            n555 = xnode "Error Ring"("parameter 0"=w1780, "parameter 1"=w1779) -> ("error out"=w1781:errorcluster)
          }
          frame "Do Nothing State" {
          }
          frame "------- Depricated -------" {
          }
          frame "------- New Cmds -------" {
          }
        }
        n556 = call-dynamic "Delacor_lib_QMH_Error Handler - Message Handling Loop.vi"("error in (no error)"=w530, "Message Queue in"=w522) -> ("dup error in"=w521:errorcluster)  [unwired: 8 in, 1 out]
      }
      n557 = while {
        tunnel: w69 -> [w106]
        shift-right: [w105] -> _
        shift-left: w68 -> [w98]
        tunnel: w64 -> [w101]
        tunnel: w66 -> [w97]
        tunnel: [w100] -> w67
        tunnel: [w99] -> w62
        stop <- w103 stop-if-true
        # "Inspecting Helper Loop (IHL)"
        n558 = Unbundle By Name(w98) -> ("Timeout"=w104:i32)
        n559 = event shown="[2] <Start Inspect 2>: User Event" {
          selector: w106 -> [_ _ _ _ _ _]
          dyn-events: [_ _ _ _ _ _] -> w100
          timeout: w104 -> [_ _ _ _ _ _]
          tunnel: w98 -> [w108 w233 w248 w273 w281 w283]
          tunnel: [w113 w232 w247 w273 w280 w283] -> w105
          tunnel: [_ _ _ _ _ TRUE] -> w103
          tunnel: [w112 _ w244 w278 _ w282] -> w102
          tunnel: w101 -> [w111 _ _ _ _ _]
          tunnel: w97 -> [w109 _ _ _ _ _]
          event Timeout {
            n560 = event-data() -> ()  [unwired: 1 in, 1 out]
            n561 = Unbundle By Name(w108) -> ("IHL State"=w114:T3, "EventLog"=w110:refnum<class "EventLog.lvclass">)
            n562 = call "IHL_Update Loop Data.vi"("Inspect Helper Loop Data"=w108, "Tool Status notifier"=w109) -> ("Inspect Helper Loop Data out"=w107:T2)  [unwired: 8 in, 1 out]
            n563 = case shown="\"Inspect: START\"" w114 {
              tunnel: [w116 w138 w147 w173 w175 w186 w210 w212 w216 w222] -> w113
              tunnel: w107 -> [w124 w128 w155 w170 w174 w195 w211 w213 w217 w225]
              tunnel: [w118 w131 w150 w172 w176 w180 w209 w215 w218 w223] -> w112
              tunnel: w111 -> [_ _ w159 _ w177 w184 _ w214 _ w226]
              tunnel: w110 -> [_ w127 w145 w163 _ w196 w200 _ _ _]
              frame "Init", Default {
                # "Once we do one cycle of \"Init\" state, set Timeout to -1 (no timeout)."
                # "Make sure the HS Raw Data receiver loop is in idle mode. We set the other parameters in the Inspect:START state."
                n564 = Bundle By Name(cluster=T16 {"Raw Data Stream Loop cmd"=enum."Idle", "Data Array DVR ref"=refnum, "HS Sample Data notifier"=refnum, "Block Count Notifier"=refnum} ("_HS Data Stream Params Cluster--typedef"), "Raw Data Stream Loop cmd"=_HS_Data_Stream_SM_enum--typedef."Idle") -> (w120:T16)
                n565 = call "Obtain Raw HS Stream Ctrl Notifiers.vi"() -> ("error out"=w119:errorcluster, "Loop Ctrl Notifiers Cluster"=w121:T13)  [unwired: 10 in]
                n566 = Bundle By Name(cluster=w124, "Timeout"=-1) -> (w116:T2)
                n567 = Unbundle By Name(w121) -> ("Raw Stream Ctrl"=w122:refnum<notifier>)
                n568 = Send Notification(notification=w120, notifier=w122, error in (no error)=w119) -> (error out=w118:errorcluster)  [unwired: 1 out]
              }
              frame "Set Motion Speed" {
                # "Set to 100 to allow time for host to observe the False Inspecting flag. In next state, we set it to True."
                n569 = call "Get Jog Speed.vi"() -> ("Jog Speed"=w133:u16)  [unwired: 11 in]
                n570 = call "Motion Set Speed.vi"("Speed"=w133) -> ("error out"=w130:errorcluster)  [unwired: 10 in]
                n571 = Format Into String(format string="Set Speed to %d", w133) -> (resulting string=w135:string)  [unwired: 2 in, 1 out]
                n572 = Bundle By Name(cluster=w128, "IHL State"=_IHL_SM_Enum--typedef."Move To Scan Start" ("Inspect State"), "Timeout"=100, "Success Flag"=FALSE, "Inspect Status"=T4 {"Ready"=FALSE, "Inspecting"=FALSE, "Cancel"=FALSE}) -> (w138:T2)
                n573 = call "Log General Event Helper.vi"("Payload"=w135, "State Info"="IHL:Timeout: Set Motion Speed", "EventLog in"=w127) -> ("error out"=w129:errorcluster)  [unwired: 7 in, 1 out]
                n574 = Merge Errors(w130, w129) -> (w131:errorcluster)
              }
              frame "Move To Scan Start" {
                w141 = TRUE  # Inspecting
                w143 = FALSE  # Decel?
                # "Now we turn on the Inspecting flag (for host)."
                n575 = Unbundle By Name(w155) -> ("PosToStartScan"=w152:i32)
                n576 = call "Get Start Delay.vi"() -> ("Encoder out"=w157:i32)  [unwired: 10 in, 1 out]
                n577 = Add(x=w152, y=w157) -> (x+y=w144:i32)
                n578 = Format Into String(format string="InspectLim.PosToStart=%d, Final Start Pos=%d", w152, w144) -> (resulting string=w154:string)  [unwired: 2 in, 1 out]
                n579 = call "Motion Move Absolute.vi"("Decel?"=w143, "Position"=w144) -> ("error out"=w140:errorcluster)  [unwired: 9 in]
                n580 = Bundle By Name(cluster=w155, "IHL State"=_IHL_SM_Enum--typedef."Wait for Motion Out" ("Inspect State"), "Timeout"=100) -> (w147:T2)
                n581 = call "Update Host Sample Data.vi"("Inspecting"=w141, "error in (no error)"=w140) -> ("error out"=w139:errorcluster)  [unwired: 9 in]
                n582 = Unbundle By Name(w147) -> ("Inspect Status"=w146:T4)
                n583 = call-poly <vilib>:"Delacor_lib_QMH_Enqueue Message (poly).vi"("Message Data"=w146, "Message"="Update Inspect Status", "Message Queue in"=w159) -> ("error out"=w149:errorcluster)  [unwired: 7 in, 1 out]
                n584 = call "Log General Event Helper.vi"("Payload"=w154, "State Info"="IHL: Timeout: Move to Scan Start", "EventLog in"=w145) -> ("error out"=w142:errorcluster)  [unwired: 7 in, 1 out]
                n585 = Merge Errors(w139, w149, w142) -> (w150:errorcluster)
              }
              frame "Wait for Motion Out" {
                w166 = _IHL_SM_Enum--typedef."Wait for Start Pos"  # New State on success
                n586 = Unbundle By Name(w170) -> ("Status"=w161:u16, "Inspect Status.Cancel"=w160:bool, "IHL State"=w168:T3, "Loop Count"=w167:i32)  [unwired: 1 out]
                n587 = call "IHL_Wait for Motion Helper.vi"("Status"=w161, "EventLog ref"=w163, "Cancel"=w160, "Loop Count in"=w167, "Next State"=w166, "Current State"=w168) -> ("error out"=w165:errorcluster, "Loop Count out"=w162:i32, "New State out"=w169:T3)  [unwired: 3 in]
                n588 = Bundle By Name(cluster=w170, "IHL State"=w169, "Loop Count"=w162) -> (w173:T2)
                n589 = call "Log Wait Motion Helper.vi"("Cancel"=w160, "State Info"="IHL:Timeout: Wait for Motion Out", "Status"=w161, "Loop Count"=w162, "EventLog in"=w163) -> ("error out"=w164:errorcluster)  [unwired: 5 in, 1 out]
                n590 = Merge Errors(w165, w164) -> (w172:errorcluster)
              }
              frame "Wait for Start Pos" {
                # "Wait for the Start position. When we reach it, wait 500mSec before starting the inspection to allow motor/stage to settle."
                n591 = call "IHL_Wait for Start Pos Helper.vi"("Inspect Helper Loop Data"=w174, "Message Queue in"=w177) -> ("error out"=w176:errorcluster, "Inspect Helper Loop Data out"=w175:T2)  [unwired: 8 in]
              }
              frame "Inspect: START" {
                (unwired) FALSE ("Success")
                # "Set to same rate as Tool Status gets updated."
                n592 = Unbundle By Name(w195) -> ("Encoder Count"=w181:i32, "PosToEndScan"=w194:i32, "MaxSamples"=w193:i32)
                n593 = call "IHL_Inspect-Start Helper.vi"("Encoder Cnt"=w181, "MaxSamples"=w193, "PosToEndScan"=w194, "EventLog in"=w196) -> ("error out"=w179:errorcluster, "Success"=w178:bool, "data value reference"=w190:refnum<data-value>, "Block Cnt notifier out"=w189:refnum<notifier>)  [unwired: 4 in]
                n594 = Select(t=_IHL_SM_Enum--typedef."Wait for Motion IN" ("Inspect State"), s=w178, f=_IHL_SM_Enum--typedef."Inspect: STOP") -> (s? t:f=w197:T3)
                n595 = Bundle By Name(cluster=w195, "Timeout"=50, "Loop Count"=0, "Collecting Data"=w178, "IHL State"=w197, "Block Cnt notifier out"=w189, "data value reference"=w190) -> (w186:T2)
                n596 = Unbundle By Name(w186) -> ("Inspect Status"=w185:T4)
                n597 = call-poly <vilib>:"Delacor_lib_QMH_Enqueue Message (poly).vi"("Message Data"=w185, "Message"="Update Inspect Status", "Message Queue in"=w184) -> ("error out"=w188:errorcluster)  [unwired: 7 in, 1 out]
                n598 = Merge Errors(w179, w188) -> (w180:errorcluster)
              }
              frame "Wait for Motion IN" {
                w205 = _IHL_SM_Enum--typedef."Wait for Inspect Range"  # New state on success
                n599 = Unbundle By Name(w211) -> ("Status"=w199:u16, "Inspect Status.Cancel"=w198:bool, "IHL State"=w201:T3, "Loop Count"=w202:i32)  [unwired: 1 out]
                n600 = call "IHL_Wait for Motion Helper.vi"("Status"=w199, "EventLog ref"=w200, "Cancel"=w198, "Loop Count in"=w202, "Next State"=w205, "Current State"=w201) -> ("error out"=w206:errorcluster, "Loop Count out"=w203:i32, "New State out"=w204:T3)  [unwired: 3 in]
                n601 = Bundle By Name(cluster=w211, "IHL State"=w204, "Loop Count"=w203) -> (w210:T2)
                n602 = call "Log Wait Motion Helper.vi"("Cancel"=w198, "State Info"="IHL:Timeout: Wait for Motion IN", "Status"=w199, "Loop Count"=w203, "EventLog in"=w200) -> ("error out"=w208:errorcluster)  [unwired: 5 in, 1 out]
                n603 = Merge Errors(w206, w208) -> (w209:errorcluster)
              }
              frame "Wait for Inspect Range" {
                # "When in Scan Range, Set time for 500mSec and wait before go to Inspecting."
                n604 = call "IHL_Wait for Inspect Range Helper.vi"("Inspect Helper Loop Data"=w213, "Message Queue in"=w214) -> ("error out"=w215:errorcluster, "Inspect Helper Loop Data out"=w212:T2)  [unwired: 8 in]
              }
              frame "Inspecting" {
                # "If Cancel==True \n   Then Set Inspecting Flag (in Scan return notifier) to False.\n   Else True \n\nSet Success Flag True if not Cancelled and Inspection complete\n   Else Set False if Cancel==True"
                n605 = call "IHL_Inspecting Helper.vi"("Inspect Helper Loop Data"=w217) -> ("error out"=w218:errorcluster, "Inspect Helper Loop Data out"=w216:T2)  [unwired: 8 in, 1 out]
              }
              frame "Inspect: STOP" {
                # "If inspecting and complete, Set Success Flag to True\n   Else Success Flag = False."
                n606 = call "IHL_Inspect-Stop Helper.vi"("Inspect Helper Loop Data"=w225, "Message Queue in"=w226) -> ("error out"=w223:errorcluster, "Inspect Helper Loop Data out"=w224:T2)  [unwired: 7 in, 1 out]
                n607 = Bundle By Name(cluster=w224, "IHL State"=_IHL_SM_Enum--typedef."Init" ("Inspect State"), "Timeout"=10, "Collecting Data"=FALSE) -> (w222:T2)
              }
            }
          }
          event User Event {
            n608 = event-data() -> ("Inspection Limits"=w231:T11)  [unwired: 1 in]
            n609 = Unbundle By Name(w231) -> ("PosToStartScan"=w230:i32, "ScanLength"=w229:i32, "MaxSamples"=w228:i32, "PosToEndScan"=w227:i32)
            n610 = Bundle By Name(cluster=w233, "PosToStartScan"=w230, "ScanLength"=w229, "MaxSamples"=w228, "PosToEndScan"=w227) -> (w232:T2)
          }
          event User Event {
            w240 = TRUE
            n611 = event-data() -> ("Start(T)/Stop(F)"=w242:bool, "Wait Notifier"=w246:refnum<notifier>, "wait for reply"=w237:bool)  [unwired: 1 in]
            n612 = Unbundle By Name(w248) -> ("EventLog"=w245:refnum<class "EventLog.lvclass">)  [unwired: 1 out]
            n613 = call "Obtain Host Sample Data Notifier.vi"() -> ("Data Notifiers"=w239:T74)  [unwired: 10 in, 1 out]
            n614 = Unbundle By Name(w239) -> ("Sample Data"=w238:refnum<notifier>)
            n615 = Not(x=w242) -> (.not. x?=w241:bool)
            n616 = And(x=w240, y=w242) -> (x .and. y?=w249:bool)
            n617 = call "Log Inspect State Helper.vi"("State Info"="IHL: <Start Inspect>: User Event", "Inspect"=w242, "Ready"=w240, "EventLog in"=w245) -> ("error out"=w243:errorcluster)  [unwired: 6 in, 1 out]
            n618 = case shown="False" w249 {
              tunnel: w248 -> [w253 w265]
              tunnel: [w252 w264] -> w247
              tunnel: w246 -> [_ w260]
              tunnel: w241 -> [w251 w261]
              tunnel: w238 -> [_ w257]
              tunnel: w237 -> [_ w256]
              tunnel: [_ w255] -> w236
              tunnel: [_ w254] -> w235
              frame False {
                n619 = Bundle By Name(cluster=w253, "Timeout"=1, "Inspect Status.Cancel"=w251) -> (w252:T2)
              }
              frame True {
                # "Set default values in the notifier."
                n620 = Bundle By Name(cluster=T17 {"Sample Data notifier"=refnum, "Start Inspect 2_error"={"status"=FALSE, "code"=0, "source"=""}} ("Start Inspect 2 (Reply Payload)"), "Sample Data notifier"=w257) -> (w258:T17)
                n621 = case shown="True" w256 {
                  tunnel: w260 -> [_ w268]
                  tunnel: w258 -> [_ w267]
                  tunnel: [_ w266] -> w255
                  frame False {
                  }
                  frame True {
                    n622 = Send Notification(notification=w267, notifier=w268) -> (error out=w266:errorcluster)  [unwired: 1 in, 1 out]
                  }
                }
                n623 = Bundle By Name(cluster=w265, "Timeout"=50, "IHL State"=_IHL_SM_Enum--typedef."Set Motion Speed" ("Inspect State"), "Inspect Status.Cancel"=w261) -> (w264:T2)
                n624 = call "Update Host Sample Data.vi"() -> ("error out"=w254:errorcluster)  [unwired: 11 in]
              }
            }
            n625 = Merge Errors(w235, w236, w243) -> (w244:errorcluster)
          }
          event User Event {
            n626 = event-data() -> ("Wait Notifier"=w277:refnum<notifier>)  [unwired: 1 in]
            n627 = Unbundle By Name(w273) -> ("Success Flag"=w272:bool, "data value reference"=w271:refnum<data-value>, "No. Samples"=w269:i32, "PosToStartScan"=w270:i32)
            n628 = call "Reverse Data Set V2.vi"("Pos to Start Scan"=w270, "data value reference"=w271, "Final No of Blocks"=w269) -> ("data value ref out"=w275:refnum<data-value>)  [unwired: 8 in]
            n629 = Bundle By Name(cluster=T18 {"Success"=FALSE, "Full Inspection Data"=[], "data value reference"=refnum} ("Get All Inspect Data (Reply Payload)"), "Success"=w272, "data value reference"=w275) -> (w274:T18)
            n630 = Send Notification(notification=w274, notifier=w277) -> (error out=w278:errorcluster)  [unwired: 1 in, 1 out]
          }
          event User Event {
            n631 = event-data() -> ("EventLog.lvclass"=w279:refnum<class "EventLog.lvclass">)  [unwired: 1 in]
            n632 = Bundle By Name(cluster=w281, "EventLog"=w279) -> (w280:T2)
          }
          event User Event {
            n633 = event-data() -> ()  [unwired: 1 in, 5 out]
            n634 = Unbundle By Name(w283) -> ()  [unwired: 1 out]
            n635 = call "Obtain Raw HS Stream Ctrl Notifiers.vi"() -> ("error out"=w285:errorcluster, "Loop Ctrl Notifiers Cluster"=w287:T13)  [unwired: 10 in]
            n636 = Unbundle By Name(w287) -> ("Raw Stream Ctrl"=w286:refnum<notifier>)
            n637 = Release Notifier(notifier=w286, error in (no error)=w285) -> (error out=w284:errorcluster)  [unwired: 1 in, 2 out]
            n638 = Merge Errors(w284) -> (w282:errorcluster)
          }
        }
        n639 = call-dynamic "Delacor_lib_QMH_Error Handler - Message Handling Loop.vi"("error in (no error)"=w102, "Message Queue in"=w101) -> ("dup error in"=w99:errorcluster)  [unwired: 8 in, 1 out]
      }
      n640 = while {
        tunnel: w64 -> [w1812]
        tunnel: w85 -> [w1814]
        shift-right: [w1810] -> _
        shift-left: w84 -> [w1811]
        shift-right: [w1803] -> _
        shift-left: w96 -> [w1809]
        tunnel: w83 -> [w1808]
        shift-right: [w1806] -> _
        shift-left: w82 -> [w1807]
        shift-right: [w1804] -> _
        shift-left: w74 -> [w1805]
        shift-right: [w1801] -> _
        shift-left: w95 -> [w1802]
        tunnel: [w1800] -> w81
        tunnel: [w1799] -> w80
        tunnel: w66 -> [w1797]
        stop <- w1813 stop-if-true
        # "Tool Status Reader State Machine Helper Loop"
        n641 = event shown="[2] <Time Expired>: User Event" {
          selector: w1814 -> [_ _ _ _]
          dyn-events: [_ _ _ _] -> w1799
          timeout: w1805 -> [_ _ _ _]
          tunnel: [_ _ _ TRUE] -> w1813
          tunnel: w1812 -> [_ _ w1907 _]
          tunnel: w1811 -> [w1824 w1903 w1908 w1931]
          tunnel: [w1823 w1903 w1908 w1931] -> w1810
          tunnel: w1809 -> [w1822 _ w1910 w1930]
          tunnel: w1808 -> [w1821 _ _ _]
          tunnel: w1807 -> [w1825 w1901 w1909 w1927]
          tunnel: [w1820 w1901 w1909 w1927] -> w1806
          tunnel: w1805 -> [w1819 w1900 w1905 w1929]
          tunnel: [w1818 w1900 w1905 w1929] -> w1804
          tunnel: [w1817 w1902 w1910 w1930] -> w1803
          tunnel: w1802 -> [w1816 w1904 w1911 w1928]
          tunnel: [w1815 w1904 w1911 w1928] -> w1801
          tunnel: [_ _ w1912 _] -> w1798
          tunnel: w1797 -> [_ _ w1906 _]
          event Timeout {
            n642 = event-data() -> ()  [unwired: 1 in, 1 out]
            n643 = case shown="\"Receive Data\"" w1824 {
              selector: w1824 -> [w1839 _ w1869 w1887 _]
              tunnel: w1821 -> [_ _ _ w1878 _]
              tunnel: [w1836 w1841 w1867 w1889 refnum<k21> refnum ("reader endpoint")] -> w1820
              tunnel: w1822 -> [w1827 w1843 w1858 w1874 w1893]
              tunnel: [w1838 w1848 w1866 w1885 _Motion_Status_Reader_SM_enum--typedef."Not Connected" ("_Motion Status Reader SM Enum--typedef")] -> w1823
              tunnel: [_ w1842 _ w1871 w1897] -> _
              tunnel: w1825 -> [w1836 _ w1867 w1879 w1899]
              tunnel: w1819 -> [_ w1844 _ _ _]
              tunnel: [w1831 w1844 10 1 ("milliseconds to wait") 10 ("milliseconds to wait")] -> w1818
              tunnel: [w1827 w1843 w1858 w1874 w1893] -> w1817
              tunnel: w1816 -> [w1826 w1840 w1857 w1873 w1892]
              tunnel: [w1826 w1840 w1857 w1872 w1892] -> w1815
              frame "Not Connected", Default {
                n644 = Equal?(x=_Host_-_HS_Data_Stream_State_Enum_Typedef."Connect", y=w1827) -> (x = y?=w1834:bool)
                n645 = Equal?(x=_Host_-_HS_Data_Stream_State_Enum_Typedef."Receive Data", y=w1827) -> (x = y?=w1832:bool)
                n646 = Or(x=w1834, y=w1832) -> (x .or. y?=w1828:bool)
                n647 = Select(t=1, s=w1828, f=10 ("milliseconds to wait")) -> (s? t:f=w1831:i32)
                n648 = Select(t=_Motion_Status_Reader_SM_enum--typedef."Connect", s=w1828, f=w1839) -> (s? t:f=w1838:T6)
              }
              frame "Connect" {
                n649 = global read "GLOB - Configuration Options.vi" "Controller Address"() -> (w1856:string)
                n650 = global read "GLOB - Configuration Options.vi" "Network Stream Connect Timeout (ms)"() -> (w1853:i32)
                n651 = Format Into String(format string="//%s/%s", w1856, "RT/MotionData/Writer" ("input 2")) -> (resulting string=w1852:string)  [unwired: 2 in, 1 out]
                n652 = Create Network Stream Reader Endpoint(5:w1853, 7:4096 ("reader buffer size"), 9:T5 {"Encoder"=0, "STATUS"=0, "MC SM State"=0, "M_Ctrl"=0} ("_Motion Status Cluster--typedef"), 10:w1852, 11:"Host/MotionData/Reader" ("reader name")) -> (0:w1842:errorcluster, 3:w1841:refnum<k21>)  [unwired: 2 in]
                n653 = Unbundle By Name(w1842) -> ("status"=w1847:bool)
                n654 = Select(t=_Motion_Status_Reader_SM_enum--typedef."Not Connected", s=w1847, f=_Motion_Status_Reader_SM_enum--typedef."Idle") -> (s? t:f=w1848:T6)
              }
              frame "Idle" {
                n655 = Equal?(x=w1858, y=_Host_-_HS_Data_Stream_State_Enum_Typedef."Receive Data" ("x")) -> (x = y?=w1870:bool)
                n656 = Equal?(x=w1858, y=_Host_-_HS_Data_Stream_State_Enum_Typedef."Close Connection" ("x")) -> (x = y?=w1863:bool)
                n657 = Select(t=_Motion_Status_Reader_SM_enum--typedef."Receive Data", s=w1870, f=w1869) -> (s? t:f=w1865:T6)
                n658 = global write "ToolModGLOB.vi" "Connected?"(TRUE ("Connected?")) -> ()
                n659 = Select(t=_Motion_Status_Reader_SM_enum--typedef."Disconnect", s=w1863, f=w1865) -> (s? t:f=w1866:T6)
              }
              frame "Receive Data" {
                n660 = shared-variable-read(w1879, w1878) -> (w1889:refnum<k21>, w1871:errorcluster, w1876:bool, w1877:T5)  [unwired: 1 in]
                n661 = case shown="False" w1876 {
                  tunnel: w1877 -> [w1890 _]
                  tunnel: w1873 -> [_ w1891]
                  tunnel: [w1890 w1891] -> w1872
                  frame False {
                  }
                  frame True {
                  }
                }
                n662 = Equal?(x=w1874, y=_Host_-_HS_Data_Stream_State_Enum_Typedef."Idle" ("x")) -> (x = y?=w1884:bool)
                n663 = Equal?(x=w1874, y=_Host_-_HS_Data_Stream_State_Enum_Typedef."Close Connection") -> (x = y?=w1882:bool)
                n664 = Select(t=_Motion_Status_Reader_SM_enum--typedef."Idle", s=w1884, f=w1887) -> (s? t:f=w1881:T6)
                n665 = Select(t=_Motion_Status_Reader_SM_enum--typedef."Disconnect", s=w1882, f=w1881) -> (s? t:f=w1885:T6)
              }
              frame "Disconnect" {
                n666 = global write "ToolModGLOB.vi" "Connected?"(FALSE ("Connected?")) -> ()
                n667 = Destroy Stream Endpoint(11:w1899) -> (0:w1897:errorcluster)  [unwired: 1 in]
              }
            }
          }
          event User Event {
            n668 = event-data() -> ("Command"=w1902:T7)  [unwired: 1 in]
          }
          event User Event {
            n669 = event-data() -> ("ID"=w1913:i32)  [unwired: 1 in]
            n670 = case shown="1" w1913 {
              tunnel: w1907 -> [_ w1926]
              tunnel: [_ w1915] -> w1912
              tunnel: w1911 -> [_ w1919]
              tunnel: w1908 -> [_ w1923]
              tunnel: w1906 -> [_ w1920]
              tunnel: w1905 -> [_ _]
              frame 0, Default {
                # "Any other timer ID is to be ignored."
              }
              frame 1 {
                # "Timer ID \"1\" is the one that drives this 50mSec update."
                n671 = Bundle("Tool Status Cluster"=w1919, "Tool Status Reader State"=w1923) -> (w1922:T75)  [unwired: 1 in]
                n672 = Unbundle By Name(w1919) -> ("STATUS"=w1918:u16, "Encoder"=w1917:i32)
                n673 = Bundle("STATUS"=w1918, "Encoder"=w1917) -> (w1916:cluster{"STATUS":u16, "Encoder":i32})  [unwired: 1 in]
                n674 = call-poly <vilib>:"Delacor_lib_QMH_Enqueue Message (poly).vi"("Priority Message? (F)"=TRUE, "Message Data"=w1922, "Message"="Tool Status Updated", "Message Queue in"=w1926) -> ("error out"=w1925:errorcluster)  [unwired: 6 in, 1 out]
                n675 = Send Notification(notification=w1916, notifier=w1920) -> (error out=w1914:errorcluster)  [unwired: 1 in, 1 out]
                n676 = Merge Errors(w1914, w1925) -> (w1915:errorcluster)
              }
            }
          }
          event User Event {
            n677 = event-data() -> ()  [unwired: 1 in, 1 out]
          }
        }
        n678 = call-dynamic "Delacor_lib_QMH_Error Handler - Message Handling Loop.vi"("error in (no error)"=w1798, "Message Queue in"=w1812) -> ("dup error in"=w1800:errorcluster)  [unwired: 8 in, 1 out]
      }
      n679 = while {
        tunnel: w64 -> [w291]
        tunnel: w73 -> [w296]
        shift-right: [w294] -> _
        shift-left: FALSE -> [w293]
        tunnel: [w290] -> w71
        tunnel: [w289] -> w70
        stop <- w295 stop-if-true
        # "RT Receive Stream Loop"
        n680 = event shown="[0] Timeout" {
          selector: w296 -> [_ _ _]
          dyn-events: [_ _ _] -> w289
          timeout: 1 -> [_ _ _]
          tunnel: w291 -> [w300 _ _]
          tunnel: [_ _ TRUE] -> w295
          tunnel: [w299 w316 w317] -> w294
          tunnel: w293 -> [w299 _ w317]
          tunnel: [w298 _ _] -> w292
          event Timeout {
            n681 = event-data() -> ()  [unwired: 1 in, 1 out]
            n682 = case shown="True" w299 {
              tunnel: w300 -> [_ w307]
              tunnel: [_ w302] -> w298
              frame False {
                n683 = Wait (ms)(milliseconds to wait=u32 25) -> ()  [unwired: 1 out]
              }
              frame True {
                n684 = call "Read Message from Tool.vi"() -> ("error out"=w303:errorcluster, "timed out?"=w309:bool, "Message Data"=w306:variant, "Message"=w305:string)  [unwired: 8 in]
                n685 = Or(x=w309, y=w303) -> (x .or. y?=w308:bool)
                n686 = case shown="False" w308 {
                  tunnel: w307 -> [w314 w315]
                  tunnel: w306 -> [w313 _]
                  tunnel: w305 -> [w312 _]
                  tunnel: [w311 w315] -> w304
                  tunnel: [w310 _] -> _
                  frame False {
                    n687 = call-poly <vilib>:"Delacor_lib_QMH_Enqueue Message (poly).vi"("Message Data"=w313, "Message"=w312, "Message Queue in"=w314) -> ("error out"=w310:errorcluster, "Message Queue out"=w311:refnum<class "Delacor_lib_QMH_Message Queue.lvclass">)  [unwired: 7 in]
                  }
                  frame True {
                  }
                }
                n688 = call-dynamic "Delacor_lib_QMH_Error Handler - Event Handling Loop.vi"("error in (no error)"=w303, "Message Queue in"=w304) -> ("dup error in"=w302:errorcluster)  [unwired: 8 in, 1 out]
              }
            }
          }
          event User Event {
            n689 = event-data() -> ("Enable"=w316:bool)  [unwired: 1 in]
          }
          event User Event {
            n690 = event-data() -> ()  [unwired: 1 in, 1 out]
          }
        }
        n691 = call-dynamic "Delacor_lib_QMH_Error Handler - Message Handling Loop.vi"("error in (no error)"=w292, "Message Queue in"=w291) -> ("dup error in"=w290:errorcluster)  [unwired: 8 in, 1 out]
      }
      n692 = call "Raw Data Stream Receiver.vi"("error in (no error)"=w65, "Raw Stream Ctrl"=w63) -> ()  [unwired: 9 in, 1 out]
      n693 = disable-structure shown="Disabled" {
        disable-tunnel: w64 -> [w320 _]
        disable-tunnel: w87 -> [w319 _]
        frame Disabled {
          n694 = call "Read Stream from RT.vi"("Connected notifier"=w319, "Message Queue in"=w320) -> ()  [unwired: 9 in, 1 out]
        }
        frame Enabled {
        }
      }
      n695 = call "Timer Helper Loop.vi"("Timer ID"=w79, "Setup Timer"=w76, "Stop Helper Loop"=w77, "Message Queue"=w64) -> ()  [unwired: 8 in]
      n696 = while {
        tunnel: w64 -> [w321]
        shift-right: [w326] -> w92
        shift-left: w91 -> [w327]
        tunnel: [w323] -> w90
        tunnel: w88 -> [w322]
        stop <- w324 stop-if-true
        # "Event Handling Loop"
        n697 = event "DQMH_EVENT_MAIN" shown="[11] <Tool Module Request Events.Get All Inspect Data>: User Event" {
          selector: w327 -> [_ _ _ _ _ _ _ _ _ _ _ _ _ _ _ _ _ _ _ _ _ _ _ _ _ _ _ _]
          dyn-events: [_ _ _ _ _ _ _ _ _ _ _ _ _ _ _ _ _ _ _ _ _ _ _ _ _ _ _ _] -> w326
          timeout: _ -> [_ _ _ _ _ _ _ _ _ _ _ _ _ _ _ _ _ _ _ _ _ _ _ _ _ _ _ _]
          tunnel: [_ _ _ _ _ _ _ TRUE ("Discard?") _ _ _ _ _ _ _ _ _ _ _ _ _ _ _ _ _ _ _ _] -> w324
          tunnel: w321 -> [_ w340 w343 _ _ _ _ w369 w372 w387 w394 w401 w410 w417 w424 w430 w437 w445 w452 w458 w464 w471 w479 w485 w492 w500 w507 w516]
          tunnel: [w329 w339 w341 _ _ w349 _ w364 w371 w383 w390 w397 w406 w413 w420 w426 w433 w441 w448 w454 w460 w467 w475 w481 w488 w496 w503 w512] -> w325
          tunnel: w322 -> [_ _ _ _ _ _ _ _ w374 _ _ _ _ _ _ _ _ _ _ _ _ _ _ _ _ _ _ _]
          event "Simulate EHL Error": Value Change {
            # "This case simulates an error being generated at the EHL"
            n698 = event-data() -> ()  [unwired: 1 in, 1 out]
            n699 = call "Module Name--constant.vi"() -> ("Module Name"=w328:string)  [unwired: 11 in]
            n700 = xnode "Error Ring"("parameter 0"=w328) -> ("error out"=w329:errorcluster)
          }
          event "Retrieve Cfg": Value Change {
            n701 = event-data() -> ()  [unwired: 1 in, 1 out]
            n702 = call-poly <vilib>:"Delacor_lib_QMH_Enqueue Message (poly).vi"("Message Data"=TRUE, "Message"="Connect: Retrieve Tool Config", "Message Queue in"=w340) -> ("error out"=w339:errorcluster)  [unwired: 7 in, 1 out]
          }
          event "Simulate MHL Error": Value Change {
            # "This case simulates an error being generated at the EHL"
            n703 = event-data() -> ()  [unwired: 1 in, 1 out]
            n704 = call-poly <vilib>:"Delacor_lib_QMH_Enqueue Message (poly).vi"("Message"="Simulate MHL Error", "Message Queue in"=w343) -> ("error out"=w341:errorcluster)  [unwired: 8 in, 1 out]
          }
          event User Event {
            # "Another Module called the \"Show Panel\" API Method."
            n705 = event-data() -> ()  [unwired: 1 in, 1 out]
            n706 = control-ref of="This VI"() -> (w345:refnum<vi>)
            n707 = call "Open VI Panel.vi"("VI in"=w345) -> ()  [unwired: 10 in, 1 out]
            n708 = call "Status Updated.vi"("Status"="Panel shown." ("format string")) -> ()  [unwired: 10 in, 1 out]
          }
          event User Event {
            # "Another Module called the \"Hide Panel\" API Method."
            n709 = event-data() -> ()  [unwired: 1 in, 1 out]
            n710 = control-ref of="This VI"() -> (w347:refnum<vi>)
            n711 = call "Hide VI Panel.vi"("VI in"=w347) -> ()  [unwired: 10 in, 1 out]
            n712 = call "Status Updated.vi"("Status"="Panel hidden." ("format string")) -> ()  [unwired: 10 in, 1 out]
          }
          event User Event {
            # "Another Module called the \"Get Module Execution Status\" API Method."
            n713 = event-data() -> ()  [unwired: 1 in, 1 out]
            n714 = call "Update Module Execution Status.vi"("Running?"=TRUE) -> ("error out"=w349:errorcluster)  [unwired: 10 in]
          }
          event User Event {
            # "Another Module called the \"Show Diagram\" API Method."
            n715 = event-data() -> ()  [unwired: 1 in, 1 out]
            n716 = disable-structure shown="RUN_TIME_ENGINE==False" {
              frame condition #0 (active) {
                # "functionality not available in exe"
                n717 = invoke on="Invoke Node" class="VI" method="Lock State.Get"() -> (error out=w355:errorcluster, "Get Lock State"=w354:T19, "pwd in cache"=w351:bool)  [unwired: 4 in, 1 out]
                n718 = Equal?(x=T19."Password-protected", y=w354) -> (x = y?=w352:bool)
                n719 = Compound Arithmetic op=AND(w352, invert w351) -> (w350:bool)
                n720 = case shown="False" w350 {
                  tunnel: w355 -> [w358 _]
                  frame False {
                    n721 = property on="Property Node" class="VI"(error in=w358, "BDWin.Open"=TRUE ("Block Diagram Window:Open")) -> ()  [unwired: 1 in, 2 out]
                    n722 = call "Status Updated.vi"("Status"="Block Diagram shown." ("format string")) -> ()  [unwired: 10 in, 1 out]
                  }
                  frame True {
                    # "Password-protected VI, and the password is not in the cache. Do not show the diagram."
                  }
                }
              }
              frame condition #1 {
              }
            }
          }
          event User Event {
            # "The Stop Module Event can get fired from the Exit message in the MHL. The queue gets destroyed in that case. If the queue no longer exists, the Enqueue Exit as a priority message will return error 1. It is safe to ignore, because the module is already exiting."
            # "Another Module called the \"Stop Module\" API Method  or the Message Handling Loop below."
            n723 = event-data() -> ("Origin"=w368:string, "Exit via Stop Module Req?"=w362:bool, "Wait for Module to stop?"=w361:bool)  [unwired: 1 in]
            n724 = local write "Status"(w368) -> ()
            n725 = Bundle By Name(cluster=T20 {"Origin"="", "Exit via Stop Module Req?"=FALSE, "Wait for Module to stop?"=FALSE} ("Stop Argument"), "Exit via Stop Module Req?"=w362, "Wait for Module to stop?"=w361) -> (w360:T20)
            n726 = call-poly <vilib>:"Delacor_lib_QMH_Enqueue Message (poly).vi"("Priority Message? (F)"=TRUE, "Message Data"=w360, "Message"="EXIT: Shutdown Tool", "Message Queue in"=w369) -> ("error out"=w365:errorcluster)  [unwired: 6 in, 1 out]
            n727 = call <vilib>:"Clear Errors.vi"("error in (no error)"=w365, "specific error code to clear (0: all)"=1) -> ("error out"=w364:errorcluster)  [unwired: 4 in, 1 out]
          }
          event Panel Close? {
            w375 = TRUE  # Discard the event so the 'Confirm Quit' message has a chance to run.
            # "Send the 'Confirm Quit' message if the user closes the panel of the VI."
            n728 = event-data() -> ()  [unwired: 1 in, 1 out]
            n729 = property on="Property Node" class="Module Admin"(reference=w374) -> ("Accessors:External Launch"=w373:bool)  [unwired: 1 in, 2 out]
            n730 = case shown="False" w373 {
              tunnel: w372 -> [_ w379]
              tunnel: [_ w380] -> w371
              frame True {
                # "If externally launched, clicking the 'X' hides the panel, but doesn't close it."
                n731 = control-ref of="This VI"() -> (w376:refnum<vi>)
                n732 = call "Hide VI Panel.vi"("VI in"=w376) -> ()  [unwired: 10 in, 1 out]
              }
              frame False {
                # "If run as a stand-alone VI, clicking the panel 'X' stops the VI."
                n733 = call-poly <vilib>:"Delacor_lib_QMH_Enqueue Message (poly).vi"("Priority Message? (F)"=TRUE, "Message"="EXIT: Shutdown Tool", "Message Queue in"=w379) -> ("error out"=w380:errorcluster)  [unwired: 7 in, 1 out]
              }
            }
            n734 = event-data ("Event Filter Node")("Discard?"=w375) -> ()  [unwired: 1 in, 1 out]
          }
          event User Event {
            # "<Tool Module Request Events.CONNECT>: User Event"
            n735 = event-data() -> ("Connect"=w382:bool)  [unwired: 1 in]
            n736 = Bundle(cluster=T21 {"Connect"=FALSE} ("CONNECT Argument"), "Connect"=w382) -> (w384:T21)
            n737 = call-poly <vilib>:"Delacor_lib_QMH_Enqueue Message (poly).vi"("Priority Message? (F)"=FALSE, "Message Data"=w384, "Message"="CONNECT", "Message Queue in"=w387) -> ("error out"=w383:errorcluster)  [unwired: 6 in, 1 out]
          }
          event User Event {
            # "<Tool Modle Request Events.GOTO>: User Event"
            n738 = event-data() -> ("GoTo Cmd"=w389:T23, "Data"=w388:i32)  [unwired: 1 in]
            n739 = Bundle(cluster=T22 {"GoTo Cmd"=enum."MoveA", "Data"=0} ("GOTO Argument"), "GoTo Cmd"=w389, "Data"=w388) -> (w391:T22)
            n740 = call-poly <vilib>:"Delacor_lib_QMH_Enqueue Message (poly).vi"("Message Data"=w391, "Message"="GOTO", "Message Queue in"=w394) -> ("error out"=w390:errorcluster)  [unwired: 7 in, 1 out]
          }
          event User Event {
            # "<Tool Module Request Events.Get All Inspect Data>: User Event"
            n741 = event-data() -> ("dummy"=w396:bool, "Wait Notifier"=w395:refnum<notifier>)  [unwired: 1 in]
            n742 = Bundle(cluster=T24 {"dummy"=FALSE, "Wait Notifier"=refnum} ("Get All Inspect Data Argument"), "dummy"=w396, "Wait Notifier"=w395) -> (w398:T24)
            n743 = call-poly <vilib>:"Delacor_lib_QMH_Enqueue Message (poly).vi"("Message Data"=w398, "Message"="Get All Inspect Data", "Message Queue in"=w401) -> ("error out"=w397:errorcluster)  [unwired: 7 in, 1 out]
          }
          event User Event {
            n744 = event-data() -> ("Monitor"=w404:bool, "Lasers ON?"=w403:bool, "Host Sample Data notifier"=w402:refnum<notifier>)  [unwired: 1 in]
            n745 = Bundle(cluster=T25 {"Monitor"=FALSE, "Lasers ON?"=FALSE, "Host Sample Data notifier"=refnum} ("Start Data Monitor Argument"), "Monitor"=w404, "Lasers ON?"=w403, "Host Sample Data notifier"=w402) -> (w407:T25)
            n746 = call-poly <vilib>:"Delacor_lib_QMH_Enqueue Message (poly).vi"("Priority Message? (F)"=TRUE, "Message Data"=w407, "Message"="MONITOR", "Message Queue in"=w410) -> ("error out"=w406:errorcluster)  [unwired: 6 in, 1 out]
          }
          event User Event {
            n747 = event-data() -> ("dummy"=w412:bool, "Wait Notifier"=w411:refnum<notifier>)  [unwired: 1 in]
            n748 = Bundle(cluster=T26 {"dummy"=FALSE, "Wait Notifier"=refnum} ("Get FPGA Setup Params Argument"), "dummy"=w412, "Wait Notifier"=w411) -> (w414:T26)
            n749 = call-poly <vilib>:"Delacor_lib_QMH_Enqueue Message (poly).vi"("Message Data"=w414, "Message"="Get FPGA Setup Params", "Message Queue in"=w417) -> ("error out"=w413:errorcluster)  [unwired: 7 in, 1 out]
          }
          event User Event {
            # "Another Module called the \"Set Cur FPGA Setup Params\" API Method."
            n750 = event-data() -> ("Commit"=w419:bool, "FPGA Setup Parameters"=w418:T28)  [unwired: 1 in]
            n751 = Bundle(cluster=T27 {"Commit"=FALSE, "FPGA Setup Parameters"={"FPGA Timing Constraints"={"frame.length Min"=530, "frame.ST_OFF Min"=15, "frame.ST_ON Min"=8, "frame.first data idx"=14, "frame.integ Offset"=6, "frame.integ Delay"=3, "frame.ad_latch Delay"=11, "frame.trig time Max"=0}, "FPGA Timing Ctrl"={"trig.time"=220, "integ.count 1"=400, "integ.count 2"=350, "encdr.latch ctrl"=1, "pixel.read count"=512, "clock.select"=2, "ad.clock offset"=16, "data.control reg"=2}, "FPGA Laser Config"={"laser.gain"=10, "laser.threshold Low"=1400, "laser.threshold High"=1900, "laser.dac init"=912, "laser.dac Min"=800, "laser.dac Max"=4000, "laser.config reg"=3}, "FPGA Peak Proc Cfg"={"PD.threshold"=0, "PD.width detect Min"=0, "PD.sensor pixels"=512, "PD.config reg"=23}, "FPGA SPI Cfg"={"SPI Divide Value"=1, "SPI config reg"=1}}} ("Set Cur FPGA Setup Params Argument"), "Commit"=w419, "FPGA Setup Parameters"=w418) -> (w421:T27)
            n752 = call-poly <vilib>:"Delacor_lib_QMH_Enqueue Message (poly).vi"("Message Data"=w421, "Message"="Set FPGA Setup Params", "Message Queue in"=w424) -> ("error out"=w420:errorcluster)  [unwired: 7 in, 1 out]
          }
          event User Event {
            # "Another Module called the \"Set Tool Config\" API Method."
            n753 = event-data() -> ("Tool Config Cluster"=w425:T35)  [unwired: 1 in]
            n754 = Bundle(cluster=T34 {"Tool Config Cluster"={"Tool Type"=0, "Tool SN"=0, "Tool Block"={"Encoder Size"=0, "Encoder Scale"=0, "Encoder Offset"=0, "MaxEncoder"=0, "MinEncoder"=0, "Start Delay"=0.0, "Tool Face Ref"=0.0}, "Motor Block"={"MinMotor Speed"=0, "MaxMotor Speed"=0, "Homing Speed"=90, "Jog Speed"=90, "Inspect Speed"=90, "VBlk Speed"=90, "CleaningPos"=0, "Safe Zone"=0, "Has Motor"=FALSE, "Use Home Index"=FALSE}, "Verification Block"={"Angle"=90.0, "FlankLength1"=0.0, "FlankLength2"=0.0, "Location"=0.0, "Serial Number"=0}, "Probe Block"={"nProbes"=0, "Probe Param Array"=[]}}} ("Set Tool Config Argument"), "Tool Config Cluster"=w425) -> (w427:T34)
            n755 = call-poly <vilib>:"Delacor_lib_QMH_Enqueue Message (poly).vi"("Message Data"=w427, "Message"="Commit Tool Config", "Message Queue in"=w430) -> ("error out"=w426:errorcluster)  [unwired: 7 in, 1 out]
          }
          event User Event {
            # "Another Module called the \"Set Integration Count\" API Method."
            n756 = event-data() -> ("Mode"=w432:i16, "Integ Count"=w431:u32)  [unwired: 1 in]
            n757 = Bundle(cluster=T42 {"Mode"=0, "Integ Count"=0} ("Set Integration Count Argument"), "Mode"=w432, "Integ Count"=w431) -> (w434:T42)
            n758 = call-poly <vilib>:"Delacor_lib_QMH_Enqueue Message (poly).vi"("Message Data"=w434, "Message"="Set Integration Count", "Message Queue in"=w437) -> ("error out"=w433:errorcluster)  [unwired: 7 in, 1 out]
          }
          event User Event {
            # "Another Module called the \"Set Laser Params\" API Method."
            n759 = event-data() -> ("Mode"=w440:i16, "Gain"=w439:u16, "Init DAC"=w438:u16)  [unwired: 1 in]
            n760 = Bundle(cluster=T43 {"Mode"=0, "Gain"=0, "Init DAC"=0} ("Set Laser Params Argument"), "Mode"=w440, "Gain"=w439, "Init DAC"=w438) -> (w442:T43)
            n761 = call-poly <vilib>:"Delacor_lib_QMH_Enqueue Message (poly).vi"("Message Data"=w442, "Message"="Set Laser Params", "Message Queue in"=w445) -> ("error out"=w441:errorcluster)  [unwired: 7 in, 1 out]
          }
          event User Event {
            # "Another Module called the \"Get Mtrl Ctrl Reg\" API Method."
            n762 = event-data() -> ("dummy"=w447:bool, "Wait Notifier"=w446:refnum<notifier>)  [unwired: 1 in]
            n763 = Bundle(cluster=T44 {"dummy"=FALSE, "Wait Notifier"=refnum} ("Get Mtrl Ctrl Reg Argument"), "dummy"=w447, "Wait Notifier"=w446) -> (w449:T44)
            n764 = call-poly <vilib>:"Delacor_lib_QMH_Enqueue Message (poly).vi"("Message Data"=w449, "Message"="Get Mtr Ctrl Reg", "Message Queue in"=w452) -> ("error out"=w448:errorcluster)  [unwired: 7 in, 1 out]
          }
          event User Event {
            # "Another Module called the \"Set Mtr Ctrl Reg\" API Method."
            n765 = event-data() -> ("Ctrl Reg"=w453:u16)  [unwired: 1 in]
            n766 = Bundle(cluster=T45 {"Ctrl Reg"=0} ("Set Mtr Ctrl Reg Argument"), "Ctrl Reg"=w453) -> (w455:T45)
            n767 = call-poly <vilib>:"Delacor_lib_QMH_Enqueue Message (poly).vi"("Message Data"=w455, "Message"="Commit Ctrl Reg", "Message Queue in"=w458) -> ("error out"=w454:errorcluster)  [unwired: 7 in, 1 out]
          }
          event User Event {
            # "Another Module called the \"Set Event Logger\" API Method."
            n768 = event-data() -> ("EventLog.lvclass"=w459:refnum<class "EventLog.lvclass">)  [unwired: 1 in]
            n769 = Bundle(cluster=T46 {"EventLog.lvclass"=refnum} ("Set Event Logger Argument"), "EventLog.lvclass"=w459) -> (w461:T46)
            n770 = call-poly <vilib>:"Delacor_lib_QMH_Enqueue Message (poly).vi"("Message Data"=w461, "Message"="Set Event Logger", "Message Queue in"=w464) -> ("error out"=w460:errorcluster)  [unwired: 7 in, 1 out]
          }
          event User Event {
            # "Another Module called the \"Write to File\" API Method."
            n771 = event-data() -> ("Filename"=w466:string, "Flattened data strings"=w465:string[])  [unwired: 1 in]
            n772 = Bundle(cluster=T47 {"Filename"="", "Flattened data strings"=[]} ("Write to File Argument"), "Filename"=w466, "Flattened data strings"=w465) -> (w468:T47)
            n773 = call-poly <vilib>:"Delacor_lib_QMH_Enqueue Message (poly).vi"("Message Data"=w468, "Message"="Write to File", "Message Queue in"=w471) -> ("error out"=w467:errorcluster)  [unwired: 7 in, 1 out]
          }
          event User Event {
            # "Another Module called the \"Read from File\" API Method."
            n774 = event-data() -> ("Filename"=w474:string, "Create?"=w473:bool, "Flattened Data Strings"=w472:string[])  [unwired: 1 in]
            n775 = Bundle(cluster=T48 {"Filename"="", "Create?"=FALSE, "Flattened Data Strings"=[]} ("Read from File Argument"), "Filename"=w474, "Create?"=w473, "Flattened Data Strings"=w472) -> (w476:T48)
            n776 = call-poly <vilib>:"Delacor_lib_QMH_Enqueue Message (poly).vi"("Message Data"=w476, "Message"="Read from File", "Message Queue in"=w479) -> ("error out"=w475:errorcluster)  [unwired: 7 in, 1 out]
          }
          event User Event {
            # "Another Module called the \"Set Device Temp Thresholds\" API Method."
            n777 = event-data() -> ("Device Temp Thold Arrays"=w480:T50)  [unwired: 1 in]
            n778 = Bundle(cluster=T49 {"Device Temp Thold Arrays"={"High Thold "=[], "Low Thold "=[]}} ("Set Device Temp Thresholds Argument"), "Device Temp Thold Arrays"=w480) -> (w482:T49)
            n779 = call-poly <vilib>:"Delacor_lib_QMH_Enqueue Message (poly).vi"("Message Data"=w482, "Message"="Set Device Temp Thresholds", "Message Queue in"=w485) -> ("error out"=w481:errorcluster)  [unwired: 7 in, 1 out]
          }
          event User Event {
            # "Another Module called the \"Get Cycle Count\" API Method."
            n780 = event-data() -> ("Clear?"=w487:bool, "Wait Notifier"=w486:refnum<notifier>)  [unwired: 1 in]
            n781 = Bundle(cluster=T51 {"Clear?"=FALSE, "Wait Notifier"=refnum} ("Get Cycle Count Argument"), "Clear?"=w487, "Wait Notifier"=w486) -> (w489:T51)
            n782 = call-poly <vilib>:"Delacor_lib_QMH_Enqueue Message (poly).vi"("Message Data"=w489, "Message"="Get Cycle Count", "Message Queue in"=w492) -> ("error out"=w488:errorcluster)  [unwired: 7 in, 1 out]
          }
          event User Event {
            # "Another Module called the \"Return FPGA Setup Data\" API Method."
            n783 = event-data() -> ("Reload"=w495:bool, "Wait Notifier"=w494:refnum<notifier>, "wait for reply"=w493:bool)  [unwired: 1 in]
            n784 = Bundle(cluster=T52 {"Reload"=FALSE, "Wait Notifier"=refnum, "wait for reply"=FALSE} ("Return FPGA Setup Data Argument"), "Reload"=w495, "Wait Notifier"=w494, "wait for reply"=w493) -> (w497:T52)
            n785 = call-poly <vilib>:"Delacor_lib_QMH_Enqueue Message (poly).vi"("Message Data"=w497, "Message"="Return FPGA Setup Data", "Message Queue in"=w500) -> ("error out"=w496:errorcluster)  [unwired: 7 in, 1 out]
          }
          event User Event {
            # "<Tool Module Request Events.Update FPGA Setup Data>:User Event"
            # "Another Module called the \"Update FPGA Setup Data\" API Method."
            n786 = event-data() -> ("Commit"=w502:bool, "FPGA Setup Parameters"=w501:T28)  [unwired: 1 in]
            n787 = Bundle(cluster=T53 {"Commit"=FALSE, "FPGA Setup Parameters"={"FPGA Timing Constraints"={"frame.length Min"=530, "frame.ST_OFF Min"=15, "frame.ST_ON Min"=8, "frame.first data idx"=14, "frame.integ Offset"=6, "frame.integ Delay"=3, "frame.ad_latch Delay"=11, "frame.trig time Max"=0}, "FPGA Timing Ctrl"={"trig.time"=220, "integ.count 1"=400, "integ.count 2"=350, "encdr.latch ctrl"=1, "pixel.read count"=512, "clock.select"=2, "ad.clock offset"=16, "data.control reg"=2}, "FPGA Laser Config"={"laser.gain"=10, "laser.threshold Low"=1400, "laser.threshold High"=1900, "laser.dac init"=912, "laser.dac Min"=800, "laser.dac Max"=4000, "laser.config reg"=3}, "FPGA Peak Proc Cfg"={"PD.threshold"=0, "PD.width detect Min"=0, "PD.sensor pixels"=512, "PD.config reg"=23}, "FPGA SPI Cfg"={"SPI Divide Value"=1, "SPI config reg"=1}}} ("Update FPGA Setup Data Argument"), "Commit"=w502, "FPGA Setup Parameters"=w501) -> (w504:T53)
            n788 = call-poly <vilib>:"Delacor_lib_QMH_Enqueue Message (poly).vi"("Message Data"=w504, "Message"="Update FPGA Setup Data", "Message Queue in"=w507) -> ("error out"=w503:errorcluster)  [unwired: 7 in, 1 out]
          }
          event User Event {
            # "Another Module called the \"Get-Set Inspection Limits\" API Method."
            n789 = event-data() -> ("Set"=w511:bool, "Inspection Limits"=w510:T11, "Wait Notifier"=w509:refnum<notifier>, "wait for reply"=w508:bool)  [unwired: 1 in]
            n790 = Bundle(cluster=T54 {"Set"=FALSE, "Inspection Limits"={"MaxSamples"=50800, "PosToStartScan"=50800, "PosToEndScan"=0, "ScanLength"=50800}, "Wait Notifier"=refnum, "wait for reply"=FALSE} ("Get-Set Inspection Limits Argument"), "Set"=w511, "Inspection Limits"=w510, "Wait Notifier"=w509, "wait for reply"=w508) -> (w513:T54)
            n791 = call-poly <vilib>:"Delacor_lib_QMH_Enqueue Message (poly).vi"("Message Data"=w513, "Message"="Get-Set Inspection Limits", "Message Queue in"=w516) -> ("error out"=w512:errorcluster)  [unwired: 7 in, 1 out]
          }
        }
        n792 = call-dynamic "Delacor_lib_QMH_Error Handler - Event Handling Loop.vi"("error in (no error)"=w325, "Message Queue in"=w321) -> ("dup error in"=w323:errorcluster)  [unwired: 8 in, 1 out]
      }
      n793 = call "Timer Helper Loop.vi"("Timer ID"=w78, "Setup Timer"=w76, "Stop Helper Loop"=w77, "Message Queue"=w64) -> ()  [unwired: 8 in]
      n794 = call "Timer Helper Loop.vi"("Timer ID"=w75, "Setup Timer"=w76, "Stop Helper Loop"=w77, "Message Queue"=w64) -> ()  [unwired: 8 in]
    }
    frame Error {
      # "Synchronize Caller Events.vi will inform Start Module.vi that the module has launched and will let the code calling Start Module.vi register for broadcasts and would permit the caller receive the broadcast that an error occurred at launch time."
      n795 = call "Synchronize Caller Events.vi"("Singleton Module Admin in"=w1940) -> ("error out"=w1937:errorcluster)  [unwired: 9 in, 1 out]
      n796 = call "Module Name--constant.vi"() -> ("Module Name"=w1943:string)  [unwired: 11 in]
      n797 = Format Into String(format string="An error occurred during initialization. %s is no longer running.", w1943) -> (resulting string=w1941:string)  [unwired: 2 in, 1 out]
      n798 = Merge Errors(w1939, w1937) -> (w1938:errorcluster)
      n799 = call "Error Reported.vi"("Additional Information"=w1941, "Error"=w1938) -> ()  [unwired: 9 in, 1 out]
    }
  }
  n800 = Merge Errors(w47, w57, w1, w2) -> (w51:errorcluster)
  n801 = call "Close Module.vi"("error in (no error)"=w51, "Module Admin in"=w58) -> ("error out"=w10:errorcluster, "External Launch"=w49:bool, "Module Admin out"=w52:refnum<class "Delacor_lib_QMH_Module Admin.lvclass">)  [unwired: 7 in]
  n802 = Unregister For Events(event registration refnum=w9, error in=w10) -> (error out=w8:errorcluster)
  n803 = Release Notifier(notifier=w7, error in (no error)=w8) -> (error out=w61:errorcluster)  [unwired: 1 in, 2 out]
  n804 = Unregister For Events(event registration refnum=w32, error in=w61) -> (error out=w27:errorcluster)
  n805 = Unregister For Events(event registration refnum=w25, error in=w27) -> (error out=w26:errorcluster)
  n806 = Unregister For Events(event registration refnum=w56, error in=w26) -> (error out=w50:errorcluster)
  "error out" <- w50
  n807 = case "External Launch?" shown="True" w49 {
    tunnel: w50 -> [_ w1945]
    frame False {
    }
    frame True {
      n808 = case shown="Error" w1945 {
        frame No Error {
          n809 = disable-structure shown="Default" {
            frame condition #0 {
              n810 = invoke class="VI" method="FP.Close"() -> ()  [unwired: 3 in, 3 out]
            }
            frame condition #1 (active) {
            }
          }
        }
        frame Error {
          n811 = invoke class="VI" method="FP.Open"("Activate"=TRUE ("Activate?")) -> ()  [unwired: 4 in, 5 out]
        }
      }
    }
  }
  n812 = local write "Module Admin"(w52) -> ()
